vi "Text control 2 v7.0_pump-specific.vi"() -> ()   [LabVIEW 2016]
panel:
  in  "Tab Control":enum32{"Main", "Other parameters"}(tab)
  out "Line running":i32
  out "Total lines":i32
  out "Path":path=path "C:/users/rlp38/09Apr2009LTtesting/test2.txt"
  out "I vs Vg":cluster{"Y data in":dbl[], "X data in":dbl[]}[](graph)
  out "Is max":dbl format="%.2e"
  out "Id max":dbl format="%.2e"
  out "Ig max":dbl format="%.2e"
  out "Imax vs time":cluster{"Y data in":dbl[], "X data in":dbl[]}[](graph)
  out "Imin vs time":cluster{"Y data in":dbl[], "X data in":dbl[]}[](graph)
  out "I vs Vd":cluster{"Y data in":dbl[], "X data in":dbl[]}[](graph)
  in  "Script":string="#-------------------------------------------------------\n# SPM pump cleaning script\n#\n# Version: 0.5\n# Author: Dimitrios Simatos\n# Last updated: 2018-01-05\n#-------------------------------------------------------\n# Description\n#\n# This script is designed to run the cleaning sequence of the SPM OEM pump.\n# This script needs to be run 4 times!\n#-------------------------------------------------------\n# Changes\n#\n# Placed initialization and hard stop commands in the beginning.\n#-------------------------------------------------------\n# Important points\n#\n# Never leave any liquid in the pump to dry after the experiments. If they dry, the residue may block the valve.\n# Always run the cleaning cycle after the experiments.\n# Use clockwise rotation when going up in valve port numbers and vice versa.\n#-------------------------------------------------------\n# Things to do before running the script\n#\n# Set time units to minutes.\n# Set filenames.\n# Replace the tubing, if necessary.\n#-------------------------------------------------------\n# Port connections\n#\n# Port 1: Waste\n# Port 2: Waste\n# Port 3: Various cleaning liquids\n# Port 4: Waste\n# Port 5: Waste\n# Port 6: Waste\n#\n# Between each of the 4 runs, the settings of Port 3 will change, according to the cleaning protocol.\n# The settings for Port 3 are:\n# 1st run: 1% v/v solution of sodium hypochlorite in ultrapure water\n# 2nd run: 0.1% w/v solution of sodium dodecyl sulfate in ultrapure water\n# 3rd run: Ultrapure water\n# 4th run: Waste (in air, not immersed in liquid)\n#-------------------------------------------------------\n# Cleaning protocol for the SPM OEM pump (from the manual)\n#\n# A cleaning procedure should be performed at the end of each day or in between two different experiments.\n# An effective cleaning can be performed in the following manner:\n# • Bleach solution to kill microorganisms\n# 1. Prepare a solution of 1% chlorine bleach and deionized water\n#    NOTE: Prepare a 1% v/v solution of sodium hypochlorite in deionized water\n# 2. Prepare a reservoir and place 1 tubing in the bleach solution and 5 tubings in a waste recipient\n# 3. Pick up the bleach solution through 1 port to entirely fill the syringe\n# 4. Sequentially output the syringe content through the remaining ports and throw it to the waste\n# 5. Repeat operation at least 2 times\n# • Detergent solution to remove debris\n# 1. Prepare a solution of 0.1% detergent and deionized water\n#    NOTE: Prepare a 0.1% w/v solution of sodium dodecyl sulfate in deionized water\n# 2. Move the tubing from the bleach solution reservoir and place it into a reservoir of detergent solution\n# 3. Pick up the detergent solution through 1 port to entirely fill the syringe\n# 4. Sequentially output the detergent solution through the remaining ports into the waste recipient\n# 5. Repeat operation at least 2 times\n# • Rinsing water to prepare the pump for your next experiment\n# 1. Move the tubing from the detergent solution reservoir and place it into a reservoir of deionized water\n# 2. Pick up the rinsing solution through 1 port to entirely fill the syringe\n# 3. Sequentially output the rinse water through the remaining ports into the waste recipient\n# 4. Repeat operation at least 2 times\n# • Replace the tubing, if necessary\n#-------------------------------------------------------\n# Pumping cycles and execution time\n#\n# Execution time for a single cycle: 6 x (1 min + 10 sec) = 7 minutes\n# Total execution time: 4 x 7 = 28 minutes\n# Since the script has to run 4 times, the cleaning lasts for: 4 x 28 = 112 minutes\n# Air must be the last to be pumped through the valve, to remove all liquids.\n# There are 4 pumping cycles. Each one draws a different liquid through port 3 and pumps it sequentially through ports 1,2,4,5,6.\n# During the sequential pumping, each port receives 200 ml of liquid (20% of the total syringe volume = 600 \"plunger units\")\n# The device must be disconnected from the port during the cleaning procedure.\n# All cycles are similar, except cycle 1 has the initialization command uncommented and the first report valve command commented.\n#-------------------------------------------------------\n# Volume of liquid needed\n#\n# Volume of liquid needed per cycle: 1 ml\n# Total volume of liquid needed per script run: 4 x 1 = 4 ml\n# Since the script has to run 4 times, the first 3 with different liquids, I need:\n# 4 ml of 1% v/v solution of sodium hypochlorite in ultrapure water\n# 4 ml of 0.1% w/v solution of sodium dodecyl sulfate in ultrapure water\n# 4 ml of ultrapure water\n#-------------------------------------------------------\n# Parameters\n#\n# Syringe size: 1 ml\n# Step resolution N = 0.01 mm\n# Drawing flow V = 300 pulses/second (6000 ul/min)\n# Pumping flow V = 300 pulses/second (6000 ul/min)\n#-------------------------------------------------------\n# Pump initialization\npump /1T #hard stop pump\npump /1ZR #initialize pump\n#-------------------------------------------------------\n# Cycle 1\n# Fill the syringe\npump /1Q #query pump\npump /1? #report absolute plunger position\n#pump /1?6 #report valve position\nwait-min 1 #wait 1 minute\npump /1N0R #set step resolution: 0.01 mm\npump /1Q #query pump\npump /1? #report absolute plunger position (the plunger should be at 0)\npump /1?6 #report valve position\nwait 1000 #wait 1 second\npump /1V300R #choose speed: 300 steps/s (6000 ul/min)\npump /1Q #query pump\nwait 1000 #wait 1 second\npump /1I3R #go to port 3, clockwise rotation\npump /1Q #query pump\npump /1?6 #report valve position\nwait 1000 #wait 1 second\npump /1A3000R #go to absolute position 3000 (= draw 1 ml)\nwait 30000 #wait 30 seconds\npump /1Q #query pump\npump /1? #report absolute plunger position (the plunger should have finished moving)\n#pump /1?6 #report valve position\n# The sequential pumping begins\n# Port 1\npump /1O1R #switch to port 1, counterclockwise rotation\npump /1Q #query pump\npump /1?6 #report valve position\npump /1A2400R #go to absolute position 2400 (= pump 200 ul)\npump /1Q #query pump\npump /1? #report absolute plunger position (the plunger should be moving to 0)\nwait-min 1 #wait 1 minute\npump /1? #report absolute plunger position (the plunger should have finished moving)\n# Port 2\npump /1I2R #switch to port 2, clockwise rotation\npump /1Q #query pump\npump /1?6 #report valve position\npump /1A1800R #go to absolute position 1800 (= pump 200 ul)\npump /1Q #query pump\npump /1? #report absolute plunger position (the plunger should be moving to 0)\nwait-min 1 #wait 1 minute\npump /1? #report absolute plunger position (the plunger should have finished moving)\n# Port 4\npump /1I4R #switch to port 4, clockwise rotation\npump /1Q #query pump\npump /1?6 #report valve position\npump /1A1200R #go to absolute position 1200 (= pump 200 ul)\npump /1Q #query pump\npump /1? #report absolute plunger position (the plunger should be moving to 0)\nwait-min 1 #wait 1 minute\npump /1? #report absolute plunger position (the plunger should have finished moving)\n# Port 5\npump /1I5R #switch to port 5, clockwise rotation\npump /1Q #query pump\npump /1?6 #report valve position\npump /1A600R #go to absolute position 600 (= pump 200 ul)\npump /1Q #query pump\npump /1? #report absolute plunger position (the plunger should be moving to 0)\nwait-min 1 #wait 1 minute\npump /1? #report absolute plunger position (the plunger should have finished moving)\n# Port 6\npump /1I6R #switch to port 6, clockwise rotation\npump /1Q #query pump\npump /1?6 #report valve position\npump /1A0R #go to absolute position 0 (= pump 200 ul)\npump /1Q #query pump\npump /1? #report absolute plunger position (the plunger should be moving to 0)\nwait-min 1 #wait 1 minute\npump /1? #report absolute plunger position (the plunger should have finished moving)\n#-------------------------------------------------------\n# Cycle 2\n# Fill the syringe\n#pump /1ZR #initialize pump\npump /1Q #query pump\npump /1? #report absolute plunger position\npump /1?6 #report valve position\nwait-min 1 #wait 1 minute\npump /1N0R #set step resolution: 0.01 mm\npump /1Q #query pump\npump /1? #report absolute plunger position (the plunger should be at 0)\npump /1?6 #report valve position\nwait 1000 #wait 1 second\npump /1V300R #choose speed: 300 steps/s (6000 ul/min)\npump /1Q #query pump\nwait 1000 #wait 1 second\npump /1O3R #go to port 3, counterclockwise rotation\npump /1Q #query pump\npump /1?6 #report valve position\nwait 1000 #wait 1 second\npump /1A3000R #go to absolute position 3000 (= draw 1 ml)\nwait 30000 #wait 30 seconds\npump /1Q #query pump\npump /1? #report absolute plunger position (the plunger should have finished moving)\n#pump /1?6 #report valve position\n# The sequential pumping begins\n# Port 1\npump /1O1R #switch to port 1, counterclockwise rotation\npump /1Q #query pump\npump /1?6 #report valve position\npump /1A2400R #go to absolute position 2400 (= pump 200 ul)\npump /1Q #query pump\npump /1? #report absolute plunger position (the plunger should be moving to 0)\nwait-min 1 #wait 1 minute\npump /1? #report absolute plunger position (the plunger should have finished moving)\n# Port 2\npump /1I2R #switch to port 2, clockwise rotation\npump /1Q #query pump\npump /1?6 #report valve position\npump /1A1800R #go to absolute position 1800 (= pump 200 ul)\npump /1Q #query pump\npump /1? #report absolute plunger position (the plunger should be moving to 0)\nwait-min 1 #wait 1 minute\npump /1? #report absolute plunger position (the plunger should have finished moving)\n# Port 4\npump /1I4R #switch to port 4, clockwise rotation\npump /1Q #query pump\npump /1?6 #report valve position\npump /1A1200R #go to absolute position 1200 (= pump 200 ul)\npump /1Q #query pump\npump /1? #report absolute plunger position (the plunger should be moving to 0)\nwait-min 1 #wait 1 minute\npump /1? #report absolute plunger position (the plunger should have finished moving)\n# Port 5\npump /1I5R #switch to port 5, clockwise rotation\npump /1Q #query pump\npump /1?6 #report valve position\npump /1A600R #go to absolute position 600 (= pump 200 ul)\npump /1Q #query pump\npump /1? #report absolute plunger position (the plunger should be moving to 0)\nwait-min 1 #wait 1 minute\npump /1? #report absolute plunger position (the plunger should have finished moving)\n# Port 6\npump /1I6R #switch to port 6, clockwise rotation\npump /1Q #query pump\npump /1?6 #report valve position\npump /1A0R #go to absolute position 0 (= pump 200 ul)\npump /1Q #query pump\npump /1? #report absolute plunger position (the plunger should be moving to 0)\nwait-min 1 #wait 1 minute\npump /1? #report absolute plunger position (the plunger should have finished moving)\n#-------------------------------------------------------\n# Cycle 3\n# Fill the syringe\n#pump /1ZR #initialize pump\npump /1Q #query pump\npump /1? #report absolute plunger position\npump /1?6 #report valve position\nwait-min 1 #wait 1 minute\npump /1N0R #set step resolution: 0.01 mm\npump /1Q #query pump\npump /1? #report absolute plunger position (the plunger should be at 0)\npump /1?6 #report valve position\nwait 1000 #wait 1 second\npump /1V300R #choose speed: 300 steps/s (6000 ul/min)\npump /1Q #query pump\nwait 1000 #wait 1 second\npump /1O3R #go to port 3, counterclockwise rotation\npump /1Q #query pump\npump /1?6 #report valve position\nwait 1000 #wait 1 second\npump /1A3000R #go to absolute position 3000 (= draw 1 ml)\nwait 30000 #wait 30 seconds\npump /1Q #query pump\npump /1? #report absolute plunger position (the plunger should have finished moving)\n#pump /1?6 #report valve position\n# The sequential pumping begins\n# Port 1\npump /1O1R #switch to port 1, counterclockwise rotation\npump /1Q #query pump\npump /1?6 #report valve position\npump /1A2400R #go to absolute position 2400 (= pump 200 ul)\npump /1Q #query pump\npump /1? #report absolute plunger position (the plunger should be moving to 0)\nwait-min 1 #wait 1 minute\npump /1? #report absolute plunger position (the plunger should have finished moving)\n# Port 2\npump /1I2R #switch to port 2, clockwise rotation\npump /1Q #query pump\npump /1?6 #report valve position\npump /1A1800R #go to absolute position 1800 (= pump 200 ul)\npump /1Q #query pump\npump /1? #report absolute plunger position (the plunger should be moving to 0)\nwait-min 1 #wait 1 minute\npump /1? #report absolute plunger position (the plunger should have finished moving)\n# Port 4\npump /1I4R #switch to port 4, clockwise rotation\npump /1Q #query pump\npump /1?6 #report valve position\npump /1A1200R #go to absolute position 1200 (= pump 200 ul)\npump /1Q #query pump\npump /1? #report absolute plunger position (the plunger should be moving to 0)\nwait-min 1 #wait 1 minute\npump /1? #report absolute plunger position (the plunger should have finished moving)\n# Port 5\npump /1I5R #switch to port 5, clockwise rotation\npump /1Q #query pump\npump /1?6 #report valve position\npump /1A600R #go to absolute position 600 (= pump 200 ul)\npump /1Q #query pump\npump /1? #report absolute plunger position (the plunger should be moving to 0)\nwait-min 1 #wait 1 minute\npump /1? #report absolute plunger position (the plunger should have finished moving)\n# Port 6\npump /1I6R #switch to port 6, clockwise rotation\npump /1Q #query pump\npump /1?6 #report valve position\npump /1A0R #go to absolute position 0 (= pump 200 ul)\npump /1Q #query pump\npump /1? #report absolute plunger position (the plunger should be moving to 0)\nwait-min 1 #wait 1 minute\npump /1? #report absolute plunger position (the plunger should have finished moving)\n#-------------------------------------------------------\n# Cycle 4\n# Fill the syringe\n#pump /1ZR #initialize pump\npump /1Q #query pump\npump /1? #report absolute plunger position\npump /1?6 #report valve position\nwait-min 1 #wait 1 minute\npump /1N0R #set step resolution: 0.01 mm\npump /1Q #query pump\npump /1? #report absolute plunger position (the plunger should be at 0)\npump /1?6 #report valve position\nwait 1000 #wait 1 second\npump /1V300R #choose speed: 300 steps/s (6000 ul/min)\npump /1Q #query pump\nwait 1000 #wait 1 second\npump /1O3R #go to port 3, counterclockwise rotation\npump /1Q #query pump\npump /1?6 #report valve position\nwait 1000 #wait 1 second\npump /1A3000R #go to absolute position 3000 (= draw 1 ml)\nwait 30000 #wait 30 seconds\npump /1Q #query pump\npump /1? #report absolute plunger position (the plunger should have finished moving)\n#pump /1?6 #report valve position\n# The sequential pumping begins\n# Port 1\npump /1O1R #switch to port 1, counterclockwise rotation\npump /1Q #query pump\npump /1?6 #report valve position\npump /1A2400R #go to absolute position 2400 (= pump 200 ul)\npump /1Q #query pump\npump /1? #report absolute plunger position (the plunger should be moving to 0)\nwait-min 1 #wait 1 minute\npump /1? #report absolute plunger position (the plunger should have finished moving)\n# Port 2\npump /1I2R #switch to port 2, clockwise rotation\npump /1Q #query pump\npump /1?6 #report valve position\npump /1A1800R #go to absolute position 1800 (= pump 200 ul)\npump /1Q #query pump\npump /1? #report absolute plunger position (the plunger should be moving to 0)\nwait-min 1 #wait 1 minute\npump /1? #report absolute plunger position (the plunger should have finished moving)\n# Port 4\npump /1I4R #switch to port 4, clockwise rotation\npump /1Q #query pump\npump /1?6 #report valve position\npump /1A1200R #go to absolute position 1200 (= pump 200 ul)\npump /1Q #query pump\npump /1? #report absolute plunger position (the plunger should be moving to 0)\nwait-min 1 #wait 1 minute\npump /1? #report absolute plunger position (the plunger should have finished moving)\n# Port 5\npump /1I5R #switch to port 5, clockwise rotation\npump /1Q #query pump\npump /1?6 #report valve position\npump /1A600R #go to absolute position 600 (= pump 200 ul)\npump /1Q #query pump\npump /1? #report absolute plunger position (the plunger should be moving to 0)\nwait-min 1 #wait 1 minute\npump /1? #report absolute plunger position (the plunger should have finished moving)\n# Port 6\npump /1I6R #switch to port 6, clockwise rotation\npump /1Q #query pump\npump /1?6 #report valve position\npump /1A0R #go to absolute position 0 (= pump 200 ul)\npump /1Q #query pump\npump /1? #report absolute plunger position (the plunger should be moving to 0)\nwait-min 1 #wait 1 minute\npump /1? #report absolute plunger position (the plunger should have finished moving)\n#-------------------------------------------------------"
  out "Command running:":string
  out "Serial port data":string
  out "Elapsed Time":dbl caption="Elapsed Time (s)"
  in  "Time Units":u16(ring)=1 items=["Seconds", "Minutes", "Hours"]
  in  "Time Offset":dbl caption="Set Start Time (s)"
  in  "Reset":bool
  in  "Auto Reset":bool
  in  "integration time":u32(slide) max=2 step=1 scale=0.0..2.0
  in  "Interrupt scan":bool
  out "Absolute plunger position vs time":cluster{"Y data in":dbl[], "X data in":dbl[]}[](graph)
  out "Valve position vs time":cluster{"Y data in":dbl[], "X data in":dbl[]}[](graph)
  out "Is on":dbl format="%.2e"
  out "Id on":dbl format="%.2e"
  out "Ig on":dbl format="%.2e"
  out "Ion vs time":cluster{"Y data in":dbl[], "X data in":dbl[]}[](graph)
  out "Ioff vs time":cluster{"Y data in":dbl[], "X data in":dbl[]}[](graph)
  out "Ig min":dbl format="%.2e"
  out "Id min":dbl format="%.2e"
  out "Is min":dbl format="%.2e"
  out "Is off":dbl format="%.2e"
  out "Id off":dbl format="%.2e"
  out "Ig off":dbl format="%.2e"
  in  "Integration time (long)":dbl=0.32 min=0.04 max=2.0 step=0.02 format="%.2f"
  in  "Integration time (short)":dbl=0.0019 min=8e-05 max=0.0019 step=8e-05 format="%^.0e"
  in  "Gate: Compliance":dbl=0.001 format="%.8f"
  in  "Drain: Compliance":dbl=0.001 format="%.8f"
  in  "Hard stop pump":bool
  in  "Halt pump":bool
  in  "Interrupt program":bool
  in  "Suffix (script)":string="step_1_up-H2O_initial_script.txt"
  in  "Filename (variable part)":string="step_1_up-H2O_initial_"
  in  "Plot output curve extrema vs time":bool
  in  "Plot transfer curve extrema vs time":bool=TRUE
  in  "Plot sample extrema vs time":bool
  out "I vs time (Bias Stress)":cluster{"Y data in":dbl[], "X data in":dbl[]}[](graph)
  in  "Sample I - Probe 4 (Disabled)":u32(ring)=3 items=["SMU1  ", "SMU2  ", "SMU3  ", "SMU4  ", "SMU5  ", "SMU6  "]
  in  "Sample I - Source/Common":u32(ring) items=["SMU1  ", "SMU2  ", "SMU3  ", "SMU4  ", "SMU5  ", "SMU6  "]
  in  "Sample I - Probe 3 (Disabled)":u32(ring)=2 items=["SMU1  ", "SMU2  ", "SMU3  ", "SMU4  ", "SMU5  ", "SMU6  "]
  in  "Sample I - Drain/Gate":u32(ring)=1 items=["SMU1  ", "SMU2  ", "SMU3  ", "SMU4  ", "SMU5  ", "SMU6  "]
  in  "Sample - Probe 4":u32(ring)=3 items=["SMU1  ", "SMU2  ", "SMU3  ", "SMU4  ", "SMU5  ", "SMU6  "]
  in  "Sample - Source/Common":u32(ring) items=["SMU1  ", "SMU2  ", "SMU3  ", "SMU4  ", "SMU5  ", "SMU6  "]
  in  "Sample - Gate":u32(ring)=2 items=["SMU1  ", "SMU2  ", "SMU3  ", "SMU4  ", "SMU5  ", "SMU6  "]
  in  "Sample - Drain":u32(ring)=1 items=["SMU1  ", "SMU2  ", "SMU3  ", "SMU4  ", "SMU5  ", "SMU6  "]
  in  "VSU2 Stress - Source/Common":u32(ring) items=["SMU1  ", "SMU2  ", "SMU3  ", "SMU4  ", "SMU5  ", "SMU6  "]
  in  "Stress I - Source/Common":u32(ring) items=["SMU1  ", "SMU2  ", "SMU3  ", "SMU4  ", "SMU5  ", "SMU6  "]
  in  "Stress I - Drain/Gate":u32(ring)=1 items=["SMU1  ", "SMU2  ", "SMU3  ", "SMU4  ", "SMU5  ", "SMU6  "]
  in  "Stress V - Source/Common":u32(ring) items=["SMU1  ", "SMU2  ", "SMU3  ", "SMU4  ", "SMU5  ", "SMU6  "]
  in  "Stress V - Gate":u32(ring)=2 items=["SMU1  ", "SMU2  ", "SMU3  ", "SMU4  ", "SMU5  ", "SMU6  "]
  in  "Stress V - Drain":u32(ring)=1 items=["SMU1  ", "SMU2  ", "SMU3  ", "SMU4  ", "SMU5  ", "SMU6  "]
  in  "FPP - Source":u32(ring) items=["VSU1  ", "VSU2  "]
  in  "FPP - Probe 2":u32(ring)=3 items=["SMU1  ", "SMU2  ", "SMU3  ", "SMU4  ", "SMU5  ", "SMU6  "]
  in  "FPP - Probe 1":u32(ring) items=["SMU1  ", "SMU2  ", "SMU3  ", "SMU4  ", "SMU5  ", "SMU6  "]
  in  "FPP - Gate":u32(ring)=2 items=["SMU1  ", "SMU2  ", "SMU3  ", "SMU4  ", "SMU5  ", "SMU6  "]
  in  "FPP - Drain":u32(ring)=1 items=["SMU1  ", "SMU2  ", "SMU3  ", "SMU4  ", "SMU5  ", "SMU6  "]
  in  "Pulsed Stress V - Vextra":u32(ring)=1 items=["VSU1  ", "VSU2  "]
  in  "Pulsed Stress V - Probe 4":u32(ring)=3 items=["SMU1  ", "SMU2  ", "SMU3  ", "SMU4  ", "SMU5  ", "SMU6  "]
  in  "Pulsed Stress V - Source/Common":u32(ring) items=["SMU1  ", "SMU2  ", "SMU3  ", "SMU4  ", "SMU5  ", "SMU6  "]
  in  "Pulsed Stress V - Gate":u32(ring)=2 items=["SMU1  ", "SMU2  ", "SMU3  ", "SMU4  ", "SMU5  ", "SMU6  "]
  in  "Pulsed Stress V - Drain":u32(ring)=1 items=["SMU1  ", "SMU2  ", "SMU3  ", "SMU4  ", "SMU5  ", "SMU6  "]
  in  "Transfer/Output - Probe 4":u32(ring)=3 items=["SMU1  ", "SMU2  ", "SMU3  ", "SMU4  ", "SMU5  ", "SMU6  "]
  in  "Transfer/Output - Source/Common":u32(ring) items=["SMU1  ", "SMU2  ", "SMU3  ", "SMU4  ", "SMU5  ", "SMU6  "]
  in  "Transfer/Output - Gate":u32(ring)=2 items=["SMU1  ", "SMU2  ", "SMU3  ", "SMU4  ", "SMU5  ", "SMU6  "]
  in  "Transfer/Output - Drain":u32(ring)=1 items=["SMU1  ", "SMU2  ", "SMU3  ", "SMU4  ", "SMU5  ", "SMU6  "]
  in  "Gate Range\nmode":u16(ring) items=["Auto", "Limited", "Fixed"]
  in  "Gate Range":u8(slide)=3 max=11 scale=0.0..11.0
  in  "Source/Drain\nRange mode":u16(ring) items=["Auto", "Limited", "Fixed"]
  in  "Source/Drain Range":u8(slide)=3 max=11 scale=0.0..11.0
  in  "Panel Controls":T1={"Emergency Stop"=refnum, "TransGraph Max"=1e-05, "Text/Graph (text=false)"=TRUE} {"TransGraph Max" format="%.2e"}
  in  "Panel Controls 2":T2={"Emergency Stop"=refnum, "TransGraph Max"=1e-05, "Text/Graph (text=false)"=TRUE, "TransGraph Min"=1e-11} {"TransGraph Min" format="%.2e"; "TransGraph Max" format="%.2e"}
  in  "Probe 4":cluster{"on/off":bool, "Voltage":dbl} {"Voltage" min=-100.0 max=100.0 format="%.2f"}
  in  "Full Reset":bool
  in  "Standby":T3
  out "error out":errorcluster
  in  "Delay before read (ms)":u32=1000
  in  "byte count":u32=64
  in  "Serial End Mode for Reads":u16(ring)=2 items=["None", "LastBit", "TermChar"]
  in  "Timeout (ms)":u32=10000
  in  "Enable Termination\nChar (T)":bool=TRUE
  in  "Termination char\n(0xA = '\\n' = LF)\n(0xD = '\\r' = CR)":u8=13 format="%.0x"
  in  "flow control":u16(ring) items=["None"=0, "XON/XOFF"=1, "RTS/CTS"=2, "DTR/DSR"=4]
  in  "stop bits":u16(ring)=10 items=["1.0"=10, "1.5"=15, "2.0"=20]
  in  "parity":u16(ring) items=["None", "Odd", "Even", "Mark", "Space"]
  in  "data bits":u16=8 min=5 max=8 step=1
  in  "VISA resource name":refnum<visa-resource-name>="COM6"
  in  "baud rate":u32=9600
  out "Timings Indicator":T4 {"integration time" scale=0.0..2.0}
  in  "Timings (overwritten by the Front Panel)":T5={"integration time"=0, "Short/Long integration time"=0.00064, "hold time (sec)"=0.0, "delay time (sec)"=0.0, "Step Time (0 disables)"=0.0, "sweep method"=0, "Pulse period"=0.005, "Base voltage"=0.0, "Pulse width"=0.0005} {"Pulse width" min=0.0005 max=0.1 step=0.0001 format="%.4f"; "Base voltage" format="%^.4e"; "Pulse period" min=0.005 max=1.0 step=0.0001 format="%.4f"; "sweep method" items=["Continuous", "Pulsed"]; "Step Time (0 disables)" format="%.2f"; "delay time (sec)" format="%.4f"; "hold time (sec)" format="%.4f"; "Short/Long integration time" format="%^.0e"; "integration time" scale=0.0..2.0}
  out "Probe 4 Indicator":cluster{"on/off":bool, "Voltage":dbl} {"Voltage" min=-100.0 max=100.0 format="%.2f"}
  in  "VISA resource name in":refnum<visa-resource-name>="GPIB0::14::INSTR"
  in  "Gate":T6={"Gate Start"=0.0, "Gate Stop"=2.0, "Gate Step (linear only)"=1.0, "Gate Compliance"=0.0001, "Gate PComp"=0.0, "Range mode"=0, "Range"=6} {"Range" max=11 scale=0.0..11.0; "Range mode" items=["Auto", "Limited", "Fixed"]; "Gate PComp" format="%^.2e"; "Gate Compliance" format="%^.2e"; "Gate Step (linear only)" format="%^.4e"; "Gate Stop" format="%^.4e"; "Gate Start" format="%^.4e"}
  in  "Drain 2":T7={"Drain Start"=0.0, "Drain Stop"=2.0, "Drain Compliance"=0.0001, "Drain Step"=1.0, "Drain PComp"=0.0, "Range mode"=0, "Range"=6} {"Range" max=11 scale=0.0..11.0; "Range mode" items=["Auto", "Limited", "Fixed"]; "Drain PComp" format="%^.2e"; "Drain Step" format="%^.4e"; "Drain Compliance" format="%^.2e"; "Drain Stop" format="%^.4e"; "Drain Start" format="%^.4e"}
  # "Syntax:\nitime [s|m|l] time(sec): [s|m|l] determines the integration time setting (small|medium|long) and time sets the value.\nNOTE: The value of the integration time has to be within the range allowed by its category (s|m|l), otherwise, the closest value will be used. (e.g. if the category is set to short but the time value is very long, the actual value used will be the maximum short integration time.\nIntegration times:\n    Short: Default: 640 us. Range: 8E-5 - 1.92E-3 seconds.\n    Medium: Fixed at 1 NPL cycle (0.02 seconds).\n    Long: Default: 16 NPL cycles (0.32 seconds). Range: 2-100 NPL cycles (0.04 seconds - 2 seconds).\ngaterangemode [a|l|f]\ndrainrangemode [a|l|f]\npulsed [on|off] PulsePeriod(sec) PulseBaseVoltage PulseONWidth(sec)\nstandby [on l off]\nwait NumMilliseconds\nwait-min NumMinutes\n# texthere = comment\nProbe4 [ON|OFF] Voltage\ntransfer [s|d] VgStart VgStop VgStep VdStart VdStop VdStep\noutput [s|d] VgStart VgStop VgStep VdStart VdStop VdStep\nsample Vg Vd NumSamples Time(s) SampleInterval(s)\nsamplei Idg NumSamples Time(s) SampleInterval(s) VDGcompliance\n100 samples is approximately 13 seconds with medium integration\n# If in doubt use SampleInterval(s) = 0.004\n    NOTE: When doing bias stress measurements, it is best to set the Time Units to \"Seconds\", as the \"sample\" command has been configured to give the output to seconds.\nstressV VG VD IGcompliance IDcompliance Duration(sec)\nstressI IDG VDGcompliance Duration(sec)\nvsu2pulse Bias Duration(s)\npulsedstressV [s|d] VEstop VgON VgOFF Period(s) PulseONwidth(s) Vd\nsample-fpp Vg Vd NumSamples Time\nresample-fpp Vg Vd\ntransfer-fpp [s|d] VgStart VgStop VgStep VdStart VdStop VdStep\noutput-fpp [s|d] VgStart VgStop VgStep VdStart VdStop VdStep\nserial SerialPortCommand\npump SerialPortCommand for the SPM pump\n\nSPM Pump Syntax (<x>: pump number, use 1 if only one pump):\nif the command syntax contains [R], then append the letter R to the command\n/<x>Q: query (a query command should follow each command)\n/<x>Z[R] or /<x>Y[R]: initialize pump\n/<x>N<n>[R] (<n>=0,1): <0> (<1>) microstep 0.01 mm (0.00125 mm) resolution\n/<x>I<n> (<n>=0-6): turn to port number n (clockwise)\n/<x>O<n> (<n>=0-6): turn to port number n (counterclockwise)\n/<x>X: Re-execute last command string\n/<x>G<n>[R] (<n>=0-60000): repeat command sequence (default: 0, 0=loop forever)\n/<x>g: Mark the start of a repeat sequence (max = 10)\n/<x>M<n>[R] (<n>=0-86400000): delay command execution by n milliseconds\n/<x>H: Halt; Pause the sequence after finishing the current move\n/<x>T: Hardstop; Interrupt the current move and suppress it from the sequence\n/<x>A<n>[R] (<n>=0-3000 with N=0, 0-24000 with N=1): absolute position\n/<x>P<n>[R] (<n>=0-3000 with N=0, 0-24000 with N=1): relative pickup\n/<x>D<n>[R] (<n>=0-3000 with N=0, 0-24000 with N=1): relative dispense\n/<x>V<n>[R] (<n>=1-1600 default: 150): set peak speed (pulses/sec)\nNOTE: The lowest speed limit is 1 pulse/sec, not 5, as the manual states.\n/<x>S<n>[R] (<n>=10-40 default: 22): set speed (NOT in pulses/sec, look in manual)\nNOTE: When controlled with absolute position, one does not need to pay special attention to the syringe that is mounted on the pump.\nWithdraw from lower stage (ports 3, 5), dispense from higher stage (ports 2, 4, 6).\nConnect Port 1 to waste."
  # "Time"
  # "1\n2\n3\n4\n5\n6\n7\n8\n9\n10\n11\n12\n13\n14\n15\n16\n17\n18\n19\n20"
  # "Serial port settings"
  # "SMUs"
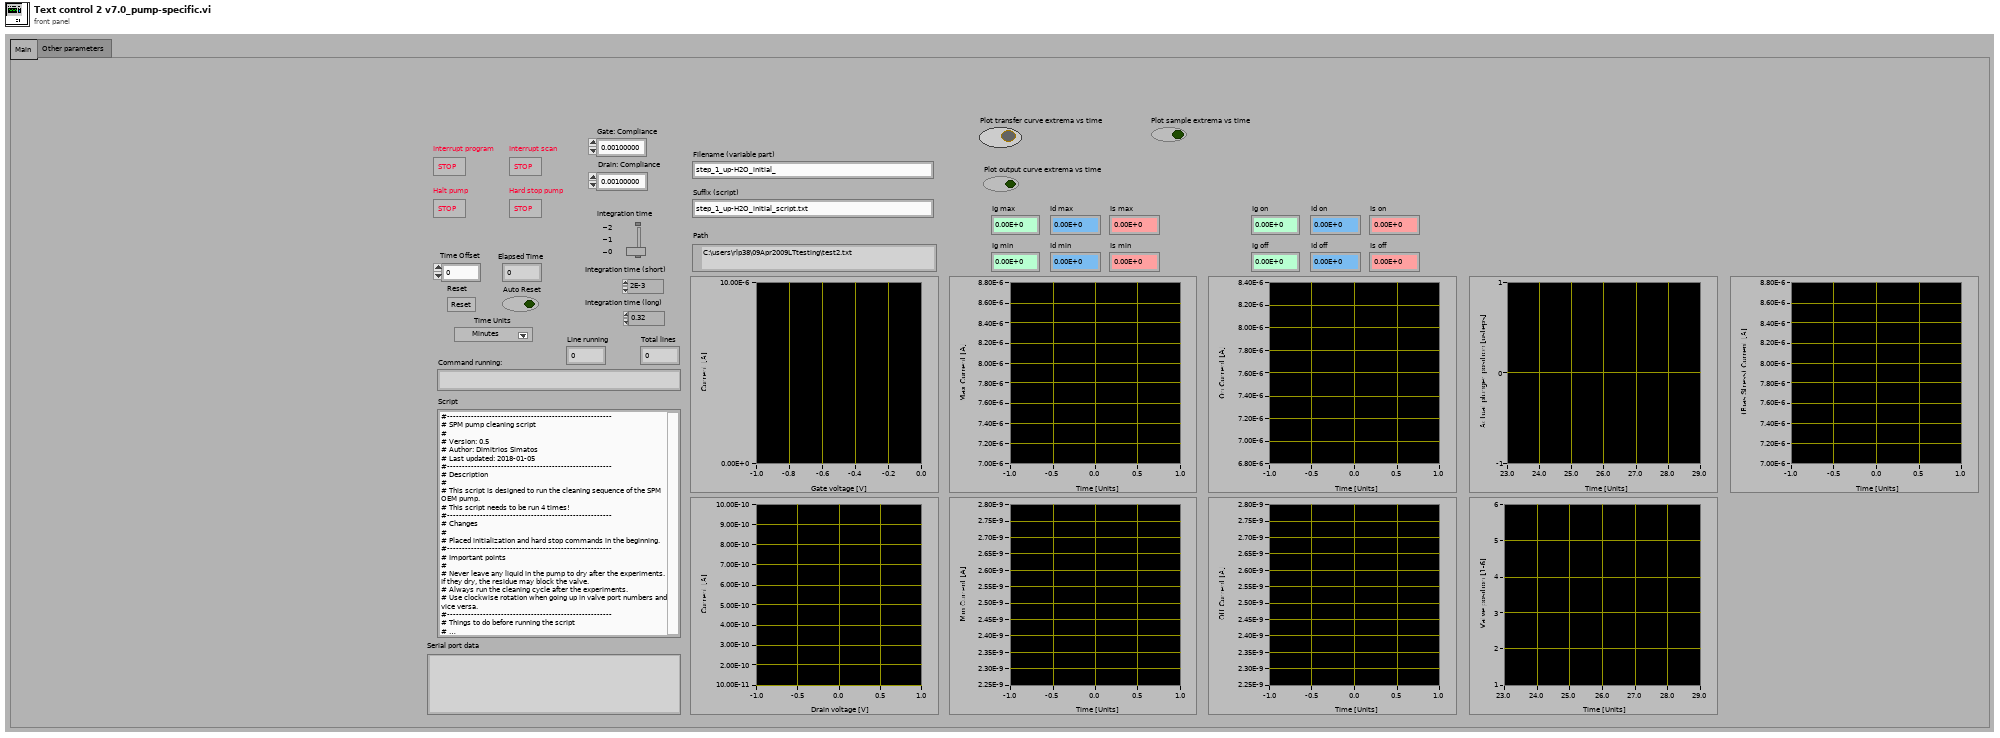
[diagram p1: front panel]
types:
  T1 = cluster{"Emergency Stop":refnum<vi>, "TransGraph Max":dbl, "Text/Graph (text=false)":bool}
  T2 = cluster{"Emergency Stop":refnum<vi>, "TransGraph Max":dbl, "Text/Graph (text=false)":bool, "TransGraph Min":dbl}
  T3 = cluster{"Gate Standby":bool, "Drain Standby":bool}
  T4 = cluster{"Short/Long integration time":dbl, "hold time (sec)":dbl, "delay time (sec)":dbl, "Step Time (0 disables)":dbl, "sweep method":u16, "Pulse period":dbl, "Base voltage":dbl, "Pulse width":dbl, "integration time":u32}
  T5 = cluster{"integration time":u32, "Short/Long integration time":dbl, "hold time (sec)":dbl, "delay time (sec)":dbl, "Step Time (0 disables)":dbl, "sweep method":u16, "Pulse period":dbl, "Base voltage":dbl, "Pulse width":dbl}
  T6 = cluster{"Gate Start":dbl, "Gate Stop":dbl, "Gate Step (linear only)":dbl, "Gate Compliance":dbl, "Gate PComp":dbl, "Range mode":u16, "Range":u8}
  T7 = cluster{"Drain Start":dbl, "Drain Stop":dbl, "Drain Compliance":dbl, "Drain Step":dbl, "Drain PComp":dbl, "Range mode":u16, "Range":u8}
  T8 = enum16{"open", "replace", "create", "open or create", "replace or create", "replace or create with confirmation"}
  T9 = cluster{"V2 Start":dbl, "V2 Step":dbl, "Number of points":i32}
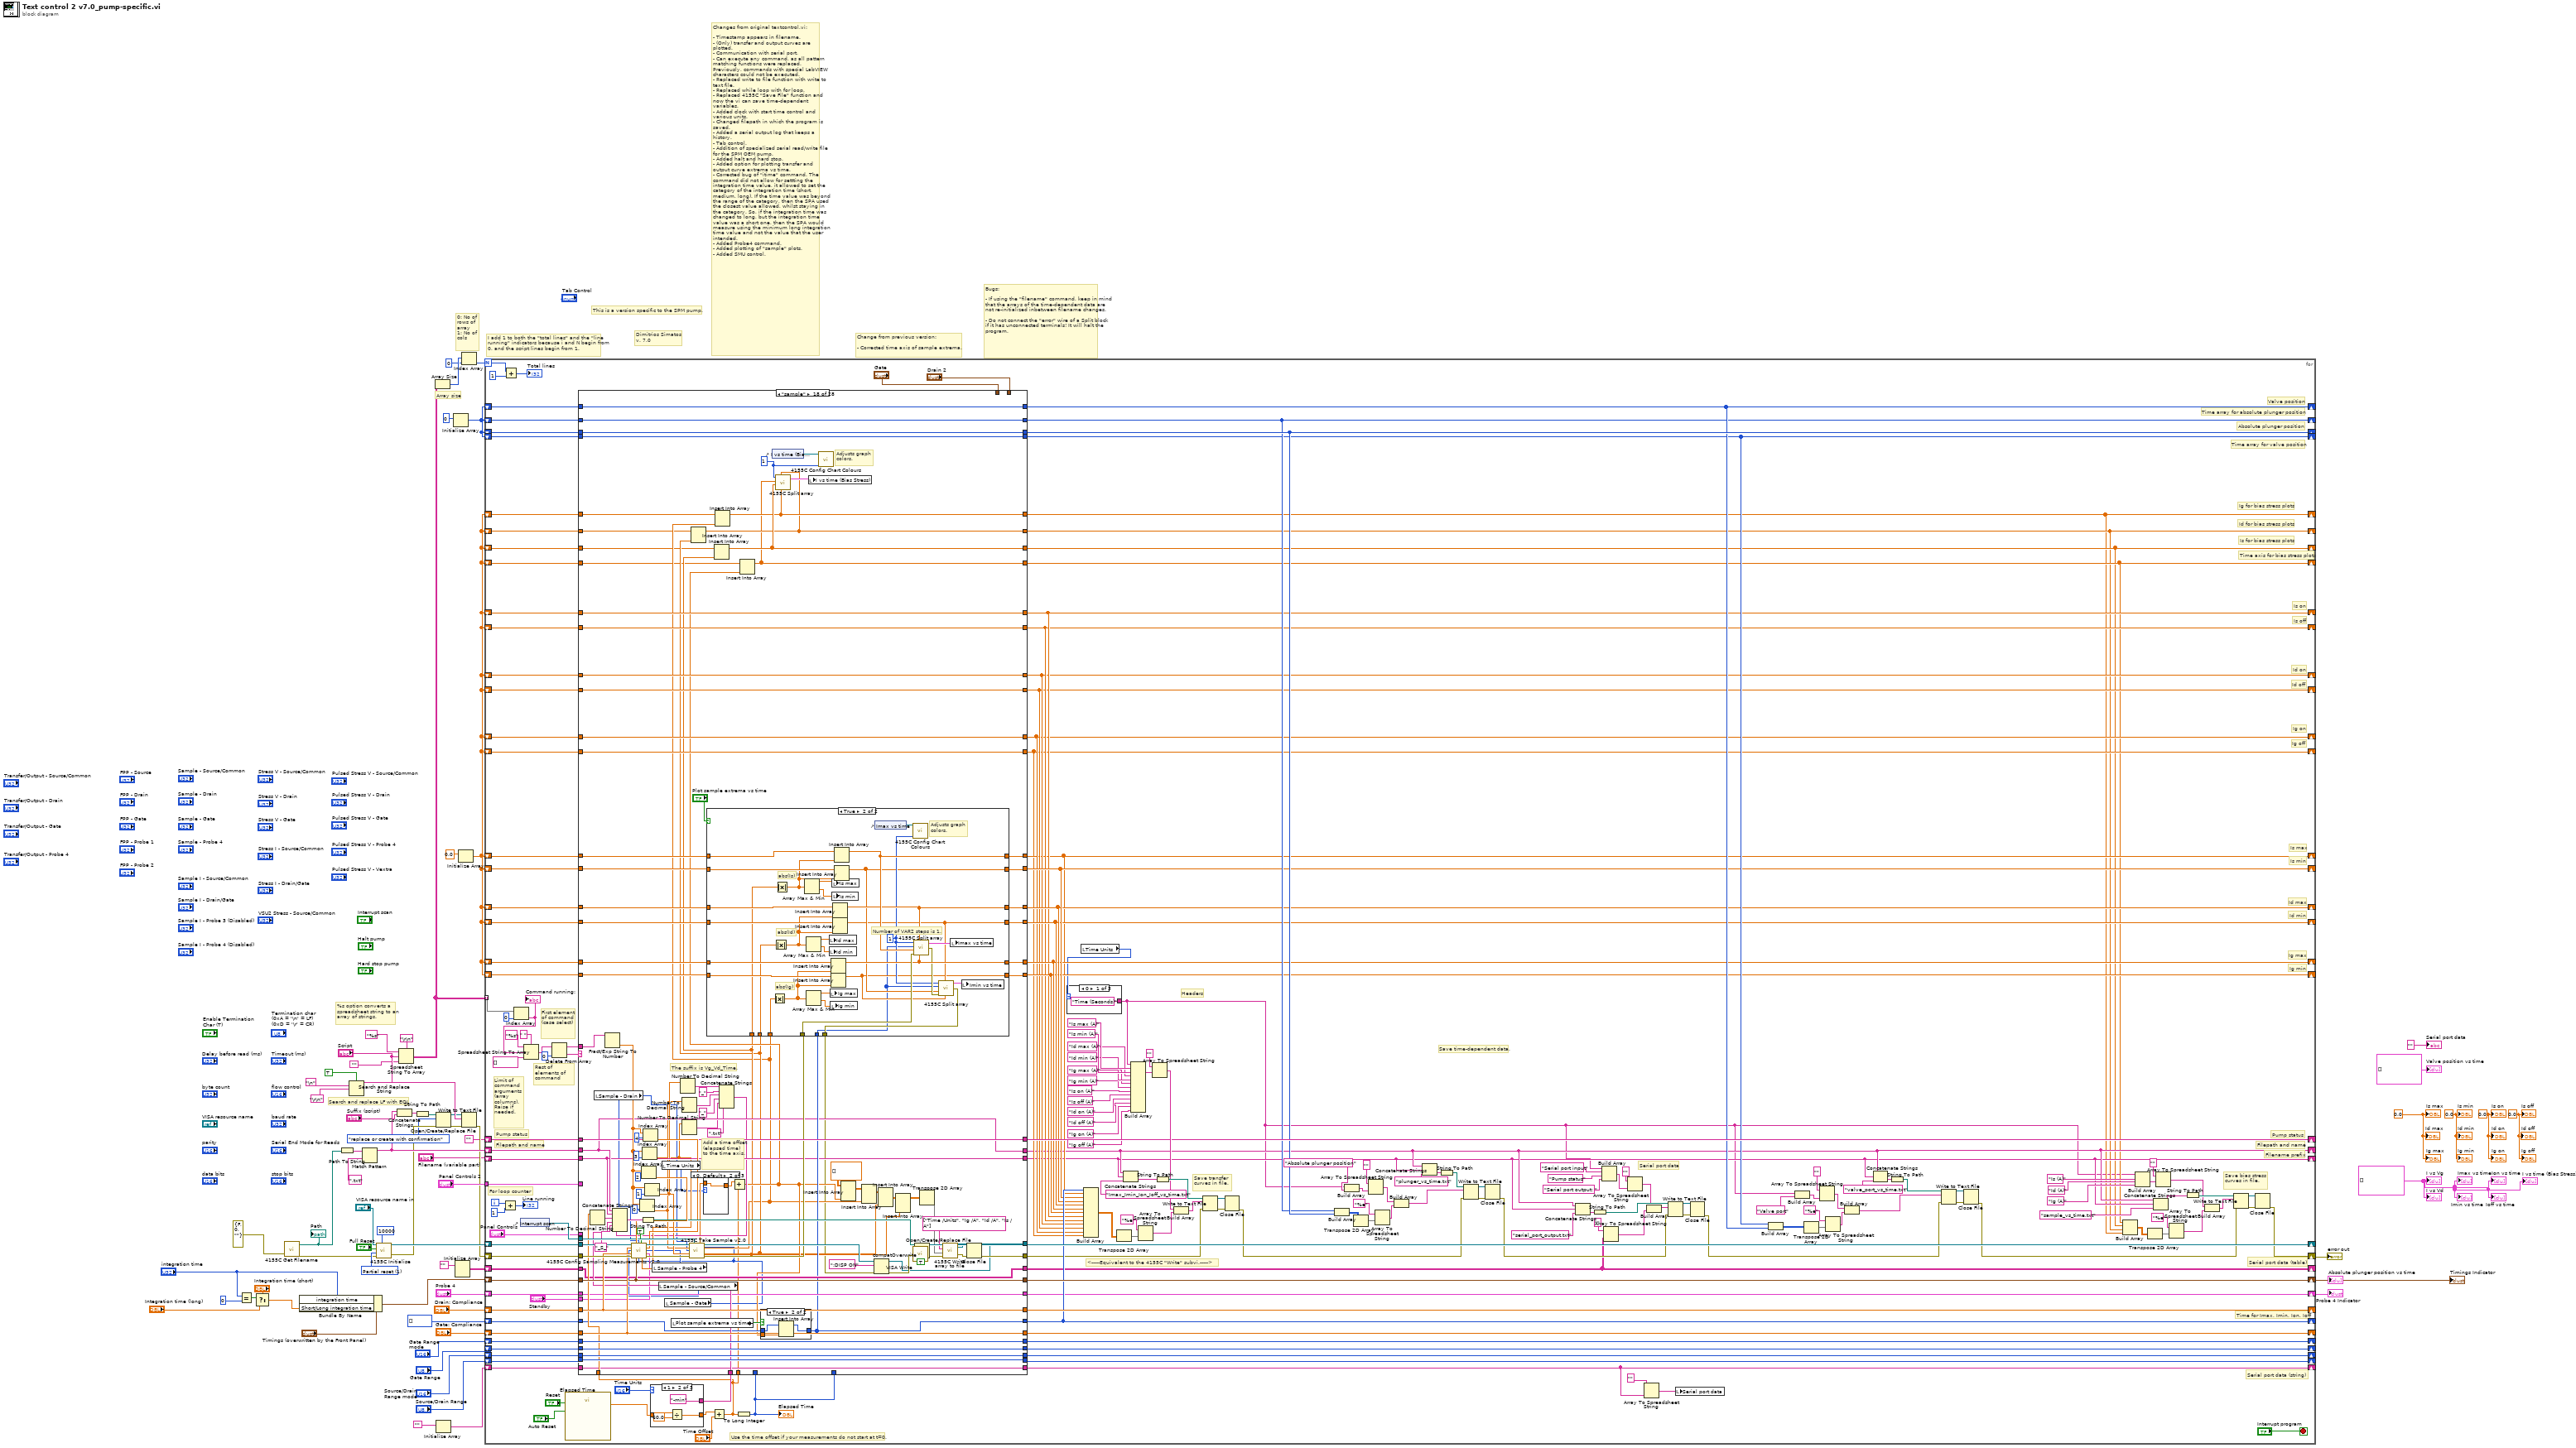
[diagram p0: block diagram]
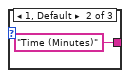
[diagram p2: hidden frame]
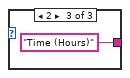
[diagram p3: hidden frame]
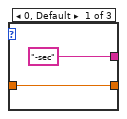
[diagram p4: hidden frame]
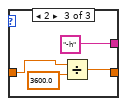
[diagram p5: hidden frame]
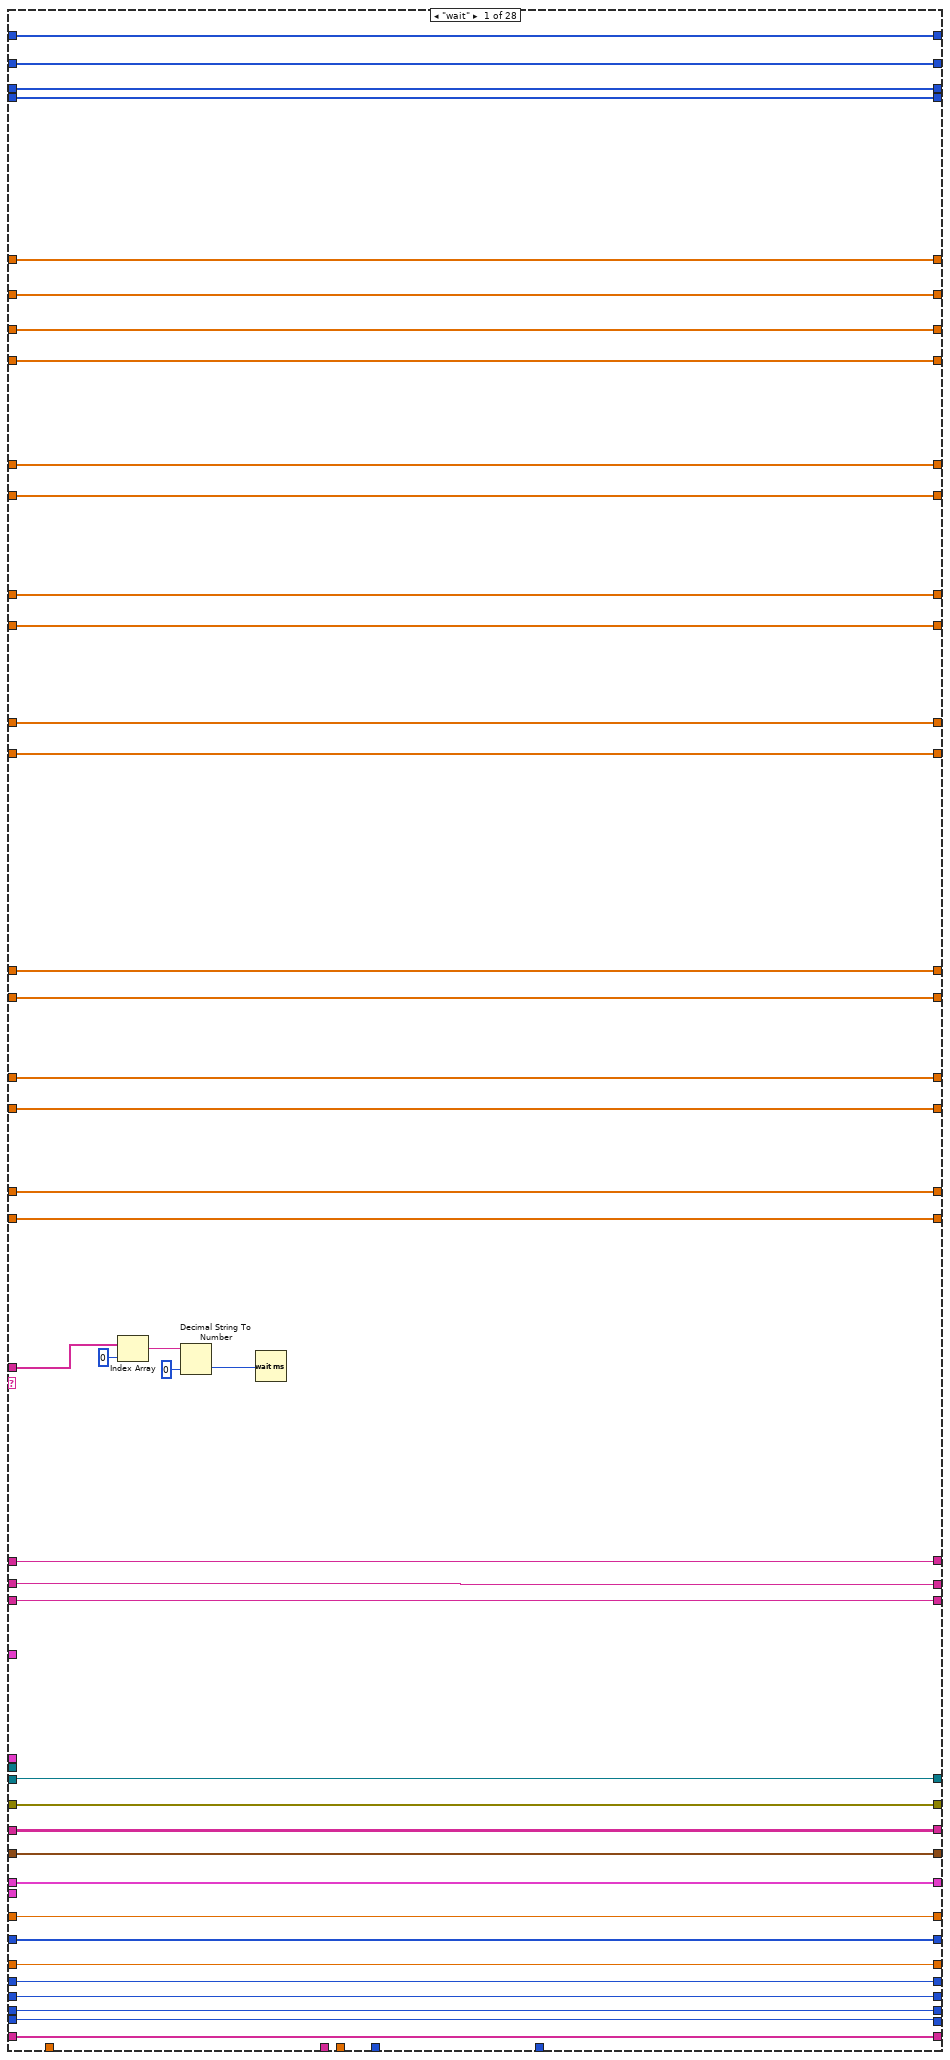
[diagram p6: hidden frame]
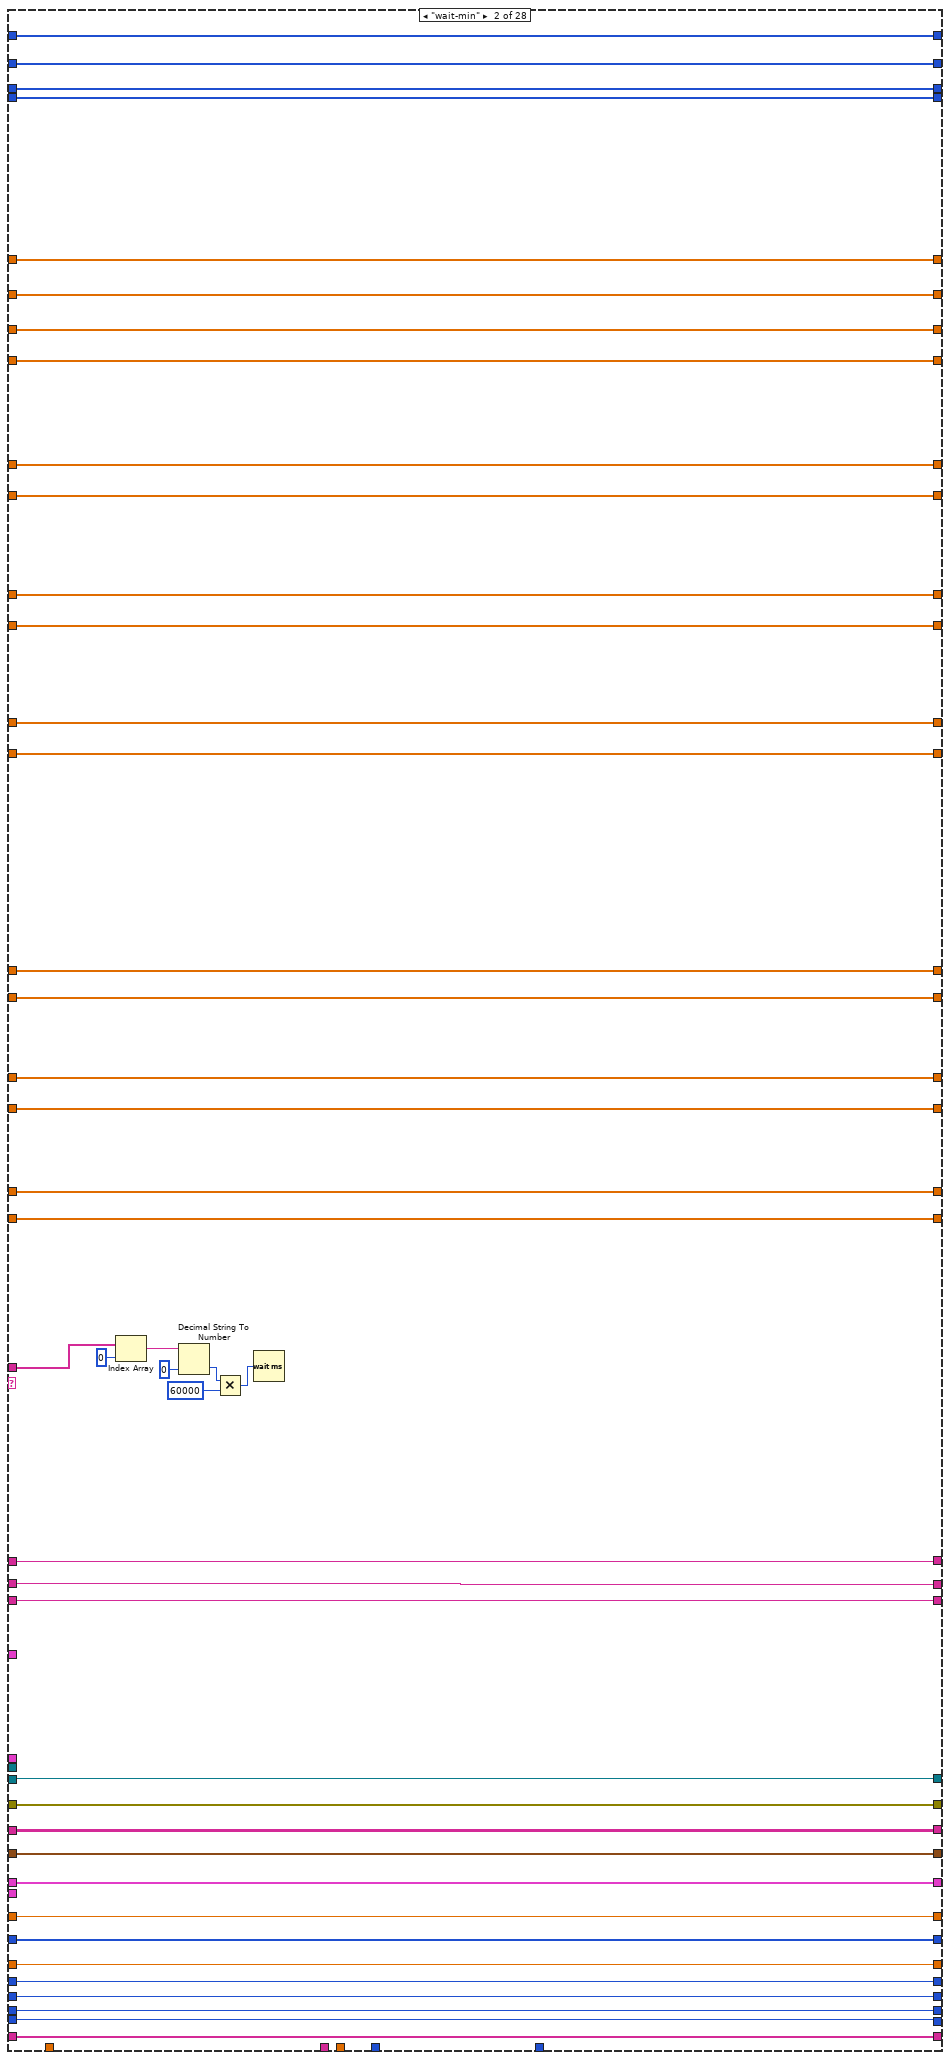
[diagram p7: hidden frame]
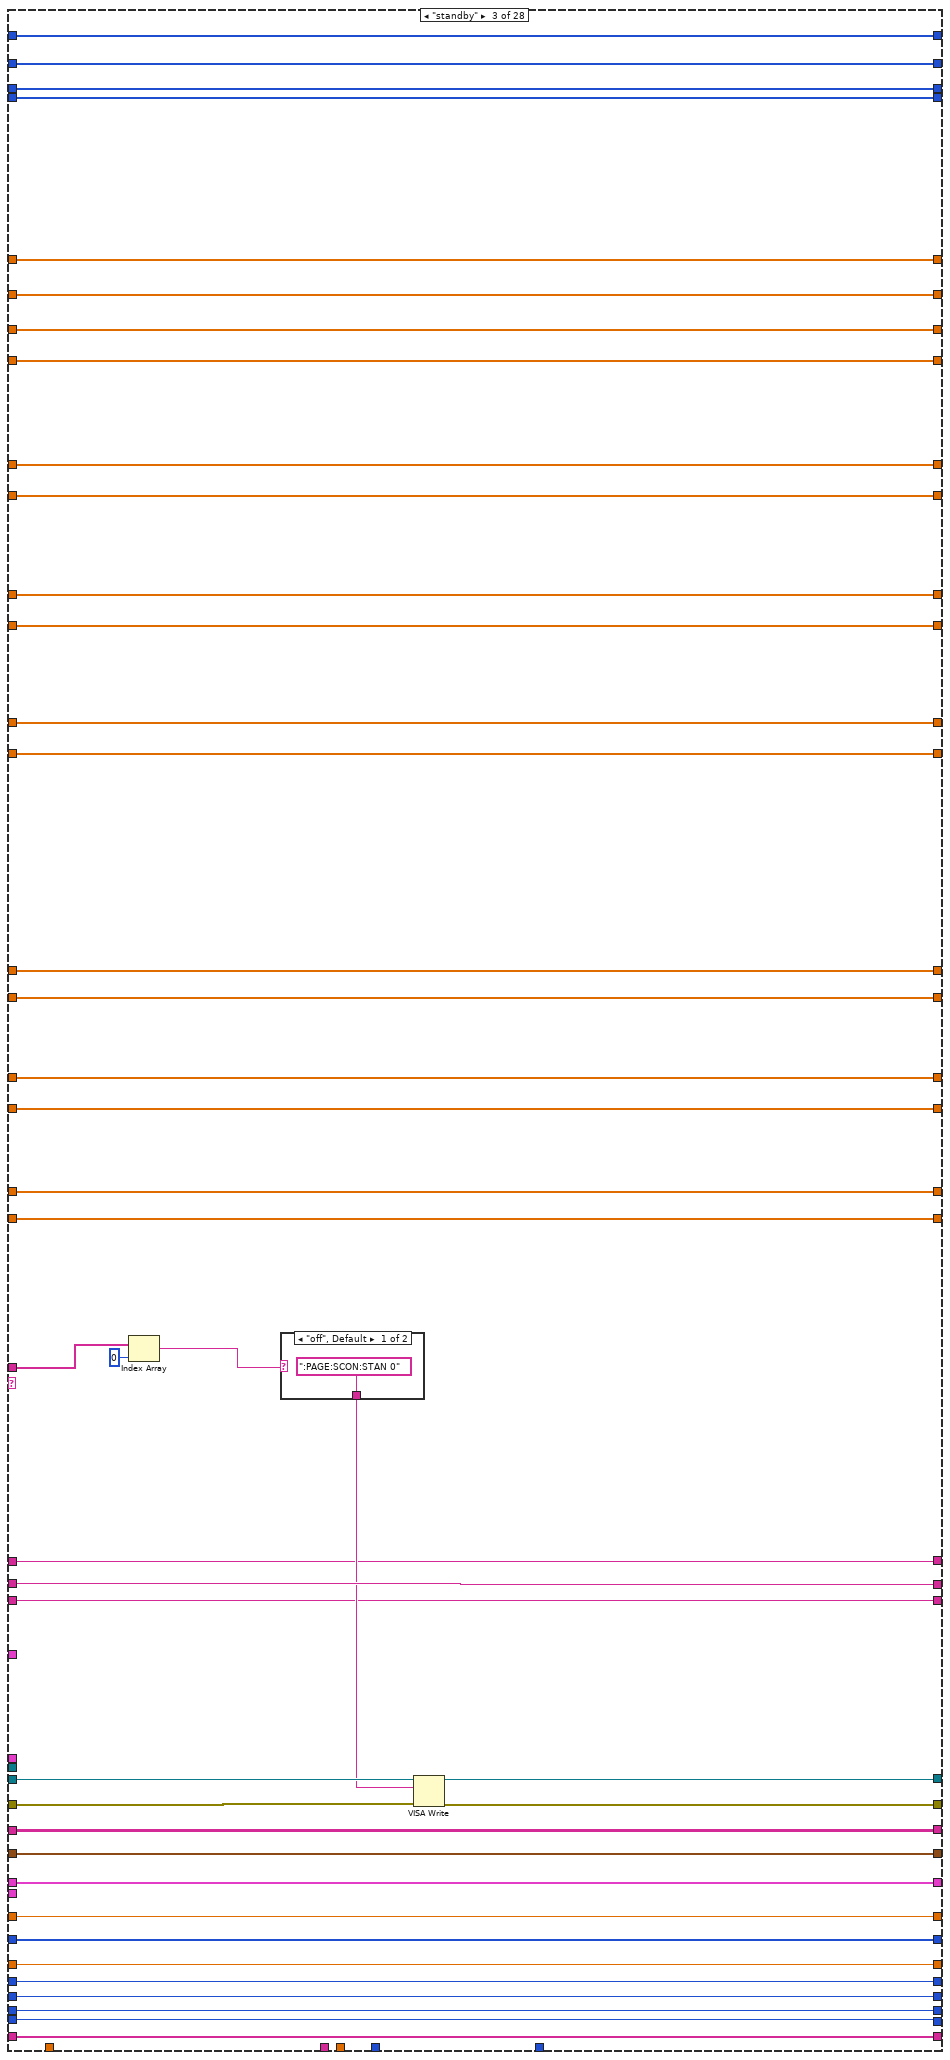
[diagram p8: hidden frame]
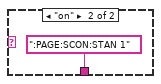
[diagram p9: hidden frame]
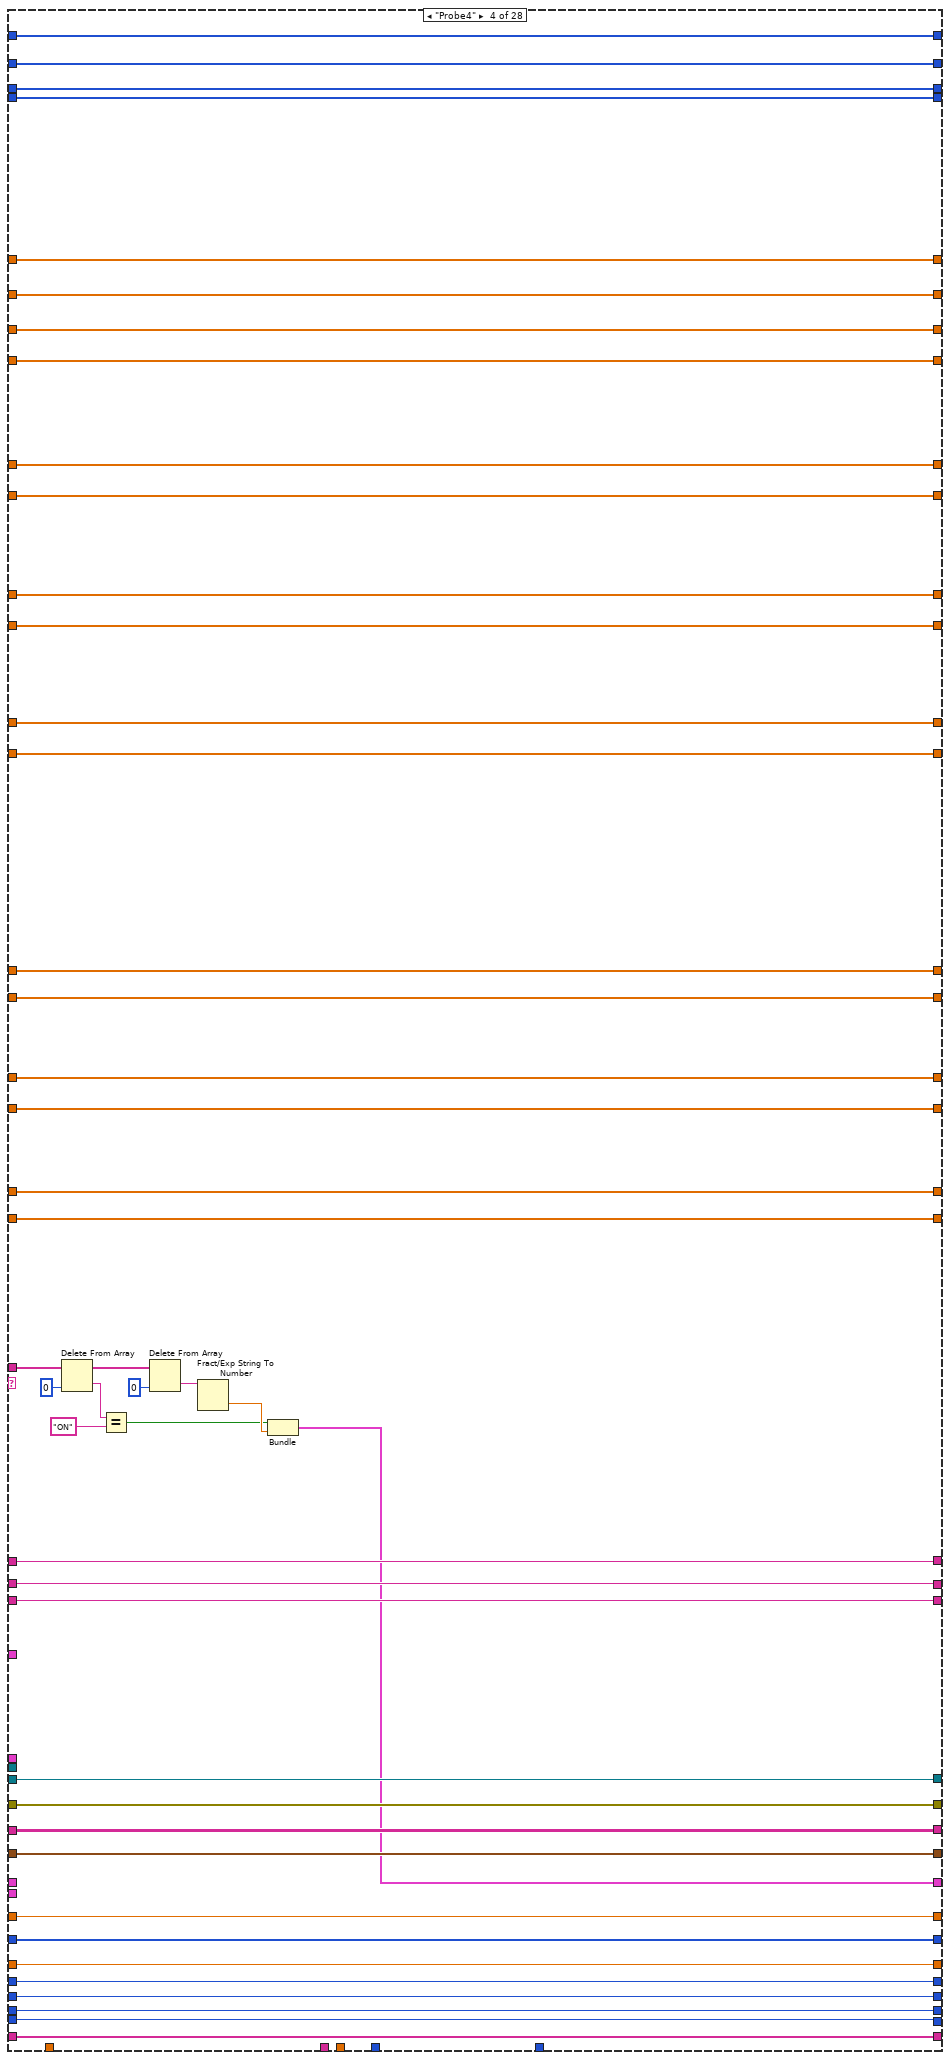
[diagram p10: hidden frame]
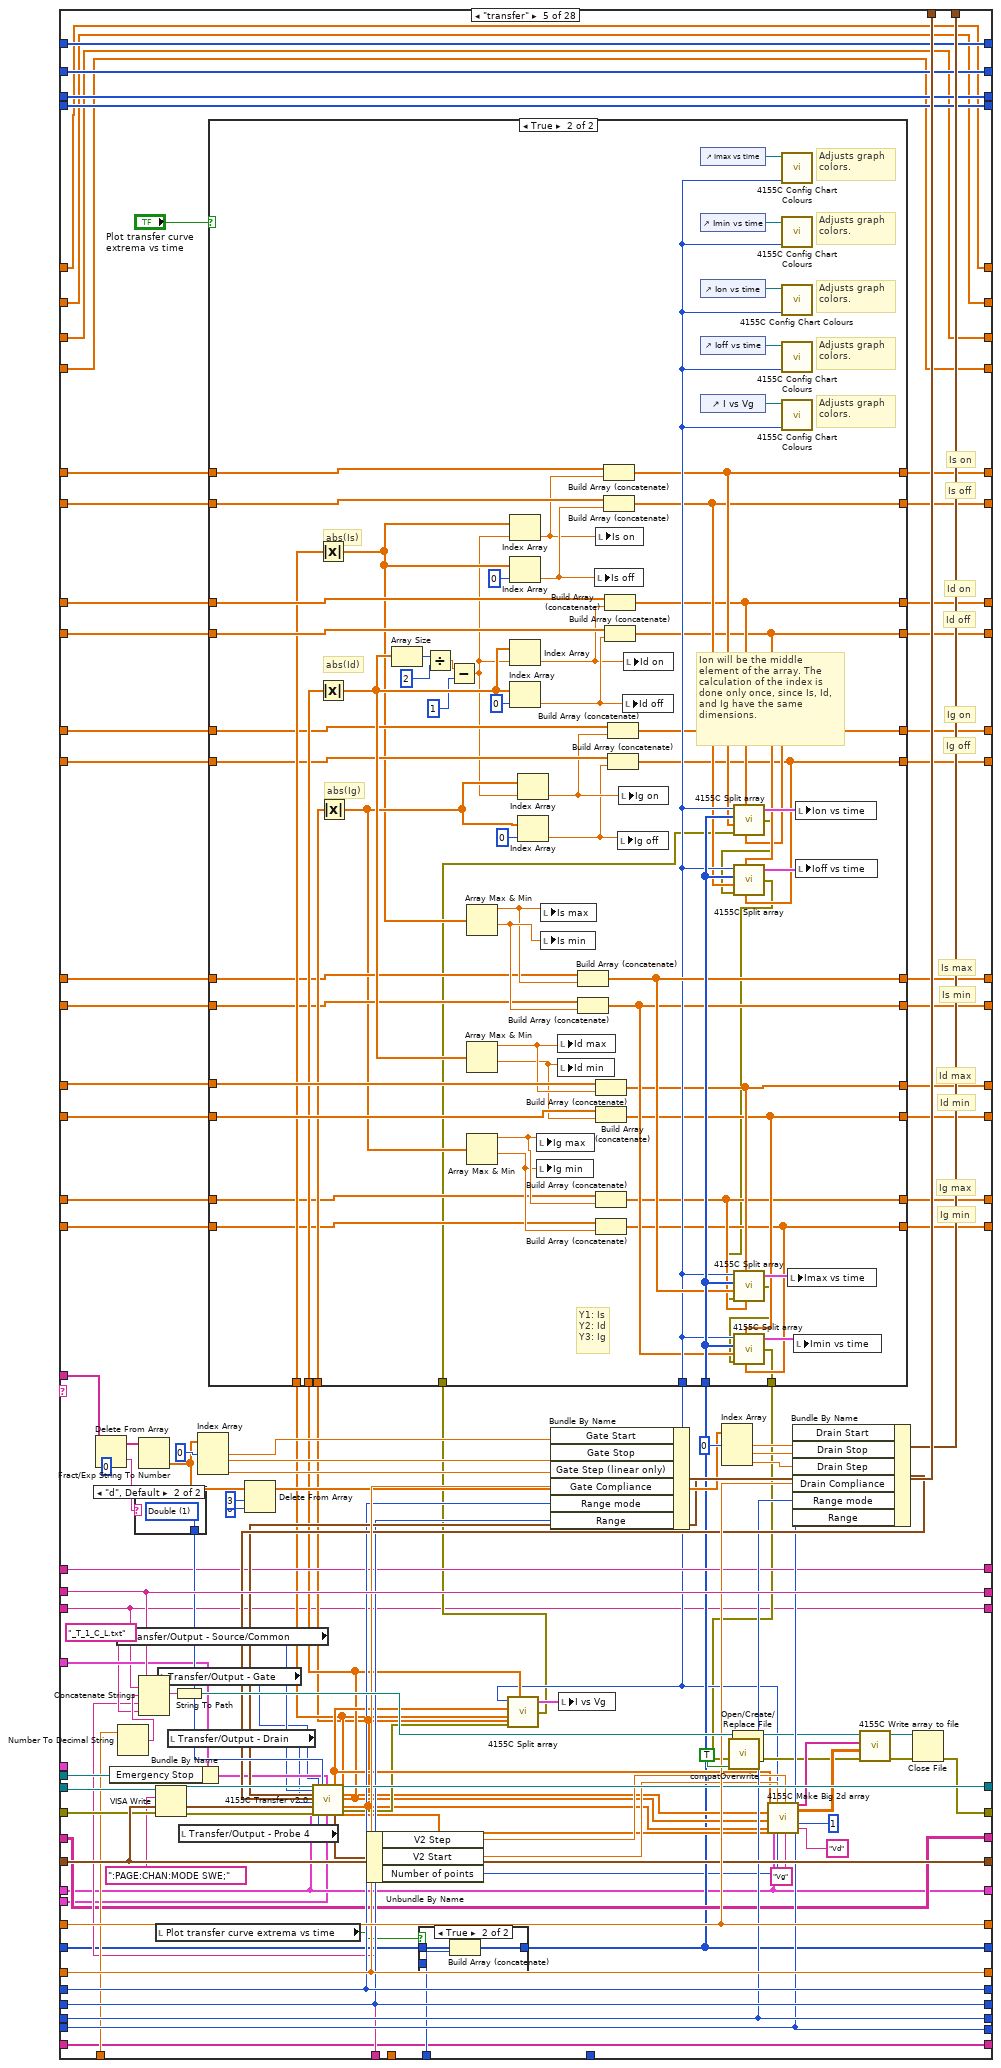
[diagram p11: hidden frame]
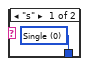
[diagram p14: hidden frame]
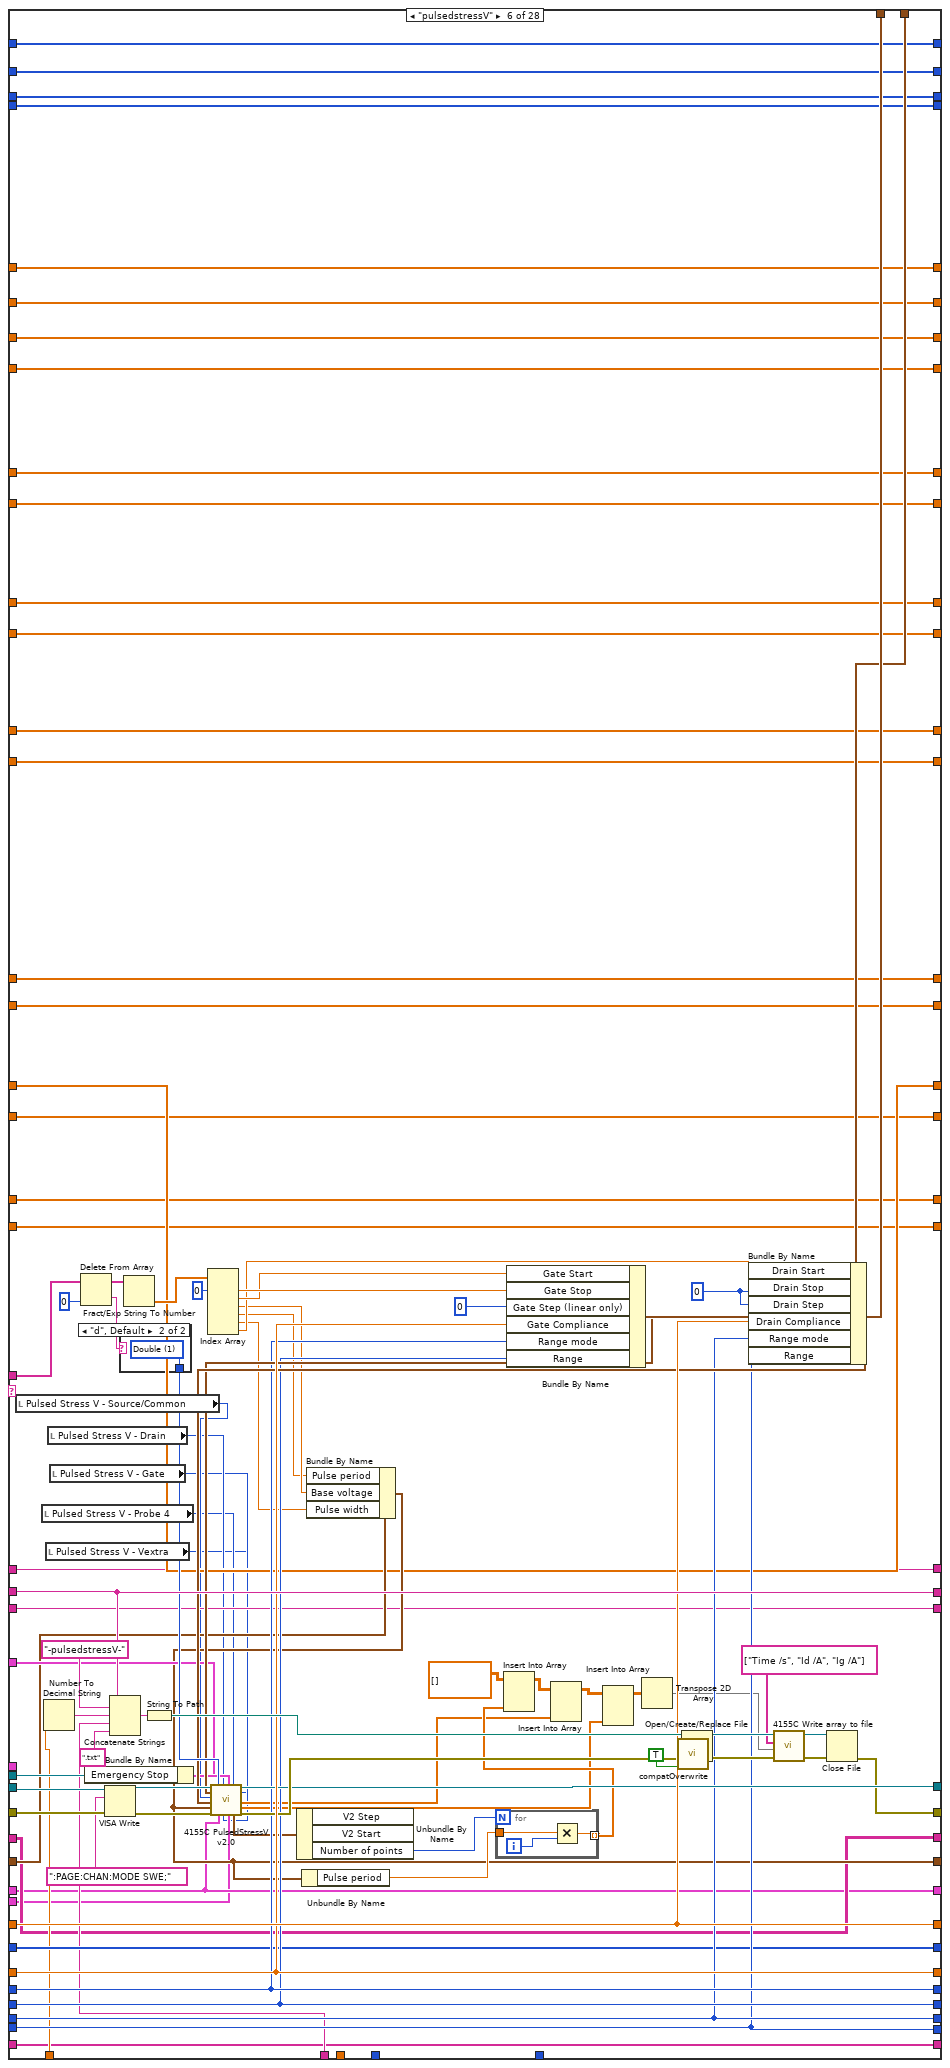
[diagram p15: hidden frame]
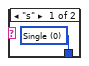
[diagram p16: hidden frame]
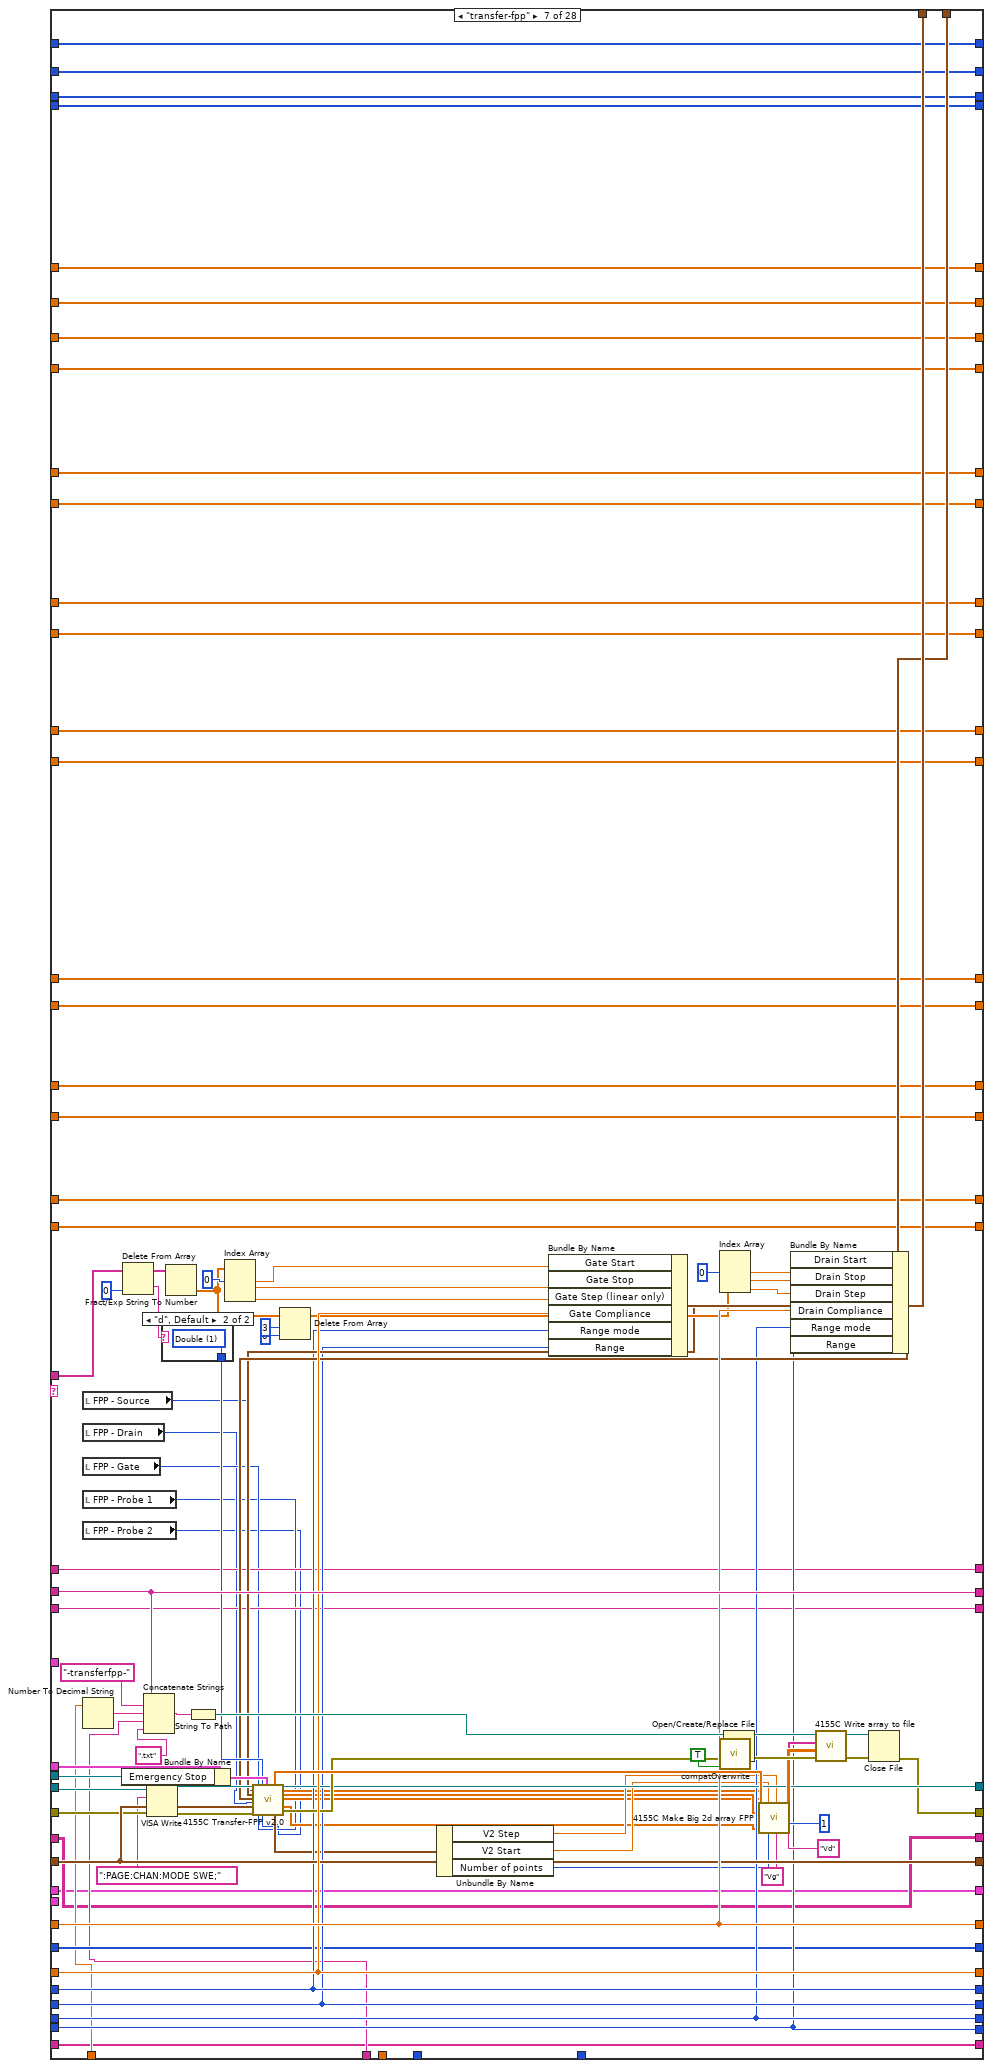
[diagram p17: hidden frame]
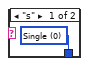
[diagram p18: hidden frame]
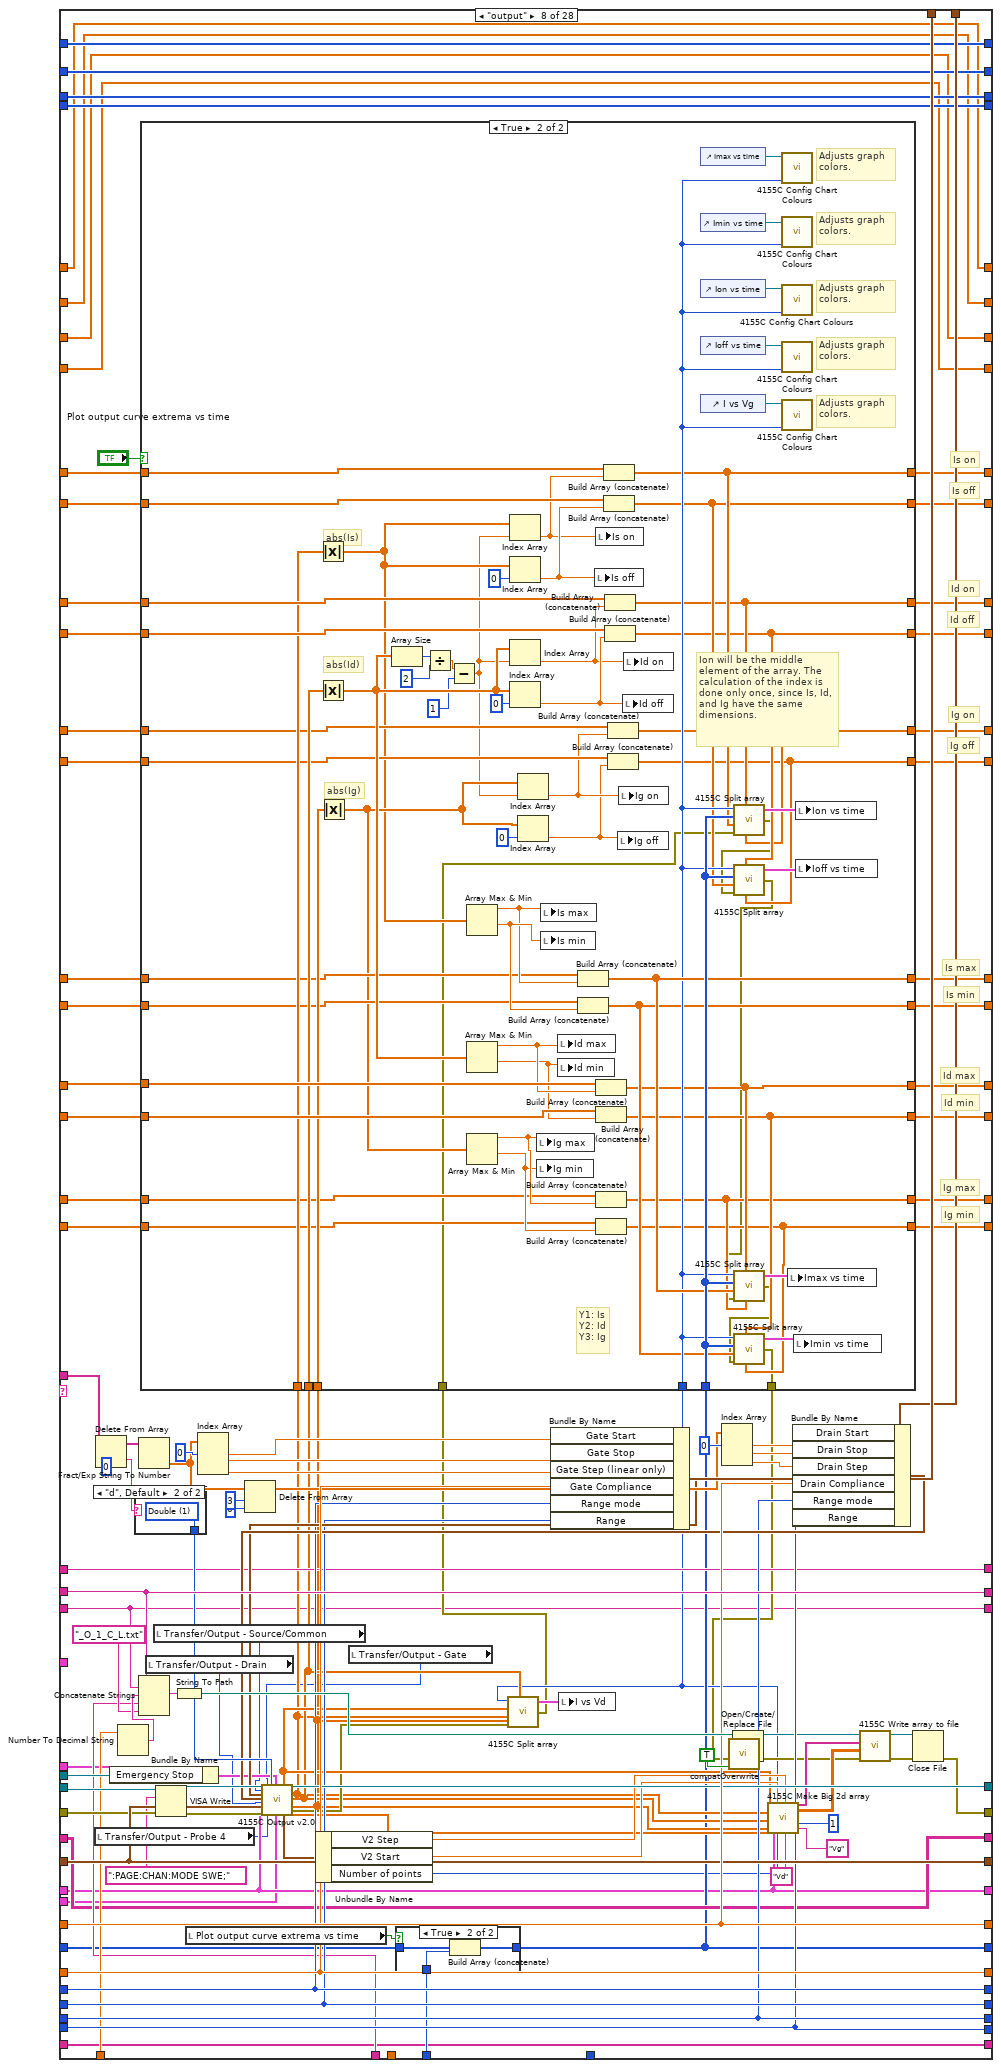
[diagram p19: hidden frame]
diagram:
  w1 = cluster{"Y data in":dbl[], "X data in":dbl[]}[] [] ("I vs Vg")
  w12 = 0.0 ("Is off")
  w13 = 0.0 ("Is on")
  w14 = 0.0 ("Is min")
  w15 = 0.0 ("Is max")
  w63 = u16 1 items=["Reset All", "Partial reset"] ("Type of reset")
  # "Change from previous version:\n\n- Corrected time axis of sample extrema."
  # "This is a version specific to the SPM pump."
  # "I add 1 to both the \"total lines\" and the \"line running\" indicators because i and N begin from 0, and the script lines begin from 1."
  # "Bugs:\n\n- If using the \"filename\" command, keep in mind that the arrays of the time-dependent data are not re-initialized inbetween filename changes. \n\n- Do not connect the \"error\" wire of a Split block if it has unconnected terminals! It will halt the program."
  # "Array size"
  # "%s option converts a spreadsheet string to an array of strings."
  # "0: No of rows of array\n1: No of cols"
  # "Dimitrios Simatos\nv. 7.0"
  # "Changes from original textcontrol.vi:\n\n- Timestamp appears in filename.\n- (Only) transfer and output curves are plotted.\n- Communication with serial port.\n- Can execute any command, as all pattern matching functions were replaced. Previously, commands with special LabVIEW characters could not be executed.\n- Replaced write to file function with write to text file.\n- Replaced while loop with for loop.\n- Replaced 4155C \"Save File\" function and now the vi can save time-dependent variables.\n- Added clock with start time control and various units.\n- Changed filepath in which the program is saved.\n- Added a serial output log that keeps a history.\n- Tab control.\n- Addition of specialized serial read/write file for the SPM OEM pump.\n- Added halt and hard stop.\n- Added option for plotting transfer and output curve extrema vs time.\n- Corrected bug of \"itime\" command. The command did not allow for settting the integration time value, it allowed to set the category of the integration time (short, medium, long). If the time value was beyond the range of the category, then the SPA used the closest value allowed, whilst staying in the category. So, if the integration time was changed to long, but the integration time value was a short one, then the SPA would measure using the minimum long integration time value and not the value that the user intended.\n- Added Probe4 command.\n- Added plotting of \"sample\" plots.\n- Added SMU control."
  # "Search and replace LF with EOL"
  n1 = Equal?(x="integration time", y=u32 0) -> (x = y?=w64:bool)
  n2 = Select(t="Integration time (short)", s=w64, f="Integration time (long)") -> (s? t:f=w16:dbl)
  n3 = call "4155C Get Filename.vi"("error in (no error)"=errorcluster {"status"=FALSE, "code"=0, "source"=""}) -> ("error out"=w58:errorcluster, "path"=w33:path)  [unwired: 2 in, 1 out]
  "Path" <- w33
  n4 = Bundle By Name(cluster="Timings (overwritten by the Front Panel)", "integration time"="integration time", "Short/Long integration time"=w16) -> (w56:T5)
  n5 = Path To String(path=w33) -> (string=w34:string)
  n6 = Search and Replace String(replace all?=TRUE ("replace all? (F)"), input string="Script", search string="\n", replace string="\r\n") -> (result string=w46:string)  [unwired: 4 in, 3 out]
  n7 = Match Pattern(string=w34, regular expression=".txt") -> (before substring=w29:string)  [unwired: 1 in, 3 out]
  n8 = call "4155C Initialise.vi"("VISA resource name in"="VISA resource name in", "Reset"="Full Reset", "Type of reset"=w63, "error in (no error)"=w58, "VISA Timeout Value"=u32 10000) -> ("VISA Resource Name out"=w57:refnum<visa-resource-name>, "error out"=w5:errorcluster)
  n9 = Concatenate Strings(w29, "Suffix (script)") -> (w28:string)
  n10 = Spreadsheet String To Array(delimiter (Tab)="\r\n", format string="%s", spreadsheet string="Script", array type (2D Dbl)="") -> (array=w37:string[][])
  n11 = String To Path(string=w28) -> (path=w8:path)
  n12 = Array Size(array=w37) -> (size(s)=w41:i32[])
  n13 = Initialize Array("") -> (w21:string[])  [unwired: 1 in]
  n14 = Open/Create/Replace File(file path (use dialog)=w8, error in=w5, operation (0:open)=T8."replace or create with confirmation") -> (refnum out=w7:refnum<file>, error out=w6:errorcluster)  [unwired: 3 in, 1 out]
  n15 = Initialize Array(0 ("element")) -> (w23:i32[])  [unwired: 1 in]
  n16 = Initialize Array("") -> (w19:string[][])  [unwired: 2 in]
  n17 = Initialize Array(0.0 ("element")) -> (w2:dbl[])  [unwired: 1 in]
  n18 = Index Array(array=w41, index=0) -> (element=w39:i32)
  n19 = Write to Text File(file (use dialog)=w7, text=w46, error in=w6) -> (error out=w27:errorcluster)  [unwired: 1 in, 2 out]
  n20 = for {
    N: w39 -> [w207]
    shift-left: "Source/Drain Range" -> [w247]
    shift-right: [w243] -> _
    shift-left: "Source/Drain\nRange mode" -> [w248]
    shift-right: [w244] -> _
    shift-left: "Gate Range" -> [w249]
    shift-right: [w245] -> _
    shift-left: "Gate Range\nmode" -> [w250]
    shift-right: [w246] -> _
    shift-left: "Gate: Compliance" -> [w259]
    shift-right: [w255] -> _
    shift-left: "Drain: Compliance" -> [w260]
    shift-right: [w256] -> _
    shift-left: w56 -> [w261]
    shift-right: [w257] -> w17
    shift-left: w27 -> [w262]
    shift-right: [w77] -> w32
    shift-left: w57 -> [w263]
    shift-right: [w258] -> _
    shift-left: w29 -> [w264]
    shift-right: [w76] -> _
    tunnel: "Panel Controls 2" -> [w241]
    shift-right: [w119] -> _
    shift-left: w2 -> [w240]
    shift-right: [w177] -> _
    shift-left: i32[] [] -> [w236]
    tunnel: w37 -> [w235] mode=indexing
    shift-right: [w118] -> _
    shift-left: w2 -> [w212]
    shift-right: [w150] -> _
    shift-left: w21 -> [w199]
    shift-right: [w178] -> _
    shift-left: w23 -> [w194]
    shift-right: [w160] -> _
    shift-left: w23 -> [w193]
    shift-right: [w192] -> _
    shift-left: "" -> [w191]
    shift-right: [w155] -> _
    shift-left: w23 -> [w175]
    shift-right: [w154] -> _
    shift-left: w23 -> [w159]
    shift-right: [w151] -> _
    shift-left: w19 -> [w153]
    shift-right: [w112] -> _
    shift-left: w2 -> [w140]
    shift-right: [w113] -> _
    shift-left: w2 -> [w139]
    shift-right: [w117] -> _
    shift-left: w2 -> [w128]
    shift-right: [w116] -> _
    shift-left: w2 -> [w127]
    shift-right: [w110] -> _
    shift-left: w2 -> [w126]
    shift-right: [w120] -> _
    shift-left: w2 -> [w125]
    shift-right: [w111] -> _
    shift-left: w2 -> [w124]
    shift-right: [w109] -> _
    shift-left: w2 -> [w123]
    shift-right: [w115] -> _
    shift-left: w2 -> [w122]
    shift-right: [w114] -> _
    shift-left: w2 -> [w121]
    shift-right: [w75] -> _
    shift-left: "Filename (variable part)" -> [w104]
    shift-right: [w101] -> w3
    shift-left: "Probe 4" -> [w242]
    shift-right: [w71] -> _
    shift-left: w2 -> [w98]
    shift-right: [w72] -> _
    shift-left: w2 -> [w97]
    shift-right: [w73] -> _
    shift-left: w2 -> [w96]
    shift-right: [w74] -> _
    shift-left: w2 -> [w95]
    i -> [w202]
    stop <- "Interrupt program" stop-if-true
    # "Ig for bias stress plots"
    # "Id for bias stress plots"
    # "Is for bias stress plots"
    # "Time axis for bias stress plots"
    # "Save bias stress curves in file."
    # "Filename prefix"
    # "Is off"
    # "Is on"
    # "Ig off"
    # "Ig on"
    # "Is min"
    # "Is max"
    # "Ig min"
    # "Ig max"
    # "Id min"
    # "Id max"
    # "Id off"
    # "Id on"
    # "Pump status"
    # "Filepath and name"
    # "Pump status"
    # "Limit of command arguments (array columns). Raise if needed."
    # "Serial port data (string)"
    # "Serial port data (table)"
    # "Time array for valve position"
    # "Time array for absolute plunger position"
    # "Valve position"
    # "Absolute plunger position"
    # "Serial port data"
    # "For loop counter"
    # "<-----Equivalent to the 4155C \"Write\" subvi.----->"
    # "Headers"
    # "Save transfer curves in file."
    # "Filepath and name"
    # "Save time-dependent data."
    # "Use the time offset if your measurements do not start at t=0."
    # "Time for Imax, Imin, Ion, Ioff"
    # "Rest of elements of command"
    # "First element of command\n(case select)"
    n21 = Add(x=w202, y=1) -> (x+y=→"Line running":i32)
    n22 = Add(x=w207, y=1) -> (x+y=→"Total lines":i32)
    n23 = Index Array(array=w235, index=0 ("line index")) -> (element=w230:string)
    "Command running:" <- w230
    n24 = control-ref of="Interrupt scan"() -> (w254:refnum<vi>)
    n25 = Spreadsheet String To Array(delimiter (Tab)=" ", format string="%s", spreadsheet string=w230, array type (2D Dbl)=string[] []) -> (array=w228:string[])
    n26 = Delete From Array(array=w228, index=0) -> (deleted portion=w141:string, array with subset deleted=w227:string[])  [unwired: 1 in]
    n27 = call "Elapsed Time"("Reset"="Reset", "Auto Reset"="Auto Reset") -> ("Elapsed Time (s)"=w237:dbl)  [unwired: 10 in, 7 out]
    n28 = case shown="1" "Time Units" {
      tunnel: ["-sec" "-min" "-h"] -> w238
      tunnel: [w268 w272 w275] -> w208
      tunnel: w237 -> [w268 w271 w276]
      frame 0, Default {
      }
      frame 1 {
        n29 = Divide(x=w271, y=60.0) -> (x/y=w272:dbl)
      }
      frame 2 {
        n30 = Divide(x=w276, y=3600.0) -> (x/y=w275:dbl)
      }
    }
    n31 = Add(x=w208, y="Time Offset") -> (x+y=w99:dbl)
    n32 = To Long Integer(number=w99) -> (32bit integer=w100:i32)
    "Elapsed Time" <- w100
    n33 = case shown="\"sample\"" w141 {
      tunnel: w227 -> [w318 w361 w403 w411 w556 w674 w829 w958 w1129 w1161 w1246 w1297 w1346 w1391 w1429 _ _ w1640 w1777 _ w1893 w1963 w2030 w2129 w2215 w2259 w2334 w2393]
      tunnel: w264 -> [w313 w357 w401 w433 w563 w738 w837 w965 w1137 w1184 w1235 w1289 w1339 w1385 w1422 w1465 w1531 w1567 w1759 w1814 w1880 w1950 w2018 w2123 w2211 w2261 w2336 w2395]
      tunnel: w263 -> [w312 w356 w392 w431 w534 w723 w806 w936 w1105 w1185 w1236 w1290 w1340 w1386 w1423 w1470 w1533 w1645 w1783 w1818 w1899 w1969 w2036 w2135 w2169 w2265 w2340 w2397]
      tunnel: w262 -> [w311 w355 w391 w430 w533 w722 w805 w935 w1102 w1186 w1237 w1291 w1341 w1387 w1424 w1469 w1504 w1644 w1782 w1817 w1898 w1968 w2035 w2134 w2168 w2264 w2339 w2398]
      tunnel: w261 -> [w310 w354 w400 w428 w559 w699 w833 w961 w1133 w1194 w1245 w1288 w1338 w1384 w1421 w1468 w1528 w1615 w1751 w1823 w1873 w1943 w2011 w2122 w2210 w2266 w2341 w2400]
      tunnel: w260 -> [w309 w353 w399 w427 w561 w736 w835 w963 w1135 w1193 w1244 w1296 w1345 w1390 w1428 w1467 w1513 w1643 w1781 w1826 w1897 w1967 w2034 w2133 w2219 w2267 w2342 w2401]
      tunnel: w259 -> [w308 w352 w398 w425 w560 w735 w834 w962 w1134 w1192 w1243 w1295 w1344 w1389 w1427 w1466 w1514 w1623 w1760 w1825 w1881 w1951 w2019 w2124 w2212 w2269 w2343 w2403]
      tunnel: [w312 w356 w390 w431 w558 w733 w831 w960 w1131 w1185 w1236 w1290 w1340 w1386 w1423 w1470 w1533 w1616 w1733 w1816 w1874 w1944 w2012 w2076 w2171 w2265 w2340 w2397] -> w258
      tunnel: [w311 w355 w389 w430 w557 w732 w830 w959 w1130 w1186 w1237 w1291 w1341 w1387 w1424 w1469 w1503 w1624 w1734 w1815 w1882 w1952 w2020 w2075 w2170 w2263 w2338 w2398] -> w174
      tunnel: [w310 w354 w400 w428 w559 w695 w833 w961 w1133 w1187 w1238 w1288 w1338 w1384 w1421 w1468 w1528 w1615 w1751 w1823 w1873 w1943 w2011 w2122 w2210 w2266 w2341 w2400] -> w257
      tunnel: [w309 w353 w399 w427 w561 w736 w835 w963 w1135 w1193 w1244 w1296 w1345 w1390 w1428 w1467 w1513 w1643 w1781 w1826 w1897 w1967 w2034 w2133 w2219 w2267 w2342 w2401] -> w256
      tunnel: [w308 w352 w398 w425 w560 w735 w834 w962 w1134 w1192 w1243 w1295 w1344 w1389 w1427 w1466 w1514 w1623 w1760 w1825 w1881 w1951 w2019 w2124 w2212 w2269 w2343 w2403] -> w255
      tunnel: [w313 w357 w401 w433 w563 w738 w837 w965 w1137 w1184 w1235 w1289 w1339 w1385 w1422 w1465 w1531 w1567 w1759 w1814 w1880 w1950 w2018 w2123 w2211 w2261 w2336 w2395] -> w76
      tunnel: w254 -> [_ _ _ _ w565 w742 w842 w967 w1141 _ _ _ _ _ _ _ _ w1620 w1756 _ w1879 w1949 w2017 w2095 w2187 _ _ _]
      tunnel: "Gate" -> [_ _ _ _ w543 w726 w816 w945 w1116 _ _ _ _ _ _ _ _ _ _ _ _ _ _ _ _ _ _ _]
      tunnel: "Drain 2" -> [_ _ _ _ w542 w725 w815 w944 w1115 _ _ _ _ _ _ _ _ _ _ _ _ _ _ _ _ _ _ _]
      tunnel: "Panel Controls" -> [_ _ _ _ _ _ w814 w865 w1114 _ _ _ _ _ _ _ _ _ _ _ _ _ _ _ _ _ _ _]
      tunnel: w250 -> [w307 w351 w397 w424 w527 w716 w799 w929 w1100 w1191 w1242 _ w1337 w1383 w1420 w1464 w1515 w1611 w1747 w1819 w1869 w1939 w2007 w2118 w2206 w2270 w2344 w2404]
      tunnel: w249 -> [w306 w350 w396 w423 w526 w715 w798 w928 w1099 w1190 w1241 w1294 _ w1374 w1426 w1463 w1516 w1612 w1748 w1820 w1870 w1940 w2008 w2119 w2207 w2271 w2345 w2405]
      tunnel: w248 -> [w305 w349 w395 w422 w525 w714 w797 w927 w1098 w1189 w1240 w1293 w1343 w1388 _ w1462 w1517 w1613 w1749 w1821 w1871 w1941 w2009 w2120 w2208 w2272 w2346 w2406]
      tunnel: w247 -> [w304 w348 w394 w421 w524 w713 w796 w926 w1101 w1188 w1239 w1292 w1342 _ w1425 w1461 w1518 w1614 w1750 w1822 w1872 w1942 w2010 w2121 w2209 w2273 w2347 w2407]
      tunnel: [w307 w351 w397 w424 w527 w716 w799 w929 w1100 w1191 w1242 w1287 w1337 w1383 w1420 w1464 w1515 w1611 w1747 w1819 w1869 w1939 w2007 w2118 w2206 w2270 w2344 w2404] -> w246
      tunnel: [w306 w350 w396 w423 w526 w715 w798 w928 w1099 w1190 w1241 w1294 w1329 w1374 w1426 w1463 w1516 w1612 w1748 w1820 w1870 w1940 w2008 w2119 w2207 w2271 w2345 w2405] -> w245
      tunnel: [w305 w349 w395 w422 w525 w714 w797 w927 w1098 w1189 w1240 w1293 w1343 w1388 w1419 w1462 w1517 w1613 w1749 w1821 w1871 w1941 w2009 w2120 w2208 w2272 w2346 w2406] -> w244
      tunnel: [w304 w348 w394 w421 w524 w713 w796 w926 w1101 w1188 w1239 w1292 w1342 w1375 w1425 w1461 w1518 w1614 w1750 w1822 w1872 w1942 w2010 w2121 w2209 w2273 w2347 w2407] -> w243
      tunnel: w242 -> [w282 w323 w366 _ w460 w662 w762 w862 w1063 w1158 w1212 w1265 w1307 w1352 w1397 w1439 w1475 w1588 w1707 w1792 w1834 w1908 w1977 w2049 w2140 w2224 w2278 w2391]
      tunnel: w241 -> [_ _ _ _ w518 w710 _ _ _ _ _ _ _ _ _ _ _ _ _ _ _ _ _ _ _ _ _ _]
      tunnel: [w303 w344 w387 w438 w475 w687 w786 w878 w1087 w1183 w1233 w1286 w1328 w1373 w1418 w1460 w1499 w1577 w1712 w1813 w1858 w1932 w2001 w2073 w2164 w2262 w2337 w2412] -> w119
      tunnel: w240 -> [w303 w344 w387 w438 w515 w687 w786 w918 w1087 w1183 w1233 w1286 w1328 w1373 w1418 w1460 w1499 w1584 w1712 w1813 w1858 w1932 w2001 w2073 w2164 w2262 w2337 w2412]
      tunnel: w99 -> [_ _ _ _ w514 w684 w784 w917 w1084 _ _ _ _ _ _ _ w1497 w1604 w1729 _ w1855 w1929 w1998 w2070 w2160 _ _ _]
      tunnel: w238 -> [_ _ _ _ w511 w683 w782 w914 w1083 _ _ _ _ _ _ _ w1495 w1602 w1728 _ w1854 w1928 w1997 w2069 w2161 _ w2305 _]
      tunnel: w100 -> [_ _ _ _ w507 _ _ w910 _ _ _ _ _ _ _ _ _ _ _ _ _ _ _ _ _ _ w2308 _]
      tunnel: [w302 w343 w386 w426 w479 w686 w785 w882 w1086 w1182 w1232 w1285 w1327 w1372 w1417 w1459 w1498 w1569 w1731 w1812 w1857 w1931 w2000 w2072 w2163 w2268 w2317 w2402] -> w177
      tunnel: w236 -> [w302 w343 w386 w426 w510 w686 w785 w913 w1086 w1182 w1232 w1285 w1327 w1372 w1417 w1459 w1498 w1573 w1731 w1812 w1857 w1931 w2000 w2072 w2163 w2268 w2317 w2402]
      tunnel: [w301 w342 w385 w437 w474 w682 w781 w877 w1082 w1181 w1231 w1284 w1326 w1371 w1416 w1458 w1494 w1576 w1711 w1811 w1853 w1927 w1996 w2068 w2159 w2257 w2333 w2411] -> w118
      tunnel: w212 -> [w301 w342 w385 w437 w506 w682 w781 w909 w1082 w1181 w1231 w1284 w1326 w1371 w1416 w1458 w1494 w1583 w1711 w1811 w1853 w1927 w1996 w2068 w2159 w2257 w2333 w2411]
      tunnel: [w300 w341 w384 w420 w499 w681 w780 w902 w1081 w1180 w1230 w1283 w1325 w1370 w1415 w1457 w1493 w1601 w1727 w1810 w1852 w1926 w1995 w2067 w2158 w2256 w2332 w2408] -> w150
      tunnel: w199 -> [w300 w341 w384 w420 w499 w681 w780 w902 w1081 w1180 w1230 w1283 w1325 w1370 w1415 w1457 w1493 w1601 w1727 w1810 w1852 w1926 w1995 w2067 w2158 w2255 w2306 w2408]
      tunnel: [w299 w340 w383 w448 w498 w680 w779 w901 w1080 w1179 w1229 w1282 w1324 w1369 w1414 w1456 w1492 w1600 w1726 w1809 w1851 w1925 w1994 w2066 w2157 w2241 w2319 w2422] -> w178
      tunnel: w194 -> [w299 w340 w383 w448 w498 w680 w779 w901 w1080 w1179 w1229 w1282 w1324 w1369 w1414 w1456 w1492 w1600 w1726 w1809 w1851 w1925 w1994 w2066 w2157 w2241 w2318 w2422]
      tunnel: [w298 w339 w382 w450 w497 w679 w778 w900 w1079 w1178 w1228 w1281 w1323 w1368 w1413 w1455 w1491 w1599 w1725 w1808 w1850 w1924 w1993 w2065 w2156 w2240 w2301 w2424] -> w160
      tunnel: w193 -> [w298 w339 w382 w450 w497 w679 w778 w900 w1079 w1178 w1228 w1281 w1323 w1368 w1413 w1455 w1491 w1599 w1725 w1808 w1850 w1924 w1993 w2065 w2156 w2240 w2299 w2424]
      tunnel: [w297 w338 w381 w434 w496 w678 w777 w899 w1078 w1177 w1227 w1280 w1322 w1367 w1412 w1454 w1490 w1598 w1724 w1807 w1849 w1923 w1992 w2064 w2155 w2239 w2298 w2396] -> w192
      tunnel: w191 -> [w297 w338 w381 w434 w496 w678 w777 w899 w1078 w1177 w1227 w1280 w1322 w1367 w1412 w1454 w1490 w1598 w1724 w1807 w1849 w1923 w1992 w2064 w2155 w2239 w2309 w2396]
      tunnel: w100 -> [_ _ _ _ _ _ _ _ _ _ _ _ _ _ _ _ _ _ _ _ _ _ _ _ _ _ w2297 _]
      tunnel: w175 -> [w296 w337 w380 w449 w495 w677 w776 w898 w1077 w1176 w1226 w1279 w1321 w1366 w1411 w1453 w1489 w1597 w1723 w1806 w1848 w1922 w1991 w2063 w2154 w2238 w2296 w2423]
      tunnel: [w296 w337 w380 w449 w495 w677 w776 w898 w1077 w1176 w1226 w1279 w1321 w1366 w1411 w1453 w1489 w1597 w1723 w1806 w1848 w1922 w1991 w2063 w2154 w2238 w2295 w2423] -> w155
      tunnel: [w295 w336 w379 w447 w494 w676 w775 w897 w1076 w1175 w1225 w1278 w1320 w1365 w1410 w1452 w1488 w1596 w1722 w1805 w1847 w1921 w1990 w2062 w2153 w2237 w2294 w2421] -> w154
      tunnel: w159 -> [w295 w336 w379 w447 w494 w676 w775 w897 w1076 w1175 w1225 w1278 w1320 w1365 w1410 w1452 w1488 w1596 w1722 w1805 w1847 w1921 w1990 w2062 w2153 w2237 w2293 w2421]
      tunnel: [w294 w335 w378 w429 w493 w675 w774 w896 w1075 w1174 w1224 w1277 w1319 w1364 w1409 w1451 w1487 w1595 w1721 w1804 w1846 w1920 w1989 w2061 w2152 w2236 w2291 w2399] -> w151
      tunnel: w153 -> [w294 w335 w378 w429 w493 w675 w774 w896 w1075 w1174 w1224 w1277 w1319 w1364 w1409 w1451 w1487 w1595 w1721 w1804 w1846 w1920 w1989 w2061 w2152 w2236 w2290 w2399]
      tunnel: [w292 w333 w376 w443 w468 w672 w772 w871 w1073 w1172 w1223 w1276 w1317 w1362 w1407 w1449 w1485 w1594 w1720 w1803 w1845 w1919 w1987 w2060 w2151 w2235 w2289 w2417] -> w112
      tunnel: w140 -> [w292 w333 w376 w443 w492 w672 w772 w895 w1073 w1172 w1223 w1276 w1317 w1362 w1407 w1449 w1485 w1594 w1720 w1803 w1845 w1919 w1987 w2060 w2151 w2235 w2289 w2417]
      tunnel: [w293 w334 w377 w444 w469 w673 w773 w872 w1074 w1173 w1222 w1275 w1318 w1363 w1408 w1450 w1486 w1593 w1719 w1802 w1844 w1918 w1988 w2059 w2150 w2234 w2288 w2418] -> w113
      tunnel: w139 -> [w293 w334 w377 w444 w491 w673 w773 w894 w1074 w1173 w1222 w1275 w1318 w1363 w1408 w1450 w1486 w1593 w1719 w1802 w1844 w1918 w1988 w2059 w2150 w2234 w2288 w2418]
      tunnel: [w285 w326 w369 w436 w473 w669 w770 w876 w1071 w1165 w1220 w1273 w1315 w1360 w1405 w1447 w1478 w1575 w1710 w1801 w1837 w1911 w1980 w2052 w2145 w2227 w2287 w2410] -> w117
      tunnel: w128 -> [w285 w326 w369 w436 w487 w669 w770 w890 w1071 w1165 w1220 w1273 w1315 w1360 w1405 w1447 w1478 w1582 w1710 w1801 w1837 w1911 w1980 w2052 w2145 w2227 w2287 w2410]
      tunnel: [w284 w325 w368 w435 w472 w670 w771 w875 w1072 w1164 w1221 w1274 w1316 w1361 w1406 w1448 w1477 w1574 w1709 w1800 w1836 w1910 w1979 w2051 w2144 w2226 w2286 w2409] -> w116
      tunnel: w127 -> [w284 w325 w368 w435 w486 w670 w771 w889 w1072 w1164 w1221 w1274 w1316 w1361 w1406 w1448 w1477 w1581 w1709 w1800 w1836 w1910 w1979 w2051 w2144 w2226 w2286 w2409]
      tunnel: [w287 w328 w371 w440 w478 w668 w768 w881 w1069 w1170 w1218 w1271 w1313 w1358 w1403 w1445 w1480 w1579 w1714 w1795 w1839 w1913 w1982 w2054 w2143 w2231 w2284 w2414] -> w110
      tunnel: w126 -> [w287 w328 w371 w440 w485 w668 w768 w888 w1069 w1170 w1218 w1271 w1313 w1358 w1403 w1445 w1480 w1586 w1714 w1795 w1839 w1913 w1982 w2054 w2143 w2231 w2284 w2414]
      tunnel: [w286 w327 w370 w439 w476 w671 w769 w879 w1070 w1171 w1219 w1272 w1314 w1359 w1404 w1446 w1479 w1578 w1713 w1794 w1838 w1912 w1981 w2053 w2142 w2230 w2285 w2413] -> w120
      tunnel: w125 -> [w286 w327 w370 w439 w484 w671 w769 w887 w1070 w1171 w1219 w1272 w1314 w1359 w1404 w1446 w1479 w1585 w1713 w1794 w1838 w1912 w1981 w2053 w2142 w2230 w2285 w2413]
      tunnel: [w289 w330 w373 w442 w467 w667 w766 w870 w1067 w1168 w1216 w1269 w1311 w1356 w1401 w1443 w1482 w1590 w1716 w1797 w1841 w1915 w1984 w2056 w2147 w2233 w2282 w2416] -> w111
      tunnel: w124 -> [w289 w330 w373 w442 w483 w667 w766 w886 w1067 w1168 w1216 w1269 w1311 w1356 w1401 w1443 w1482 w1590 w1716 w1797 w1841 w1915 w1984 w2056 w2147 w2233 w2282 w2416]
      tunnel: [w288 w329 w372 w441 w466 w666 w767 w869 w1068 w1169 w1217 w1270 w1312 w1357 w1402 w1444 w1481 w1589 w1715 w1796 w1840 w1914 w1983 w2055 w2146 w2232 w2283 w2415] -> w109
      tunnel: w123 -> [w288 w329 w372 w441 w482 w666 w767 w885 w1068 w1169 w1217 w1270 w1312 w1357 w1402 w1444 w1481 w1589 w1715 w1796 w1840 w1914 w1983 w2055 w2146 w2232 w2283 w2415]
      tunnel: [w291 w332 w375 w446 w471 w665 w764 w874 w1065 w1166 w1214 w1267 w1309 w1354 w1399 w1441 w1484 w1592 w1718 w1799 w1843 w1917 w1986 w2058 w2149 w2229 w2280 w2420] -> w115
      tunnel: w122 -> [w291 w332 w375 w446 w481 w665 w764 w884 w1065 w1166 w1214 w1267 w1309 w1354 w1399 w1441 w1484 w1592 w1718 w1799 w1843 w1917 w1986 w2058 w2149 w2229 w2280 w2420]
      tunnel: [w290 w331 w374 w445 w470 w664 w765 w873 w1066 w1167 w1215 w1268 w1310 w1355 w1400 w1442 w1483 w1591 w1717 w1798 w1842 w1916 w1985 w2057 w2148 w2228 w2281 w2419] -> w114
      tunnel: w121 -> [w290 w331 w374 w445 w480 w664 w765 w883 w1066 w1167 w1215 w1268 w1310 w1355 w1400 w1442 w1483 w1591 w1717 w1798 w1842 w1916 w1985 w2057 w2148 w2228 w2281 w2419]
      tunnel: w104 -> [w283 w324 w367 w432 w463 w663 w763 w866 w1064 w1163 w1213 w1266 w1308 w1353 w1398 w1440 w1476 w1566 w1708 w1793 w1835 w1909 w1978 w2050 w2141 w2225 w2279 _]
      tunnel: [w283 w324 w367 w432 w463 w663 w763 w866 w1064 w1163 w1213 w1266 w1308 w1353 w1398 w1440 w1476 w1566 w1708 w1793 w1835 w1909 w1978 w2050 w2141 w2225 w2279 w2392] -> w75
      tunnel: [w282 w323 w366 w410 w460 w662 w762 w862 w1063 w1158 w1212 w1265 w1307 w1352 w1397 w1439 w1475 w1588 w1707 w1792 w1834 w1908 w1977 w2049 w2140 w2224 w2278 w2391] -> w101
      tunnel: w99 -> [_ _ _ _ _ _ _ _ _ _ _ _ _ _ _ _ _ w1536 _ _ _ _ _ _ _ _ _ _]
      tunnel: [w281 w322 w365 w409 w459 w661 w761 w861 w1062 w1157 w1211 w1264 w1306 w1351 w1396 w1438 w1474 w1550 w1706 w1791 w1833 w1907 w1976 w2048 w2139 w2223 w2277 w2390] -> w71
      tunnel: [w280 w321 w364 w408 w458 w660 w760 w860 w1061 w1156 w1210 w1263 w1305 w1350 w1395 w1437 w1473 w1549 w1705 w1790 w1832 w1906 w1975 w2047 w2138 w2222 w2276 w2389] -> w72
      tunnel: [w279 w320 w363 w407 w457 w659 w759 w859 w1060 w1155 w1209 w1262 w1304 w1349 w1394 w1436 w1472 w1551 w1704 w1789 w1831 w1905 w1974 w2046 w2137 w2221 w2275 w2388] -> w73
      tunnel: [w278 w319 w362 w406 w456 w658 w758 w858 w1059 w1154 w1208 w1261 w1303 w1348 w1393 w1435 w1471 w1548 w1703 w1788 w1830 w1904 w1973 w2045 w2136 w2220 w2274 w2387] -> w74
      tunnel: w98 -> [w281 w322 w365 w409 w459 w661 w761 w861 w1062 w1157 w1211 w1264 w1306 w1351 w1396 w1438 w1474 w1547 w1706 w1791 w1833 w1907 w1976 w2048 w2139 w2223 w2277 w2390]
      tunnel: w97 -> [w280 w321 w364 w408 w458 w660 w760 w860 w1061 w1156 w1210 w1263 w1305 w1350 w1395 w1437 w1473 w1546 w1705 w1790 w1832 w1906 w1975 w2047 w2138 w2222 w2276 w2389]
      tunnel: w96 -> [w279 w320 w363 w407 w457 w659 w759 w859 w1060 w1155 w1209 w1262 w1304 w1349 w1394 w1436 w1472 w1545 w1704 w1789 w1831 w1905 w1974 w2046 w2137 w2221 w2275 w2388]
      tunnel: w95 -> [w278 w319 w362 w406 w456 w658 w758 w858 w1059 w1154 w1208 w1261 w1303 w1348 w1393 w1435 w1471 w1544 w1703 w1788 w1830 w1904 w1973 w2045 w2136 w2220 w2274 w2387]
      tunnel: "Standby" -> [_ _ _ _ w455 w657 _ w857 _ _ _ _ _ _ _ _ _ w1542 w1702 _ _ _ _ w2044 _ _ _ _]
      frame "wait" {
        n34 = Index Array(array=w318, index=0 ("Index")) -> (element=w316:string)
        n35 = Decimal String To Number(string=w316, default (0L)=u32 0) -> (number=w315:u32)  [unwired: 1 in, 1 out]
        n36 = Wait (ms)(milliseconds to wait=w315) -> ()  [unwired: 1 out]
      }
      frame "wait-min" {
        n37 = Index Array(array=w361, index=0 ("Index")) -> (element=w359:string)
        n38 = Decimal String To Number(string=w359, default (0L)=u32 0) -> (number=w347:u32)  [unwired: 1 in, 1 out]
        n39 = Multiply(x=w347, y=u32 60000) -> (x*y=w346:u32)
        n40 = Wait (ms)(milliseconds to wait=w346) -> ()  [unwired: 1 out]
      }
      frame "standby" {
        n41 = Index Array(array=w403, index=0 ("Index")) -> (element=w393:string)
        n42 = case shown="\"off\", Default" w393 {
          tunnel: [":PAGE:SCON:STAN 0" ":PAGE:SCON:STAN 1"] -> w388
          frame "off", Default {
          }
          frame "on" {
          }
        }
        n43 = VISA Write(VISA resource name=w392, write buffer=w388, error in (no error)=w391) -> (VISA resource name out=w390:refnum<visa-resource-name>, error out=w389:errorcluster)  [unwired: 1 out]
      }
      frame "Probe4" {
        n44 = Delete From Array(array=w411, index=0) -> (deleted portion=w414:string, array with subset deleted=w417:string[])  [unwired: 1 in]
        n45 = Equal?(x=w414, y="ON") -> (x = y?=w412:bool)
        n46 = Delete From Array(array=w417, index=0) -> (deleted portion=w416:string)  [unwired: 1 in, 1 out]
        n47 = Fract/Exp String To Number(string=w416) -> (number=w413:dbl)  [unwired: 3 in, 1 out]
        n48 = Bundle(w412, w413) -> (w410:cluster{bool, dbl})  [unwired: 1 in]
      }
      frame "transfer" {
        # "Is off"
        # "Is on"
        # "Ig off"
        # "Ig on"
        # "Is min"
        # "Is max"
        # "Ig min"
        # "Ig max"
        # "Id min"
        # "Id max"
        # "Id off"
        # "Id on"
        n49 = Delete From Array(array=w556, index=0 ("Index")) -> (deleted portion=w554:string, array with subset deleted=w553:string[])  [unwired: 1 in]
        n50 = Bundle By Name(cluster=w518, "Emergency Stop"=w565) -> (w519:T2)
        n51 = local read "Transfer/Output - Source/Common"() -> (w454:u32)
        n52 = Number To Decimal String(number=w514) -> (decimal integer string=w513:string)  [unwired: 1 in]
        n53 = case shown="\"d\", Default" w554 {
          tunnel: [w650 w651] -> w552
          frame "s" {
            w650 = u16 0 items=["Single", "Double"] ("sweep mode")
          }
          frame "d", Default {
            w651 = u16 1 items=["Single", "Double"] ("sweep mode")
          }
        }
        n54 = Fract/Exp String To Number(string=w553) -> (number=w538:dbl[])  [unwired: 3 in, 1 out]
        n55 = Concatenate Strings(w563, w463, w513, w511, "_T_1_C_L.txt" ("Suffix (transfer)")) -> (w564:string)
        n56 = VISA Write(VISA resource name=w534, write buffer=":PAGE:CHAN:MODE SWE;" ("write buffer (\"\")"), error in (no error)=w533) -> (VISA resource name out=w531:refnum<visa-resource-name>, error out=w532:errorcluster)  [unwired: 1 out]
        n57 = local read "Plot transfer curve extrema vs time"() -> (w461:bool)
        n58 = local read "Transfer/Output - Gate"() -> (w452:u32)
        n59 = local read "Transfer/Output - Drain"() -> (w453:u32)
        n60 = String To Path(string=w564) -> (path=w562:path)
        n61 = local read "Transfer/Output - Probe 4"() -> (w451:u32)
        n62 = Index Array(array=w538, index #1=0 ("Index")) -> (element #1=w551:dbl, element #2=w550:dbl, element #3=w549:dbl)  [unwired: 2 in]
        n63 = Delete From Array(array=w538, length=3 ("Length"), index=0 ("Index")) -> (array with subset deleted=w536:dbl[])  [unwired: 1 out]
        n64 = case shown="True" w461 {
          tunnel: w510 -> [w567 w570]
          tunnel: w507 -> [_ w569]
          tunnel: [w567 w568] -> w479
          frame False {
          }
          frame True {
            n65 = Build Array (concatenate)(w570, w569) -> (w568:i32[])
          }
        }
        n66 = Bundle By Name(cluster=w543, "Gate Start"=w551, "Gate Stop"=w550, "Gate Step (linear only)"=w549, "Gate Compliance"=w560, "Range mode"=w527, "Range"=w526) -> (w528:T6)
        n67 = Index Array(array=w536, index #1=0 ("Index")) -> (element #1=w546:dbl, element #2=w545:dbl, element #3=w544:dbl)  [unwired: 2 in]
        n68 = call <vilib>:"compatOverwrite.vi"("overwrite (F)"=TRUE) -> ("overwrite?"=w517:T8)
        n69 = Bundle By Name(cluster=w542, "Drain Start"=w546, "Drain Stop"=w545, "Drain Step"=w544, "Drain Compliance"=w561, "Range mode"=w525, "Range"=w524) -> (w529:T7)
        n70 = call "4155C Transfer v2.0.vi"("VISA resource name in"=w531, "Source/Common"=w454, 2:"Gate"=w528, 3:"Drain"=w529, 4:"Drain"=w453, "Timings"=w559, "error in (no error)"=w532, 7:"Probe 4"=w460, 8:"Gate"=w452, 9:"Probe 4"=w451, "sweep mode"=w552, "Panel Controls"=w519, "Standby"=w455) -> ("VG"=w516:dbl[], "Outparams"=w523:T9, "VISA Resource Name out"=w558:refnum<visa-resource-name>, "IS"=w489:dbl[], "ID"=w490:dbl[], "IG"=w488:dbl[], "error out"=w508:errorcluster, "Probe 4"=w520:dbl[])  [unwired: 7 in]
        n71 = Unbundle By Name(w523) -> ("V2 Step"=w522:dbl, "V2 Start"=w521:dbl, "Number of points"=w477:i32)
        n72 = call "4155C Split array.vi"("Number of VAR2 steps"=w477, "Y2 data in"=w490, "X data in"=w516, "Y1 data in"=w489, "Y3 data in"=w488, "error in (no error)"=w508) -> ("Array of clusters"=w509:cluster{"Y data in":dbl[], "X data in":dbl[]}[], "error out"=w465:errorcluster)  [unwired: 1 in]
        n73 = case shown="True" "Plot transfer curve extrema vs time" {
          tunnel: w515 -> [w579 w649]
          tunnel: w506 -> [w580 w644]
          tunnel: w492 -> [w573 w640]
          tunnel: w491 -> [w574 w639]
          tunnel: w490 -> [_ w636]
          tunnel: w489 -> [_ w634]
          tunnel: w488 -> [_ w633]
          tunnel: w487 -> [w581 w629]
          tunnel: w486 -> [w582 w628]
          tunnel: w485 -> [w577 w625]
          tunnel: w484 -> [w578 w624]
          tunnel: w483 -> [w572 w621]
          tunnel: w482 -> [w571 w620]
          tunnel: w481 -> [w576 w617]
          tunnel: w480 -> [w575 w616]
          tunnel: w479 -> [_ w609]
          tunnel: [w577 w604] -> w478
          tunnel: w477 -> [_ w603]
          tunnel: [w578 w602] -> w476
          tunnel: [w579 w601] -> w475
          tunnel: [w580 w600] -> w474
          tunnel: [w581 w599] -> w473
          tunnel: [w582 w598] -> w472
          tunnel: [w576 w597] -> w471
          tunnel: [w575 w596] -> w470
          tunnel: [w574 w595] -> w469
          tunnel: [w573 w594] -> w468
          tunnel: [w572 w593] -> w467
          tunnel: [w571 w592] -> w466
          tunnel: w465 -> [w583 w591]
          tunnel: [w583 w587] -> w464
          frame False {
          }
          frame True {
            # "Adjusts graph colors."
            # "Adjusts graph colors."
            # "Ion will be the middle element of the array. The calculation of the index is done only once, since Is, Id, and Ig have the same dimensions."
            # "abs(Ig)"
            # "abs(Is)"
            # "Y1: Is\nY2: Id\nY3: Ig"
            # "abs(Id)"
            # "Adjusts graph colors."
            # "Adjusts graph colors."
            # "Adjusts graph colors."
            n74 = Absolute Value(x=w634) -> (abs(x)=w619:dbl[])
            n75 = Absolute Value(x=w636) -> (abs(x)=w635:dbl[])
            n76 = Absolute Value(x=w633) -> (abs(x)=w622:dbl[])
            n77 = Array Size(array=w635) -> (size(s)=w643:i32)
            n78 = Divide(x=w643, y=2) -> (x/y=w586:dbl)
            n79 = Subtract(x=w586, y=1) -> (x-y=w585:dbl)
            n80 = Array Max & Min(array=w619) -> (max value=w626:dbl, min value=w627:dbl)  [unwired: 2 out]
            n81 = Array Max & Min(array=w635) -> (max value=w648:dbl, min value=w632:dbl)  [unwired: 2 out]
            n82 = Array Max & Min(array=w622) -> (max value=w631:dbl, min value=w630:dbl)  [unwired: 2 out]
            n83 = Index Array(array=w619, index=w585) -> (element=w610:dbl)
            n84 = Index Array(array=w619, index=0) -> (element=w611:dbl)
            n85 = Index Array(array=w635, index=w585) -> (element=w612:dbl)
            n86 = Index Array(array=w635, index=0) -> (element=w613:dbl)
            n87 = Index Array(array=w622, index=w585) -> (element=w615:dbl)
            n88 = Index Array(array=w622, index=0) -> (element=w614:dbl)
            n89 = local write "Ig max"(w631) -> ()
            n90 = local write "Ig min"(w630) -> ()
            n91 = local write "Is max"(w626) -> ()
            n92 = local write "Is min"(w627) -> ()
            n93 = local write "Id max"(w648) -> ()
            n94 = local write "Id min"(w632) -> ()
            n95 = Build Array (concatenate)(w625, w626) -> (w604:dbl[])
            n96 = Build Array (concatenate)(w624, w627) -> (w602:dbl[])
            n97 = local write "Is off"(w611) -> ()
            n98 = local write "Is on"(w610) -> ()
            n99 = Build Array (concatenate)(w649, w648) -> (w601:dbl[])
            n100 = Build Array (concatenate)(w644, w632) -> (w600:dbl[])
            n101 = Build Array (concatenate)(w629, w631) -> (w599:dbl[])
            n102 = Build Array (concatenate)(w628, w630) -> (w598:dbl[])
            n103 = Build Array (concatenate)(w617, w610) -> (w597:dbl[])
            n104 = Build Array (concatenate)(w616, w611) -> (w596:dbl[])
            n105 = Build Array (concatenate)(w639, w612) -> (w595:dbl[])
            n106 = Build Array (concatenate)(w640, w613) -> (w594:dbl[])
            n107 = Build Array (concatenate)(w621, w615) -> (w593:dbl[])
            n108 = Build Array (concatenate)(w620, w614) -> (w592:dbl[])
            n109 = local write "Ig off"(w614) -> ()
            n110 = local write "Ig on"(w615) -> ()
            n111 = local write "Id off"(w613) -> ()
            n112 = local write "Id on"(w612) -> ()
            n113 = control-ref of="Imax vs time"() -> (w638:refnum<vi>)
            n114 = control-ref of="Imin vs time"() -> (w637:refnum<vi>)
            n115 = control-ref of="Ion vs time"() -> (w606:refnum<vi>)
            n116 = control-ref of="Ioff vs time"() -> (w605:refnum<vi>)
            n117 = control-ref of="I vs Vg"() -> (w647:refnum<vi>)
            n118 = call "4155C Split array.vi"("Number of VAR2 steps"=w603, "Y2 data in"=w595, "X data in"=w609, "Y1 data in"=w597, "Y3 data in"=w593, "error in (no error)"=w591) -> ("Array of clusters"=w607:cluster{"Y data in":dbl[], "X data in":dbl[]}[], "error out"=w590:errorcluster)  [unwired: 1 in]
            n119 = call "4155C Split array.vi"("Number of VAR2 steps"=w603, "Y2 data in"=w594, "X data in"=w609, "Y1 data in"=w596, "Y3 data in"=w592, "error in (no error)"=w590) -> ("Array of clusters"=w608:cluster{"Y data in":dbl[], "X data in":dbl[]}[], "error out"=w589:errorcluster)  [unwired: 1 in]
            n120 = call "4155C Split array.vi"("Number of VAR2 steps"=w603, "Y2 data in"=w601, "X data in"=w609, "Y1 data in"=w604, "Y3 data in"=w599, "error in (no error)"=w589) -> ("Array of clusters"=w646:cluster{"Y data in":dbl[], "X data in":dbl[]}[], "error out"=w588:errorcluster)  [unwired: 1 in]
            n121 = call "4155C Split array.vi"("Number of VAR2 steps"=w603, "Y2 data in"=w600, "X data in"=w609, "Y1 data in"=w602, "Y3 data in"=w598, "error in (no error)"=w588) -> ("Array of clusters"=w645:cluster{"Y data in":dbl[], "X data in":dbl[]}[], "error out"=w587:errorcluster)  [unwired: 1 in]
            n122 = call "4155C Config Chart Colours.vi"("Numeric"=w603, "XY Graph 2"=w638) -> ()  [unwired: 6 in]
            n123 = call "4155C Config Chart Colours.vi"("Numeric"=w603, "XY Graph 2"=w637) -> ()  [unwired: 6 in]
            n124 = call "4155C Config Chart Colours.vi"("Numeric"=w603, "XY Graph 2"=w606) -> ()  [unwired: 6 in]
            n125 = call "4155C Config Chart Colours.vi"("Numeric"=w603, "XY Graph 2"=w605) -> ()  [unwired: 6 in]
            n126 = call "4155C Config Chart Colours.vi"("Numeric"=w603, "XY Graph 2"=w647) -> ()  [unwired: 6 in]
            n127 = local write "Imax vs time"(w646) -> ()
            n128 = local write "Imin vs time"(w645) -> ()
            n129 = local write "Ion vs time"(w607) -> ()
            n130 = local write "Ioff vs time"(w608) -> ()
          }
        }
        n131 = local write "I vs Vg"(w509) -> ()
        n132 = Open/Create/Replace File(file path (use dialog)=w562, error in=w464, operation (0:open)=w517) -> (refnum out=w504:refnum<file>, error out=w502:errorcluster)  [unwired: 3 in, 1 out]
        n133 = call "4155C Make Big 2d array.vi"("1D Var1"=w516, "1d IS"=w489, "1d ID"=w490, "1d IG"=w488, "1d SMU4"=w520, "SMU4"=w460, "VAR2 START"=w521, "Number of VAR2 steps"=w477, "VAR2 STEP"=w522, "VAR1 Name"="Vg", "Decimal places in header"=i8 1, "VAR2 Name"="Vd") -> ("Header array"=w505:string[], "Data array"=w503:dbl[][])  [unwired: 14 in]
        n134 = call "4155C Write array to file.vi"("Byte Stream File Refnum"=w504, "Header"=w505, "Data Array"=w503, "error in (no error)"=w502) -> ("dup refnum"=w501:refnum<file>, "error out"=w500:errorcluster)  [unwired: 1 in]
        n135 = Close File(refnum=w501, error in=w500) -> (error out=w557:errorcluster)  [unwired: 1 out]
      }
      frame "pulsedstressV" {
        w693 = 0
        n136 = local read "Pulsed Stress V - Source/Common"() -> (w656:u32)
        n137 = local read "Pulsed Stress V - Probe 4"() -> (w653:u32)
        n138 = Number To Decimal String(number=w684) -> (decimal integer string=w739:string)  [unwired: 1 in]
        n139 = local read "Pulsed Stress V - Vextra"() -> (w652:u32)
        n140 = local read "Pulsed Stress V - Drain"() -> (w655:u32)
        n141 = local read "Pulsed Stress V - Gate"() -> (w654:u32)
        n142 = Delete From Array(array=w674, index=0 ("Index")) -> (deleted portion=w730:string, array with subset deleted=w729:string[])  [unwired: 1 in]
        n143 = Bundle By Name(cluster=w710, "Emergency Stop"=w742) -> (w711:T2)
        n144 = VISA Write(VISA resource name=w723, write buffer=":PAGE:CHAN:MODE SWE;" ("write buffer (\"\")"), error in (no error)=w722) -> (VISA resource name out=w720:refnum<visa-resource-name>, error out=w721:errorcluster)  [unwired: 1 out]
        n145 = Concatenate Strings(w738, "-pulsedstressV-" ("Substring"), w739, w683, ".txt" ("Substring")) -> (w741:string)
        n146 = case shown="\"d\", Default" w730 {
          tunnel: [w751 w752] -> w728
          frame "s" {
            w751 = u16 0 items=["Single", "Double"] ("sweep mode")
          }
          frame "d", Default {
            w752 = u16 1 items=["Single", "Double"] ("sweep mode")
          }
        }
        n147 = Fract/Exp String To Number(string=w729) -> (number=w724:dbl[])  [unwired: 3 in, 1 out]
        n148 = String To Path(string=w741) -> (path=w737:path)
        n149 = Index Array(array=w724, index #1=0 ("Index")) -> (element #1=w702:dbl, element #2=w701:dbl, element #3=w698:dbl, element #4=w697:dbl, element #5=w696:dbl, element #6=w700:dbl)  [unwired: 5 in]
        n150 = Bundle By Name(cluster=w699, "Pulse period"=w697, "Base voltage"=w698, "Pulse width"=w696) -> (w695:T5)
        n151 = Unbundle By Name(w695) -> ("Pulse period"=w703:dbl)
        n152 = Bundle By Name(cluster=w726, "Gate Start"=w701, "Gate Stop"=w702, "Gate Step (linear only)"=0, "Gate Compliance"=w735, "Range mode"=w716, "Range"=w715) -> (w717:T6)
        n153 = call <vilib>:"compatOverwrite.vi"("overwrite (F)"=TRUE) -> ("overwrite?"=w688:T8)
        n154 = Bundle By Name(cluster=w725, "Drain Start"=w700, "Drain Stop"=w693, "Drain Step"=w693, "Drain Compliance"=w736, "Range mode"=w714, "Range"=w713) -> (w718:T7)
        n155 = call "4155C PulsedStressV v2.0.vi"("VISA resource name in"=w720, "Gate"=w717, "Pulsed Stress V - Source/Common"=w656, "Drain"=w718, "Timings"=w695, "error in (no error)"=w721, "sweep mode"=w728, "Probe 4"=w662, "Pulsed Stress V - Drain"=w655, "Pulsed Stress V - Gate"=w654, "Panel Controls"=w711, "Standby"=w657, "Pulsed Stress V - Probe 4"=w653, "Pulsed Stress V - Vextra"=w652) -> ("Outparams"=w712:T9, "VISA Resource Name out"=w733:refnum<visa-resource-name>, "ID"=w691:dbl[], "IG"=w689:dbl[], "error out"=w734:errorcluster)  [unwired: 1 in]
        n156 = Unbundle By Name(w712) -> ("Number of points"=w690:i32)  [unwired: 2 out]
        n157 = for {
          N: w690 -> [_]
          tunnel: [w748] -> w692 mode=indexing
          tunnel: w703 -> [w750]
          i -> [w749]
          n158 = Multiply(x=w750, y=w749) -> (x*y=w748:dbl)
        }
        n159 = Insert Into Array(array=dbl[][] [] ("Input Array"), new element=w692) -> (w704:dbl[][])  [unwired: 2 in]
        n160 = Insert Into Array(array=w704, new element=w691) -> (w709:dbl[][])  [unwired: 2 in]
        n161 = Insert Into Array(array=w709, new element=w689) -> (w708:dbl[][])  [unwired: 2 in]
        n162 = Transpose 2D Array(2D array=w708) -> (transposed array=w707:dbl[][])
        n163 = Open/Create/Replace File(file path (use dialog)=w737, error in=w734, operation (0:open)=w688) -> (refnum out=w745:refnum<file>, error out=w746:errorcluster)  [unwired: 3 in, 1 out]
        n164 = call "4155C Write array to file.vi"("Byte Stream File Refnum"=w745, "Header"=string[] ["Time /s", "Id /A", "Ig /A"], "Data Array"=w707, "error in (no error)"=w746) -> ("dup refnum"=w743:refnum<file>, "error out"=w744:errorcluster)  [unwired: 1 in]
        n165 = Close File(refnum=w743, error in=w744) -> (error out=w732:errorcluster)  [unwired: 1 out]
      }
      frame "transfer-fpp" {
        n166 = local read "FPP - Source"() -> (w757:u32)
        n167 = local read "FPP - Drain"() -> (w755:u32)
        n168 = local read "FPP - Gate"() -> (w756:u32)
        n169 = local read "FPP - Probe 1"() -> (w754:u32)
        n170 = local read "FPP - Probe 2"() -> (w753:u32)
        n171 = Number To Decimal String(number=w784) -> (decimal integer string=w838:string)  [unwired: 1 in]
        n172 = Bundle By Name(cluster=w814, "Emergency Stop"=w842) -> (w850:T1)
        n173 = Delete From Array(array=w829, index=0 ("Index")) -> (deleted portion=w827:string, array with subset deleted=w826:string[])  [unwired: 1 in]
        n174 = Concatenate Strings(w837, "-transferfpp-" ("Substring"), w838, w782, ".txt" ("Substring")) -> (w840:string)
        n175 = VISA Write(VISA resource name=w806, write buffer=":PAGE:CHAN:MODE SWE;" ("write buffer (\"\")"), error in (no error)=w805) -> (VISA resource name out=w803:refnum<visa-resource-name>, error out=w804:errorcluster)  [unwired: 1 out]
        n176 = case shown="\"d\", Default" w827 {
          tunnel: [w851 w852] -> w825
          frame "s" {
            w851 = u16 0 items=["Single", "Double"] ("sweep mode")
          }
          frame "d", Default {
            w852 = u16 1 items=["Single", "Double"] ("sweep mode")
          }
        }
        n177 = Fract/Exp String To Number(string=w826) -> (number=w810:dbl[])  [unwired: 3 in, 1 out]
        n178 = String To Path(string=w840) -> (path=w836:path)
        n179 = Index Array(array=w810, index #1=0 ("Index")) -> (element #1=w824:dbl, element #2=w823:dbl, element #3=w822:dbl)  [unwired: 2 in]
        n180 = Delete From Array(array=w810, length=3 ("Length"), index=0 ("Index")) -> (array with subset deleted=w808:dbl[])  [unwired: 1 out]
        n181 = Bundle By Name(cluster=w816, "Gate Start"=w824, "Gate Stop"=w823, "Gate Step (linear only)"=w822, "Gate Compliance"=w834, "Range mode"=w799, "Range"=w798) -> (w800:T6)
        n182 = Index Array(array=w808, index #1=0 ("Index")) -> (element #1=w819:dbl, element #2=w818:dbl, element #3=w817:dbl)  [unwired: 2 in]
        n183 = call <vilib>:"compatOverwrite.vi"("overwrite (F)"=TRUE) -> ("overwrite?"=w787:T8)
        n184 = Bundle By Name(cluster=w815, "Drain Start"=w819, "Drain Stop"=w818, "Drain Step"=w817, "Drain Compliance"=w835, "Range mode"=w797, "Range"=w796) -> (w801:T7)
        n185 = call "4155C Transfer-FPP v2.0.vi"("VISA resource name in"=w803, "FPP - Source"=w757, "Gate"=w800, "Drain"=w801, "FPP - Drain"=w755, "Timings"=w833, "error in (no error)"=w804, "FPP - Gate"=w756, "FPP - Probe 1"=w754, "sweep mode"=w825, "FPP - Probe 2"=w753, "Panel Controls"=w850) -> ("VG"=w841:dbl[], "Outparams"=w795:T9, "VISA Resource Name out"=w831:refnum<visa-resource-name>, "Vprobe2"=w791:dbl[], "ID"=w790:dbl[], "IG"=w789:dbl[], "Vprobe1"=w788:dbl[], "error out"=w832:errorcluster)  [unwired: 8 in]
        n186 = Unbundle By Name(w795) -> ("V2 Step"=w794:dbl, "V2 Start"=w793:dbl, "Number of points"=w792:i32)
        n187 = Open/Create/Replace File(file path (use dialog)=w836, error in=w832, operation (0:open)=w787) -> (refnum out=w847:refnum<file>, error out=w848:errorcluster)  [unwired: 3 in, 1 out]
        n188 = call "4155C Make Big 2d array FPP.vi"("1D Var1"=w841, "1d ID"=w790, "1d Vp2"=w791, "1d IG"=w789, "1d Vp1"=w788, "VAR2 START"=w793, "Number of VAR2 steps"=w792, "VAR2 STEP"=w794, "VAR1 Name"="Vg", "Decimal places in header"=i8 1, "VAR2 Name"="Vd") -> ("Header array"=w843:string[], "Data array"=w844:dbl[][])  [unwired: 15 in]
        n189 = call "4155C Write array to file.vi"("Byte Stream File Refnum"=w847, "Header"=w843, "Data Array"=w844, "error in (no error)"=w848) -> ("dup refnum"=w845:refnum<file>, "error out"=w846:errorcluster)  [unwired: 1 in]
        n190 = Close File(refnum=w845, error in=w846) -> (error out=w830:errorcluster)  [unwired: 1 out]
      }
      frame "output" {
        # "Is off"
        # "Is on"
        # "Ig off"
        # "Ig on"
        # "Is min"
        # "Is max"
        # "Ig min"
        # "Ig max"
        # "Id min"
        # "Id max"
        # "Id off"
        # "Id on"
        n191 = local read "Transfer/Output - Probe 4"() -> (w853:u32)
        n192 = Delete From Array(array=w958, index=0 ("Index")) -> (deleted portion=w956:string, array with subset deleted=w955:string[])  [unwired: 1 in]
        n193 = Bundle By Name(cluster=w865, "Emergency Stop"=w967) -> (w921:T1)
        n194 = Number To Decimal String(number=w917) -> (decimal integer string=w916:string)  [unwired: 1 in]
        n195 = case shown="\"d\", Default" w956 {
          tunnel: [w1052 w1053] -> w954
          frame "s" {
            w1052 = u16 0 items=["Single", "Double"] ("sweep mode")
          }
          frame "d", Default {
            w1053 = u16 1 items=["Single", "Double"] ("sweep mode")
          }
        }
        n196 = Fract/Exp String To Number(string=w955) -> (number=w940:dbl[])  [unwired: 3 in, 1 out]
        n197 = Concatenate Strings(w965, w866, w916, w914, "_O_1_C_L.txt" ("Suffix (transfer)")) -> (w966:string)
        n198 = local read "Transfer/Output - Drain"() -> (w855:u32)
        n199 = local read "Transfer/Output - Source/Common"() -> (w856:u32)
        n200 = VISA Write(VISA resource name=w936, write buffer=":PAGE:CHAN:MODE SWE;" ("write buffer (\"\")"), error in (no error)=w935) -> (VISA resource name out=w933:refnum<visa-resource-name>, error out=w934:errorcluster)  [unwired: 1 out]
        n201 = String To Path(string=w966) -> (path=w964:path)
        n202 = local read "Plot output curve extrema vs time"() -> (w863:bool)
        n203 = Index Array(array=w940, index #1=0 ("Index")) -> (element #1=w953:dbl, element #2=w952:dbl, element #3=w951:dbl)  [unwired: 2 in]
        n204 = Delete From Array(array=w940, length=3 ("Length"), index=0 ("Index")) -> (array with subset deleted=w938:dbl[])  [unwired: 1 out]
        n205 = local read "Transfer/Output - Gate"() -> (w854:u32)
        n206 = case shown="True" w863 {
          tunnel: w913 -> [w969 w972]
          tunnel: w910 -> [_ w971]
          tunnel: [w969 w970] -> w882
          frame False {
          }
          frame True {
            n207 = Build Array (concatenate)(w972, w971) -> (w970:i32[])
          }
        }
        n208 = Bundle By Name(cluster=w945, "Gate Start"=w953, "Gate Stop"=w952, "Gate Step (linear only)"=w951, "Gate Compliance"=w962, "Range mode"=w929, "Range"=w928) -> (w930:T6)
        n209 = Index Array(array=w938, index #1=0 ("Index")) -> (element #1=w948:dbl, element #2=w947:dbl, element #3=w946:dbl)  [unwired: 2 in]
        n210 = call <vilib>:"compatOverwrite.vi"("overwrite (F)"=TRUE) -> ("overwrite?"=w920:T8)
        n211 = Bundle By Name(cluster=w944, "Drain Start"=w948, "Drain Stop"=w947, "Drain Step"=w946, "Drain Compliance"=w963, "Range mode"=w927, "Range"=w926) -> (w931:T7)
        n212 = call "4155C Output v2.0.vi"("VISA resource name in"=w933, "Source/Common"=w856, 2:"Gate"=w930, 3:"Drain"=w931, 4:"Drain"=w855, "Timings"=w961, "error in (no error)"=w934, 7:"Probe 4"=w862, 8:"Gate"=w854, 9:"Probe 4"=w853, "sweep mode"=w954, "Panel controls"=w921, "Standby"=w857) -> ("VD"=w919:dbl[], "Outparams"=w925:T9, "VISA Resource Name out"=w960:refnum<visa-resource-name>, "IS"=w892:dbl[], "ID"=w893:dbl[], "IG"=w891:dbl[], "error out"=w911:errorcluster, "Probe 4"=w922:dbl[])  [unwired: 7 in]
        n213 = Unbundle By Name(w925) -> ("V2 Step"=w924:dbl, "V2 Start"=w923:dbl, "Number of points"=w880:i32)
        n214 = call "4155C Split array.vi"("Number of VAR2 steps"=w880, "Y2 data in"=w893, "X data in"=w919, "Y1 data in"=w892, "Y3 data in"=w891, "error in (no error)"=w911) -> ("Array of clusters"=w912:cluster{"Y data in":dbl[], "X data in":dbl[]}[], "error out"=w868:errorcluster)  [unwired: 1 in]
        n215 = case shown="True" "Plot output curve extrema vs time" {
          tunnel: w918 -> [w976 w1051]
          tunnel: w909 -> [w975 w1046]
          tunnel: w895 -> [w981 w1042]
          tunnel: w894 -> [w982 w1041]
          tunnel: w893 -> [_ w1038]
          tunnel: w892 -> [_ w1036]
          tunnel: w891 -> [_ w1035]
          tunnel: w890 -> [w974 w1031]
          tunnel: w889 -> [w973 w1030]
          tunnel: w888 -> [w978 w1027]
          tunnel: w887 -> [w977 w1026]
          tunnel: w886 -> [w980 w1023]
          tunnel: w885 -> [w979 w1022]
          tunnel: w884 -> [w984 w1019]
          tunnel: w883 -> [w983 w1018]
          tunnel: w882 -> [_ w1011]
          tunnel: [w978 w1006] -> w881
          tunnel: w880 -> [_ w1005]
          tunnel: [w977 w1004] -> w879
          tunnel: [w976 w1003] -> w878
          tunnel: [w975 w1002] -> w877
          tunnel: [w974 w1001] -> w876
          tunnel: [w973 w1000] -> w875
          tunnel: [w984 w999] -> w874
          tunnel: [w983 w998] -> w873
          tunnel: [w982 w997] -> w872
          tunnel: [w981 w996] -> w871
          tunnel: [w980 w995] -> w870
          tunnel: [w979 w994] -> w869
          tunnel: w868 -> [w985 w993]
          tunnel: [w985 w989] -> w867
          frame False {
          }
          frame True {
            # "Adjusts graph colors."
            # "Adjusts graph colors."
            # "Ion will be the middle element of the array. The calculation of the index is done only once, since Is, Id, and Ig have the same dimensions."
            # "abs(Ig)"
            # "abs(Is)"
            # "Y1: Is\nY2: Id\nY3: Ig"
            # "abs(Id)"
            # "Adjusts graph colors."
            # "Adjusts graph colors."
            # "Adjusts graph colors."
            n216 = Absolute Value(x=w1036) -> (abs(x)=w1021:dbl[])
            n217 = Absolute Value(x=w1038) -> (abs(x)=w1037:dbl[])
            n218 = Absolute Value(x=w1035) -> (abs(x)=w1024:dbl[])
            n219 = Array Size(array=w1037) -> (size(s)=w1045:i32)
            n220 = Divide(x=w1045, y=2) -> (x/y=w988:dbl)
            n221 = Subtract(x=w988, y=1) -> (x-y=w987:dbl)
            n222 = Array Max & Min(array=w1021) -> (max value=w1028:dbl, min value=w1029:dbl)  [unwired: 2 out]
            n223 = Array Max & Min(array=w1037) -> (max value=w1050:dbl, min value=w1034:dbl)  [unwired: 2 out]
            n224 = Array Max & Min(array=w1024) -> (max value=w1033:dbl, min value=w1032:dbl)  [unwired: 2 out]
            n225 = Index Array(array=w1021, index=w987) -> (element=w1012:dbl)
            n226 = Index Array(array=w1021, index=0) -> (element=w1013:dbl)
            n227 = Index Array(array=w1037, index=w987) -> (element=w1014:dbl)
            n228 = Index Array(array=w1037, index=0) -> (element=w1015:dbl)
            n229 = Index Array(array=w1024, index=w987) -> (element=w1017:dbl)
            n230 = Index Array(array=w1024, index=0) -> (element=w1016:dbl)
            n231 = local write "Ig max"(w1033) -> ()
            n232 = local write "Ig min"(w1032) -> ()
            n233 = local write "Is max"(w1028) -> ()
            n234 = local write "Is min"(w1029) -> ()
            n235 = local write "Id max"(w1050) -> ()
            n236 = local write "Id min"(w1034) -> ()
            n237 = Build Array (concatenate)(w1027, w1028) -> (w1006:dbl[])
            n238 = Build Array (concatenate)(w1026, w1029) -> (w1004:dbl[])
            n239 = local write "Is off"(w1013) -> ()
            n240 = local write "Is on"(w1012) -> ()
            n241 = Build Array (concatenate)(w1051, w1050) -> (w1003:dbl[])
            n242 = Build Array (concatenate)(w1046, w1034) -> (w1002:dbl[])
            n243 = Build Array (concatenate)(w1031, w1033) -> (w1001:dbl[])
            n244 = Build Array (concatenate)(w1030, w1032) -> (w1000:dbl[])
            n245 = Build Array (concatenate)(w1019, w1012) -> (w999:dbl[])
            n246 = Build Array (concatenate)(w1018, w1013) -> (w998:dbl[])
            n247 = Build Array (concatenate)(w1041, w1014) -> (w997:dbl[])
            n248 = Build Array (concatenate)(w1042, w1015) -> (w996:dbl[])
            n249 = Build Array (concatenate)(w1023, w1017) -> (w995:dbl[])
            n250 = Build Array (concatenate)(w1022, w1016) -> (w994:dbl[])
            n251 = local write "Ig off"(w1016) -> ()
            n252 = local write "Ig on"(w1017) -> ()
            n253 = local write "Id off"(w1015) -> ()
            n254 = local write "Id on"(w1014) -> ()
            n255 = control-ref of="Imax vs time"() -> (w1040:refnum<vi>)
            n256 = control-ref of="Imin vs time"() -> (w1039:refnum<vi>)
            n257 = control-ref of="Ion vs time"() -> (w1008:refnum<vi>)
            n258 = control-ref of="Ioff vs time"() -> (w1007:refnum<vi>)
            n259 = control-ref of="I vs Vg"() -> (w1049:refnum<vi>)
            n260 = call "4155C Split array.vi"("Number of VAR2 steps"=w1005, "Y2 data in"=w997, "X data in"=w1011, "Y1 data in"=w999, "Y3 data in"=w995, "error in (no error)"=w993) -> ("Array of clusters"=w1009:cluster{"Y data in":dbl[], "X data in":dbl[]}[], "error out"=w992:errorcluster)  [unwired: 1 in]
            n261 = call "4155C Split array.vi"("Number of VAR2 steps"=w1005, "Y2 data in"=w996, "X data in"=w1011, "Y1 data in"=w998, "Y3 data in"=w994, "error in (no error)"=w992) -> ("Array of clusters"=w1010:cluster{"Y data in":dbl[], "X data in":dbl[]}[], "error out"=w991:errorcluster)  [unwired: 1 in]
            n262 = call "4155C Split array.vi"("Number of VAR2 steps"=w1005, "Y2 data in"=w1003, "X data in"=w1011, "Y1 data in"=w1006, "Y3 data in"=w1001, "error in (no error)"=w991) -> ("Array of clusters"=w1048:cluster{"Y data in":dbl[], "X data in":dbl[]}[], "error out"=w990:errorcluster)  [unwired: 1 in]
            n263 = call "4155C Split array.vi"("Number of VAR2 steps"=w1005, "Y2 data in"=w1002, "X data in"=w1011, "Y1 data in"=w1004, "Y3 data in"=w1000, "error in (no error)"=w990) -> ("Array of clusters"=w1047:cluster{"Y data in":dbl[], "X data in":dbl[]}[], "error out"=w989:errorcluster)  [unwired: 1 in]
            n264 = call "4155C Config Chart Colours.vi"("Numeric"=w1005, "XY Graph 2"=w1040) -> ()  [unwired: 6 in]
            n265 = call "4155C Config Chart Colours.vi"("Numeric"=w1005, "XY Graph 2"=w1039) -> ()  [unwired: 6 in]
            n266 = call "4155C Config Chart Colours.vi"("Numeric"=w1005, "XY Graph 2"=w1008) -> ()  [unwired: 6 in]
            n267 = call "4155C Config Chart Colours.vi"("Numeric"=w1005, "XY Graph 2"=w1007) -> ()  [unwired: 6 in]
            n268 = call "4155C Config Chart Colours.vi"("Numeric"=w1005, "XY Graph 2"=w1049) -> ()  [unwired: 6 in]
            n269 = local write "Imax vs time"(w1048) -> ()
            n270 = local write "Imin vs time"(w1047) -> ()
            n271 = local write "Ion vs time"(w1009) -> ()
            n272 = local write "Ioff vs time"(w1010) -> ()
          }
        }
        n273 = local write "I vs Vd"(w912) -> ()
        n274 = Open/Create/Replace File(file path (use dialog)=w964, error in=w867, operation (0:open)=w920) -> (refnum out=w907:refnum<file>, error out=w905:errorcluster)  [unwired: 3 in, 1 out]
        n275 = call "4155C Make Big 2d array.vi"("1D Var1"=w919, "1d IS"=w892, "1d ID"=w893, "1d IG"=w891, "1d SMU4"=w922, "SMU4"=w862, "VAR2 START"=w923, "Number of VAR2 steps"=w880, "VAR2 STEP"=w924, "VAR1 Name"="Vd", "Decimal places in header"=i8 1, "VAR2 Name"="Vg") -> ("Header array"=w908:string[], "Data array"=w906:dbl[][])  [unwired: 14 in]
        n276 = call "4155C Write array to file.vi"("Byte Stream File Refnum"=w907, "Header"=w908, "Data Array"=w906, "error in (no error)"=w905) -> ("dup refnum"=w904:refnum<file>, "error out"=w903:errorcluster)  [unwired: 1 in]
        n277 = Close File(refnum=w904, error in=w903) -> (error out=w959:errorcluster)  [unwired: 1 out]
      }
      frame "output-fpp" {
        n278 = local read "FPP - Source"() -> (w1058:u32)
        n279 = local read "FPP - Drain"() -> (w1057:u32)
        n280 = local read "FPP - Gate"() -> (w1056:u32)
        n281 = local read "FPP - Probe 1"() -> (w1055:u32)
        n282 = local read "FPP - Probe 2"() -> (w1054:u32)
        n283 = Number To Decimal String(number=w1084) -> (decimal integer string=w1138:string)  [unwired: 1 in]
        n284 = Bundle By Name(cluster=w1114, "Emergency Stop"=w1141) -> (w1151:T1)
        n285 = Delete From Array(array=w1129, index=0 ("Index")) -> (deleted portion=w1127:string, array with subset deleted=w1126:string[])  [unwired: 1 in]
        n286 = VISA Write(VISA resource name=w1105, write buffer=":PAGE:CHAN:MODE SWE;" ("write buffer (\"\")"), error in (no error)=w1102) -> (VISA resource name out=w1104:refnum<visa-resource-name>, error out=w1103:errorcluster)  [unwired: 1 out]
        n287 = Concatenate Strings(w1137, "-outputfpp-" ("Substring"), w1138, w1083, ".txt" ("Substring")) -> (w1140:string)
        n288 = case shown="\"d\", Default" w1127 {
          tunnel: [w1152 w1153] -> w1125
          frame "s" {
            w1152 = u16 0 items=["Single", "Double"] ("sweep mode")
          }
          frame "d", Default {
            w1153 = u16 1 items=["Single", "Double"] ("sweep mode")
          }
        }
        n289 = Fract/Exp String To Number(string=w1126) -> (number=w1108:dbl[])  [unwired: 3 in, 1 out]
        n290 = String To Path(string=w1140) -> (path=w1136:path)
        n291 = Index Array(array=w1108, index #1=0 ("Index")) -> (element #1=w1124:dbl, element #2=w1123:dbl, element #3=w1122:dbl)  [unwired: 2 in]
        n292 = Delete From Array(array=w1108, length=3 ("Length"), index=0 ("Index")) -> (array with subset deleted=w1107:dbl[])  [unwired: 1 out]
        n293 = Bundle By Name(cluster=w1116, "Gate Start"=w1124, "Gate Stop"=w1123, "Gate Step (linear only)"=w1122, "Gate Compliance"=w1134, "Range mode"=w1100, "Range"=w1099) -> (w1150:T6)
        n294 = Index Array(array=w1107, index #1=0 ("Index")) -> (element #1=w1119:dbl, element #2=w1118:dbl, element #3=w1117:dbl)  [unwired: 2 in]
        n295 = call <vilib>:"compatOverwrite.vi"("overwrite (F)"=TRUE) -> ("overwrite?"=w1088:T8)
        n296 = Bundle By Name(cluster=w1115, "Drain Start"=w1119, "Drain Stop"=w1118, "Drain Step"=w1117, "Drain Compliance"=w1135, "Range mode"=w1098, "Range"=w1101) -> (w1149:T7)
        n297 = call "4155C Output-FPP v2.0.vi"("VISA resource name in"=w1104, "FPP - Source"=w1058, "Gate"=w1150, "Drain"=w1149, "FPP - Drain"=w1057, "Timings"=w1133, "error in (no error)"=w1103, "FPP - Gate"=w1056, "FPP - Probe 1"=w1055, "sweep mode"=w1125, "FPP - Probe 2"=w1054, "Panel controls"=w1151) -> ("VD"=w1093:dbl[], "Outparams"=w1096:T9, "VISA Resource Name out"=w1131:refnum<visa-resource-name>, "Vprobe2"=w1092:dbl[], "ID"=w1091:dbl[], "IG"=w1090:dbl[], "Vprobe1"=w1089:dbl[], "error out"=w1132:errorcluster)  [unwired: 8 in]
        n298 = Unbundle By Name(w1096) -> ("V2 Step"=w1097:dbl, "V2 Start"=w1095:dbl, "Number of points"=w1094:i32)
        n299 = Open/Create/Replace File(file path (use dialog)=w1136, error in=w1132, operation (0:open)=w1088) -> (refnum out=w1146:refnum<file>, error out=w1147:errorcluster)  [unwired: 3 in, 1 out]
        n300 = call "4155C Make Big 2d array FPP.vi"("1D Var1"=w1093, "1d ID"=w1091, "1d Vp2"=w1092, "1d IG"=w1090, "1d Vp1"=w1089, "VAR2 START"=w1095, "Number of VAR2 steps"=w1094, "VAR2 STEP"=w1097, "VAR1 Name"="Vd", "Decimal places in header"=i8 1, "VAR2 Name"="Vg") -> ("Header array"=w1142:string[], "Data array"=w1143:dbl[][])  [unwired: 15 in]
        n301 = call "4155C Write array to file.vi"("Byte Stream File Refnum"=w1146, "Header"=w1142, "Data Array"=w1143, "error in (no error)"=w1147) -> ("dup refnum"=w1144:refnum<file>, "error out"=w1145:errorcluster)  [unwired: 1 in]
        n302 = Close File(refnum=w1144, error in=w1145) -> (error out=w1130:errorcluster)  [unwired: 1 out]
      }
      frame "itime" {
        n303 = Delete From Array(array=w1161, index=1) -> (deleted portion=w1160:string)  [unwired: 1 in, 1 out]
        n304 = Delete From Array(array=w1161, index=0 ("Index")) -> (deleted portion=w1195:string)  [unwired: 1 in, 1 out]
        n305 = Fract/Exp String To Number(string=w1160) -> (number=w1159:dbl)  [unwired: 3 in, 1 out]
        n306 = case shown="\"l\"" w1195 {
          tunnel: w1194 -> [w1200 w1202 w1206]
          tunnel: [w1199 w1201 w1205] -> w1187
          tunnel: w1159 -> [w1197 _ w1204]
          frame "s" {
            w1198 = u32 0 items=["short  ", "medium  ", "long  "] ("integration time 2")
            n307 = Bundle By Name(cluster=w1200, "integration time"=w1198, "Short/Long integration time"=w1197) -> (w1199:T5)
          }
          frame "m", Default {
            w1203 = u32 1 items=["short  ", "medium  ", "long  "] ("integration time 2")
            n308 = Bundle By Name(cluster=w1202, "integration time"=w1203) -> (w1201:T5)
          }
          frame "l" {
            w1207 = u32 2 items=["short  ", "medium  ", "long  "] ("integration time 2")
            n309 = Bundle By Name(cluster=w1206, "integration time"=w1207, "Short/Long integration time"=w1204) -> (w1205:T5)
          }
        }
      }
      frame "pulsed" {
        n310 = Delete From Array(array=w1246, index=0 ("Index")) -> (deleted portion=w1247:string, array with subset deleted=w1234:string[])  [unwired: 1 in]
        n311 = case shown="\"on\", Default" w1247 {
          tunnel: w1245 -> [w1257 w1260]
          tunnel: [w1256 w1259] -> w1238
          tunnel: w1234 -> [w1254 _]
          frame "on", Default {
            w1255 = u16 1 items=["Continuous", "Pulsed"] ("sweep method")
            n312 = Fract/Exp String To Number(string=w1254) -> (number=w1252:dbl[])  [unwired: 3 in, 1 out]
            n313 = Index Array(array=w1252, index #1=0 ("Index")) -> (element #1=w1251:dbl, element #2=w1250:dbl, element #3=w1249:dbl)  [unwired: 2 in]
            n314 = Bundle By Name(cluster=w1257, "sweep method"=w1255, "Pulse period"=w1251, "Base voltage"=w1250, "Pulse width"=w1249) -> (w1256:T5)
          }
          frame "off" {
            w1258 = u16 0 items=["Continuous", "Pulsed"] ("sweep method")
            n315 = Bundle By Name(cluster=w1260, "sweep method"=w1258) -> (w1259:T5)
          }
        }
      }
      frame "gaterangemode" {
        n316 = Delete From Array(array=w1297, index=0 ("Index")) -> (deleted portion=w1298:string)  [unwired: 1 in, 1 out]
        n317 = case shown="\"f\"" w1298 {
          tunnel: [w1300 w1301 w1302] -> w1287
          frame "a", Default {
            w1300 = u16 0 items=["Auto", "Limited", "Fixed"] ("Gate Range\nmode 2")
          }
          frame "f" {
            w1301 = u16 2 items=["Auto", "Limited", "Fixed"] ("Gate Range\nmode 2")
          }
          frame "l" {
            w1302 = u16 1 items=["Auto", "Limited", "Fixed"] ("Gate Range\nmode 2")
          }
        }
      }
      frame "gaterange" {
        (unwired) u8 11 items=["10fA  ", "100fA  ", "1nA  ", "10nA", "100nA", "1uA", "10uA", "100uA", "1mA", "10mA", "100mA", "1A"] ("Gate Range 2")
        n318 = Delete From Array(array=w1346, index=0 ("Index")) -> (deleted portion=w1336:string)  [unwired: 1 in, 1 out]
        n319 = Scan Value(string=w1336, format string="") -> (value=w1334:dbl)  [unwired: 1 in, 1 out]
        n320 = Logarithm Base 10(1:w1334) -> (0:w1333:dbl)
        n321 = Round To Nearest(number=w1333) -> (nearest integer value=w1332:dbl)
        n322 = Add(x=w1332, y=11.0) -> (x+y=w1330:dbl)
        n323 = To Unsigned Byte Integer(number=w1330) -> (unsigned 8bit integer=w1329:u8)
      }
      frame "drainrange" {
        (unwired) u8 11 items=["10fA  ", "100fA  ", "1nA  ", "10nA", "100nA", "1uA", "10uA", "100uA", "1mA", "10mA", "100mA", "1A"] ("Gate Range 2")
        n324 = Delete From Array(array=w1391, index=0 ("Index")) -> (deleted portion=w1382:string)  [unwired: 1 in, 1 out]
        n325 = Scan Value(string=w1382, format string="") -> (value=w1380:dbl)  [unwired: 1 in, 1 out]
        n326 = Logarithm Base 10(1:w1380) -> (0:w1379:dbl)
        n327 = Round To Nearest(number=w1379) -> (nearest integer value=w1378:dbl)
        n328 = Add(x=w1378, y=11.0) -> (x+y=w1376:dbl)
        n329 = To Unsigned Byte Integer(number=w1376) -> (unsigned 8bit integer=w1375:u8)
      }
      frame "drainrangemode" {
        n330 = Delete From Array(array=w1429, index=0 ("Index")) -> (deleted portion=w1430:string)  [unwired: 1 in, 1 out]
        n331 = case shown="\"f\"" w1430 {
          tunnel: [w1432 w1433 w1434] -> w1419
          frame "a", Default {
            w1432 = u16 0 items=["Auto", "Limited", "Fixed"] ("Gate Range\nmode 2")
          }
          frame "f" {
            w1433 = u16 2 items=["Auto", "Limited", "Fixed"] ("Gate Range\nmode 2")
          }
          frame "l" {
            w1434 = u16 1 items=["Auto", "Limited", "Fixed"] ("Gate Range\nmode 2")
          }
        }
      }
      frame "Error", Default {
      }
      frame "logfile" {
        n332 = Number To Decimal String(number=w1497) -> (decimal integer string=w1532:string)  [unwired: 1 in]
        n333 = Concatenate Strings(w1531, "logfile" ("Substring"), w1532, w1495, ".txt" ("Substring")) -> (w1529:string)
        n334 = String To Path(string=w1529) -> (path=w1502:path)
        n335 = Unbundle(w1528) -> ("integration time"=w1527:u32, "Short/Long integration time"=w1526:dbl, "hold time (sec)"=w1525:dbl, "delay time (sec)"=w1524:dbl, "Step Time (0 disables)"=w1523:dbl, "sweep method"=w1522:u16, "Pulse period"=w1521:dbl, "Base voltage"=w1520:dbl, "Pulse width"=w1519:dbl)
        n336 = Build Array(w1527, w1526, w1525, w1524, w1523, w1522, w1521, w1520, w1519, w1513, w1514, w1515, w1516, w1517, w1518) -> (w1506:dbl[])
        n337 = Insert Into Array(array=dbl[][] [] ("Input Array"), new element=w1506) -> (w1505:dbl[][])  [unwired: 2 in]
        n338 = call <vilib>:"compatOverwrite.vi"("overwrite (F)"=TRUE) -> ("overwrite?"=w1500:T8)
        n339 = Open/Create/Replace File(file path (use dialog)=w1502, error in=w1504, operation (0:open)=w1500) -> (refnum out=w1510:refnum<file>, error out=w1509:errorcluster)  [unwired: 3 in, 1 out]
        n340 = call "4155C Write array to file.vi"("Byte Stream File Refnum"=w1510, "Header"=string[] ["Int Time", "Short/Long Itime", "Hold time", "Delay time", "Step time", "Sweep method", "Pulse period", "Base Voltage", "Pulse width", "Drain compliance", "Gate compliance", "Gate range mode", "Gate range", "S/D range mode", "S/D range"], "Data Array"=w1505, "error in (no error)"=w1509) -> ("dup refnum"=w1512:refnum<file>, "error out"=w1511:errorcluster)  [unwired: 1 in]
        n341 = Close File(refnum=w1512, error in=w1511) -> (error out=w1503:errorcluster)  [unwired: 1 out]
      }
      frame "sample" {
        w1570 = 1
        # "The suffix is Vg_Vd_Time."
        # "Add a time offset (elapsed time) to the time axis."
        # "Adjusts graph colors."
        n342 = Number To Decimal String(number=w1604) -> (decimal integer string=w1642:string)  [unwired: 1 in]
        n343 = local read "Sample - Drain"() -> (w1538:u32)
        n344 = Fract/Exp String To Number(string=w1640) -> (number=w1608:dbl[])  [unwired: 3 in, 1 out]
        n345 = Index Array(array=w1608, index=0 ("Index")) -> (element=w1562:dbl)
        n346 = Index Array(array=w1608, index=2 ("Index")) -> (element=w1636:dbl)
        n347 = Index Array(array=w1608, index=3 ("Index")) -> (element=w1559:dbl)
        n348 = Index Array(array=w1608, index=4 ("Index")) -> (element=w1607:dbl)
        n349 = Index Array(array=w1608, index=1 ("Index")) -> (element=w1564:dbl)
        n350 = local read "Sample - Probe 4"() -> (w1541:u32)
        n351 = local read "Sample - Source/Common"() -> (w1539:u32)
        n352 = local read "Time Units"() -> (w1534:u16)
        n353 = local read "Sample - Gate"() -> (w1540:u32)
        n354 = call "4155C Config Sampling Measurements v2.0.vi"("VISA session"=w1645, "Num Points"=w1636, "Sample - Drain"=w1538, "Display on/off"=TRUE, "Gate Compliance"=w1623, "Sampling interval"=w1607, "Sample - Source/Common"=w1539, "Sample - Probe 4"=w1541, "Drain Compliance"=w1643, "Standby"=w1542, "error in (no error)"=w1644, "Timings"=w1615, "Sample - Gate"=w1540, "Sample time"=w1559) -> ("dup VISA resource name"=w1647:refnum<visa-resource-name>, "error out"=w1646:errorcluster)
        n355 = local read "Plot sample extrema vs time"() -> (w1572:bool)
        n356 = Number To Decimal String(number=w1564) -> (decimal integer string=w1565:string)  [unwired: 1 in]
        n357 = Number To Decimal String(number=w1562) -> (decimal integer string=w1561:string)  [unwired: 1 in]
        n358 = Number To Decimal String(number=w1559) -> (decimal integer string=w1558:string)  [unwired: 1 in]
        n359 = call "4155C Take Sample v2.0.vi"("VISA resource name in"=w1647, "Emergency Stop"=w1620, "Sample - Gate"=w1540, "Vg"=w1562, "Sample - Drain"=w1538, "Vd"=w1564, "error in (no error)"=w1646) -> ("Time"=w1535:dbl[], "VISA Resource Name out"=w1617:refnum<visa-resource-name>, "Ig"=w1552:dbl[], "Id"=w1553:dbl[], "Is"=w1554:dbl[], "error out"=w1580:errorcluster)  [unwired: 3 in]
        n360 = Insert Into Array(array=w1546, new element=w1553) -> (w1549:dbl[])  [unwired: 1 in]
        n361 = case shown="0, Default" w1534 {
          tunnel: [w1650 w1651 w1654] -> w1537
          tunnel: w1535 -> [w1649 w1651 w1653]
          frame 2 {
            n362 = Divide(x=w1649, y=3600.0) -> (x/y=w1650:dbl[])
          }
          frame 0, Default {
          }
          frame 1 {
            n363 = Divide(x=w1653, y=60.0) -> (x/y=w1654:dbl[])
          }
        }
        n364 = Insert Into Array(array=w1545, new element=w1554) -> (w1551:dbl[])  [unwired: 1 in]
        n365 = Insert Into Array(array=w1547, new element=w1552) -> (w1550:dbl[])  [unwired: 1 in]
        n366 = Concatenate Strings(w1565, "_" ("Substring"), w1561, "_" ("Substring"), w1558, ".txt" ("Substring")) -> (w1556:string)
        n367 = Concatenate Strings(w1567, w1566, w1642, w1602, "_S_" ("Substring"), w1556) -> (w1641:string)
        n368 = String To Path(string=w1641) -> (path=w1626:path)
        n369 = Add(x=w1537, y=w1536) -> (x+y=w1555:dbl[])
        n370 = Insert Into Array(array=w1544, new element=w1555) -> (w1548:dbl[])  [unwired: 1 in]
        n371 = case shown="True" w1572 {
          tunnel: w1555 -> [_ w1657]
          tunnel: [w1655 w1658] -> w1569
          tunnel: w1573 -> [w1655 w1656]
          frame False {
          }
          frame True {
            n372 = Insert Into Array(array=w1656, new element=w1657) -> (w1658:i32[])  [unwired: 1 in]
          }
        }
        n373 = case shown="True" "Plot sample extrema vs time" {
          tunnel: w1554 -> [_ w1687]
          tunnel: w1553 -> [_ w1688]
          tunnel: w1552 -> [_ w1689]
          tunnel: [w1665 w1675] -> w1543
          tunnel: w1580 -> [w1665 w1680]
          tunnel: w1586 -> [w1664 w1692]
          tunnel: w1585 -> [w1663 w1691]
          tunnel: w1584 -> [w1662 w1693]
          tunnel: w1583 -> [w1661 w1690]
          tunnel: w1582 -> [w1660 w1695]
          tunnel: w1581 -> [w1659 w1694]
          tunnel: [w1664 w1679] -> w1579
          tunnel: [w1663 w1673] -> w1578
          tunnel: [w1662 w1677] -> w1577
          tunnel: [w1661 w1672] -> w1576
          tunnel: [w1660 w1678] -> w1575
          tunnel: [w1659 w1671] -> w1574
          tunnel: w1569 -> [_ w1669]
          frame False {
          }
          frame True {
            w1674 = 1
            # "Number of VAR2 steps is 1."
            # "abs(Ig)"
            # "abs(Is)"
            # "abs(Id)"
            # "Adjusts graph colors."
            n374 = Absolute Value(x=w1689) -> (abs(x)=w1666:dbl[])
            n375 = Absolute Value(x=w1688) -> (abs(x)=w1667:dbl[])
            n376 = Absolute Value(x=w1687) -> (abs(x)=w1668:dbl[])
            n377 = Array Max & Min(array=w1668) -> (max value=w1686:dbl, min value=w1683:dbl)  [unwired: 2 out]
            n378 = Array Max & Min(array=w1667) -> (max value=w1685:dbl, min value=w1682:dbl)  [unwired: 2 out]
            n379 = Array Max & Min(array=w1666) -> (max value=w1684:dbl, min value=w1681:dbl)  [unwired: 2 out]
            n380 = local write "Id max"(w1685) -> ()
            n381 = local write "Id min"(w1682) -> ()
            n382 = local write "Ig max"(w1684) -> ()
            n383 = local write "Ig min"(w1681) -> ()
            n384 = Insert Into Array(array=w1695, new element=w1666) -> (w1678:dbl[])  [unwired: 1 in]
            n385 = Insert Into Array(array=w1694, new element=w1666) -> (w1671:dbl[])  [unwired: 1 in]
            n386 = local write "Is max"(w1686) -> ()
            n387 = local write "Is min"(w1683) -> ()
            n388 = Insert Into Array(array=w1693, new element=w1667) -> (w1677:dbl[])  [unwired: 1 in]
            n389 = Insert Into Array(array=w1690, new element=w1667) -> (w1672:dbl[])  [unwired: 1 in]
            n390 = Insert Into Array(array=w1692, new element=w1668) -> (w1679:dbl[])  [unwired: 1 in]
            n391 = Insert Into Array(array=w1691, new element=w1668) -> (w1673:dbl[])  [unwired: 1 in]
            n392 = control-ref of="Imax vs time"() -> (w1696:refnum<vi>)
            n393 = call "4155C Config Chart Colours.vi"("Numeric"=w1674, "XY Graph 2"=w1696) -> ()  [unwired: 6 in]
            n394 = call "4155C Split array.vi"("Number of VAR2 steps"=w1674, "Y2 data in"=w1677, "X data in"=w1669, "Y1 data in"=w1679, "Y3 data in"=w1678, "error in (no error)"=w1680) -> ("Array of clusters"=w1697:cluster{"Y data in":dbl[], "X data in":dbl[]}[], "error out"=w1676:errorcluster)  [unwired: 1 in]
            n395 = call "4155C Split array.vi"("Number of VAR2 steps"=w1674, "Y2 data in"=w1672, "X data in"=w1669, "Y1 data in"=w1673, "Y3 data in"=w1671, "error in (no error)"=w1676) -> ("Array of clusters"=w1670:cluster{"Y data in":dbl[], "X data in":dbl[]}[], "error out"=w1675:errorcluster)  [unwired: 1 in]
            n396 = local write "Imax vs time"(w1697) -> ()
            n397 = local write "Imin vs time"(w1670) -> ()
          }
        }
        n398 = control-ref of="I vs time (Bias Stress)"() -> (w1568:refnum<vi>)
        n399 = call "4155C Split array.vi"("Number of VAR2 steps"=w1570, "Y2 data in"=w1549, "X data in"=w1548, "Y1 data in"=w1551, "Y3 data in"=w1550) -> ("Array of clusters"=w1571:cluster{"Y data in":dbl[], "X data in":dbl[]}[])  [unwired: 2 in, 1 out]
        n400 = local write "I vs time (Bias Stress)"(w1571) -> ()
        n401 = call "4155C Config Chart Colours.vi"("Numeric"=w1570, "XY Graph 2"=w1568) -> ()  [unwired: 6 in]
        n402 = Insert Into Array(array=dbl[][] [] ("Input Array"), new element=w1555) -> (w1630:dbl[][])  [unwired: 2 in]
        n403 = Insert Into Array(array=w1630, new element=w1552) -> (w1629:dbl[][])  [unwired: 2 in]
        n404 = VISA Write(VISA resource name=w1617, write buffer=":DISP ON" ("write buffer (\"\")"), error in (no error)=w1543) -> (VISA resource name out=w1616:refnum<visa-resource-name>, error out=w1618:errorcluster)  [unwired: 1 out]
        n405 = Insert Into Array(array=w1629, new element=w1553) -> (w1628:dbl[][])  [unwired: 2 in]
        n406 = Insert Into Array(array=w1628, new element=w1554) -> (w1622:dbl[][])  [unwired: 2 in]
        n407 = call <vilib>:"compatOverwrite.vi"("overwrite (F)"=TRUE) -> ("overwrite?"=w1605:T8)
        n408 = Open/Create/Replace File(file path (use dialog)=w1626, error in=w1618, operation (0:open)=w1605) -> (refnum out=w1633:refnum<file>, error out=w1632:errorcluster)  [unwired: 3 in, 1 out]
        n409 = Transpose 2D Array(2D array=w1622) -> (transposed array=w1621:dbl[][])
        n410 = call "4155C Write array to file.vi"("Byte Stream File Refnum"=w1633, "Header"=string[] ["Time /Units", "Ig /A", "Id /A", "Is /A"], "Data Array"=w1621, "error in (no error)"=w1632) -> ("dup refnum"=w1635:refnum<file>, "error out"=w1634:errorcluster)  [unwired: 1 in]
        n411 = Close File(refnum=w1635, error in=w1634) -> (error out=w1624:errorcluster)  [unwired: 1 out]
      }
      frame "samplei" {
        n412 = Number To Decimal String(number=w1729) -> (decimal integer string=w1780:string)  [unwired: 1 in]
        n413 = local read "Sample I - Source/Common"() -> (w1698:u32)
        n414 = local read "Sample I - Probe 4 (Disabled)"() -> (w1701:u32)
        n415 = Concatenate Strings(w1759, "-samplei-" ("Substring"), w1780, w1728, ".txt" ("Substring")) -> (w1778:string)
        n416 = Fract/Exp String To Number(string=w1777) -> (number=w1744:dbl[])  [unwired: 3 in, 1 out]
        n417 = String To Path(string=w1778) -> (path=w1762:path)
        n418 = Index Array(array=w1744, index=4 ("Index")) -> (element=w1738:dbl)
        n419 = Index Array(array=w1744, index=3 ("Index")) -> (element=w1739:dbl)
        n420 = Index Array(array=w1744, index=1 ("Index")) -> (element=w1741:dbl)
        n421 = Index Array(array=w1744, index=0 ("Index")) -> (element=w1742:dbl)
        n422 = local read "Sample I - Drain/Gate"() -> (w1700:u32)
        n423 = Index Array(array=w1744, index=2 ("Index")) -> (element=w1740:dbl)
        n424 = local read "Sample I - Probe 3 (Disabled)"() -> (w1699:u32)
        n425 = call "4155C Config SamplingI Measurements v2.0.vi"("VISA session"=w1783, "Num Points"=w1741, "Sample I - Probe 3 (Disabled)"=w1699, "Display on/off"=TRUE, "Sample I - Source/Common"=w1698, "Sample I - Drain/Gate"=w1700, "Sampling interval"=w1739, "Standby"=w1702, "error in (no error)"=w1782, "Timings"=w1751, "Sample I - Probe 4 (Disabled)"=w1701, "Sample time"=w1740) -> ("dup VISA resource name"=w1785:refnum<visa-resource-name>, "error out"=w1784:errorcluster)  [unwired: 2 in]
        n426 = call "4155C Take SampleI v2.0.vi"("Sample I - Drain/Gate"=w1700, "Emergency Stop"=w1756, "error in (no error)"=w1784, "Idg 2"=w1742, "Vdg compliance 2"=w1738, "VISA resource name in"=w1785) -> ("error out"=w1754:errorcluster, "Idg"=w1787:dbl[], "Vdg"=w1764:dbl[], "VISA Resource Name out"=w1752:refnum<visa-resource-name>, "Is"=w1786:dbl[], "Time"=w1768:dbl[])
        n427 = Insert Into Array(array=dbl[][] [] ("Input Array"), new element=w1768) -> (w1767:dbl[][])  [unwired: 2 in]
        n428 = Insert Into Array(array=w1767, new element=w1764) -> (w1766:dbl[][])  [unwired: 2 in]
        n429 = Insert Into Array(array=w1766, new element=w1787) -> (w1765:dbl[][])  [unwired: 2 in]
        n430 = VISA Write(VISA resource name=w1752, write buffer=":DISP ON" ("write buffer (\"\")"), error in (no error)=w1754) -> (VISA resource name out=w1737:refnum<visa-resource-name>, error out=w1753:errorcluster)  [unwired: 1 out]
        n431 = Insert Into Array(array=w1765, new element=w1786) -> (w1758:dbl[][])  [unwired: 2 in]
        n432 = call <vilib>:"compatOverwrite.vi"("overwrite (F)"=TRUE) -> ("overwrite?"=w1732:T8)
        n433 = Open/Create/Replace File(file path (use dialog)=w1762, error in=w1753, operation (0:open)=w1732) -> (refnum out=w1771:refnum<file>, error out=w1770:errorcluster)  [unwired: 3 in, 1 out]
        n434 = Transpose 2D Array(2D array=w1758) -> (transposed array=w1757:dbl[][])
        n435 = call "4155C Write array to file.vi"("Byte Stream File Refnum"=w1771, "Header"=string[] ["Time /s", "Vdg /V", "Idg /A", "Is /A"], "Data Array"=w1757, "error in (no error)"=w1770) -> ("dup refnum"=w1773:refnum<file>, "error out"=w1772:errorcluster)  [unwired: 1 in]
        n436 = Close File(refnum=w1773, error in=w1772) -> (error out=w1735:errorcluster)  [unwired: 1 out]
        n437 = VISA Write(VISA resource name=w1737, write buffer=";:PAGE:SCON:STAN OFF;:PAGE:CHAN:VSU2:DIS;" ("write buffer (\"\")"), error in (no error)=w1735) -> (VISA resource name out=w1733:refnum<visa-resource-name>, error out=w1734:errorcluster)  [unwired: 1 out]
      }
      frame "#" {
        n438 = VISA Write(VISA resource name=w1818, write buffer=":DISP ON" ("write buffer (\"\")"), error in (no error)=w1817) -> (VISA resource name out=w1816:refnum<visa-resource-name>, error out=w1815:errorcluster)  [unwired: 1 out]
      }
      frame "stressV" {
        n439 = Number To Decimal String(number=w1855) -> (decimal integer string=w1896:string)  [unwired: 1 in]
        n440 = Concatenate Strings(w1880, "-stressV-" ("Substring"), w1896, w1854, ".txt" ("Substring")) -> (w1894:string)
        n441 = Fract/Exp String To Number(string=w1893) -> (number=w1866:dbl[])  [unwired: 3 in, 1 out]
        n442 = local read "Stress V - Source/Common"() -> (w1829:u32)
        n443 = String To Path(string=w1894) -> (path=w1884:path)
        n444 = Index Array(array=w1866, index=3 ("Index")) -> (element=w1863:dbl)
        n445 = Index Array(array=w1866, index=1 ("Index")) -> (element=w1861:dbl)
        n446 = Index Array(array=w1866, index=0 ("Index")) -> (element=w1860:dbl)
        n447 = Index Array(array=w1866, index=4 ("Index")) -> (element=w1865:dbl)
        n448 = Index Array(array=w1866, index=2 ("Index")) -> (element=w1862:dbl)
        n449 = local read "Stress V - Drain"() -> (w1828:u32)
        n450 = local read "Stress V - Gate"() -> (w1827:u32)
        n451 = call "4155C Config V Stress v2.0.vi"("Display on/off"=TRUE, "Stress V - Gate"=w1827, "Stress V - Drain"=w1828, "Stress V - Source/Common"=w1829, "IG compliance"=w1862, "ID compliance"=w1863, "error in (no error)"=w1898, "VG"=w1860, "VD"=w1861, "VISA session"=w1899) -> ("error out"=w1900:errorcluster, "dup VISA resource name"=w1901:refnum<visa-resource-name>)
        n452 = call "4155C Apply Stress.vi"("error in (no error)"=w1900, "Duration"=w1865, "Emergency Stop"=w1879, "VISA resource name in"=w1901) -> ("error out"=w1877:errorcluster, "VISA Resource Name out"=w1875:refnum<visa-resource-name>)
        n453 = VISA Write(VISA resource name=w1875, write buffer=":DISP ON" ("write buffer (\"\")"), error in (no error)=w1877) -> (VISA resource name out=w1874:refnum<visa-resource-name>, error out=w1876:errorcluster)  [unwired: 1 out]
        n454 = call <vilib>:"compatOverwrite.vi"("overwrite (F)"=TRUE) -> ("overwrite?"=w1859:T8)
        n455 = Open/Create/Replace File(file path (use dialog)=w1884, error in=w1876, operation (0:open)=w1859) -> (refnum out=w1887:refnum<file>, error out=w1886:errorcluster)  [unwired: 3 in, 1 out]
        n456 = call "4155C Write array to file.vi"("Byte Stream File Refnum"=w1887, "Header"=string[] ["V stress completed successfully", ""], "error in (no error)"=w1886) -> ("dup refnum"=w1889:refnum<file>, "error out"=w1888:errorcluster)  [unwired: 2 in]
        n457 = Close File(refnum=w1889, error in=w1888) -> (error out=w1882:errorcluster)  [unwired: 1 out]
      }
      frame "stressI" {
        n458 = local read "Stress I - Source/Common"() -> (w1902:u32)
        n459 = Number To Decimal String(number=w1929) -> (decimal integer string=w1966:string)  [unwired: 1 in]
        n460 = Concatenate Strings(w1950, "-stressI-" ("Substring"), w1966, w1928, ".txt" ("Substring")) -> (w1964:string)
        n461 = Fract/Exp String To Number(string=w1963) -> (number=w1938:dbl[])  [unwired: 3 in, 1 out]
        n462 = Index Array(array=w1938, index=1 ("Index")) -> (element=w1934:dbl)
        n463 = Index Array(array=w1938, index=0 ("Index")) -> (element=w1935:dbl)
        n464 = Index Array(array=w1938, index=2 ("Index")) -> (element=w1936:dbl)
        n465 = String To Path(string=w1964) -> (path=w1954:path)
        n466 = local read "Stress I - Drain/Gate"() -> (w1903:u32)
        n467 = call "4155C Config I Stress v2.0.vi"("Stress I - Drain/Gate"=w1903, "Stress I - Source/Common"=w1902, "Display on/off"=TRUE, "error in (no error)"=w1968, "VDG compliance"=w1934, "IDG"=w1935, "VISA session"=w1969) -> ("error out"=w1970:errorcluster, "dup VISA resource name"=w1971:refnum<visa-resource-name>)  [unwired: 1 in]
        n468 = call "4155C Apply Stress.vi"("error in (no error)"=w1970, "Duration"=w1936, "Emergency Stop"=w1949, "VISA resource name in"=w1971) -> ("error out"=w1947:errorcluster, "VISA Resource Name out"=w1945:refnum<visa-resource-name>)
        n469 = VISA Write(VISA resource name=w1945, write buffer=":DISP ON" ("write buffer (\"\")"), error in (no error)=w1947) -> (VISA resource name out=w1944:refnum<visa-resource-name>, error out=w1946:errorcluster)  [unwired: 1 out]
        n470 = call <vilib>:"compatOverwrite.vi"("overwrite (F)"=TRUE) -> ("overwrite?"=w1933:T8)
        n471 = Open/Create/Replace File(file path (use dialog)=w1954, error in=w1946, operation (0:open)=w1933) -> (refnum out=w1957:refnum<file>, error out=w1956:errorcluster)  [unwired: 3 in, 1 out]
        n472 = call "4155C Write array to file.vi"("Byte Stream File Refnum"=w1957, "Header"=string[] ["I stress completed successfully", ""], "error in (no error)"=w1956) -> ("dup refnum"=w1959:refnum<file>, "error out"=w1958:errorcluster)  [unwired: 2 in]
        n473 = Close File(refnum=w1959, error in=w1958) -> (error out=w1952:errorcluster)  [unwired: 1 out]
      }
      frame "vsu2pulse" {
        n474 = Number To Decimal String(number=w1998) -> (decimal integer string=w2033:string)  [unwired: 1 in]
        n475 = Concatenate Strings(w2018, "-vsu2-" ("Substring"), w2033, w1997, ".txt" ("Substring")) -> (w2031:string)
        n476 = Fract/Exp String To Number(string=w2030) -> (number=w2006:dbl[])  [unwired: 3 in, 1 out]
        n477 = String To Path(string=w2031) -> (path=w2022:path)
        n478 = Index Array(array=w2006, index=1 ("Index")) -> (element=w2005:dbl)
        n479 = Index Array(array=w2006, index=0 ("Index")) -> (element=w2003:dbl)
        n480 = local read "VSU2 Stress - Source/Common"() -> (w1972:u32)
        n481 = call "4155C Config VSU2 Stress v2.0.vi"("VISA session"=w2036, "Display on/off"=TRUE, "VSU2"=w2003, "error in (no error)"=w2035, "VSU2 Stress - Source/Common"=w1972) -> ("dup VISA resource name"=w2038:refnum<visa-resource-name>, "error out"=w2037:errorcluster)
        n482 = call "4155C Apply Stress.vi"("error in (no error)"=w2037, "Duration"=w2005, "Emergency Stop"=w2017, "VISA resource name in"=w2038) -> ("error out"=w2015:errorcluster, "VISA Resource Name out"=w2013:refnum<visa-resource-name>)
        n483 = VISA Write(VISA resource name=w2013, write buffer=":DISP ON" ("write buffer (\"\")"), error in (no error)=w2015) -> (VISA resource name out=w2012:refnum<visa-resource-name>, error out=w2014:errorcluster)  [unwired: 1 out]
        n484 = call <vilib>:"compatOverwrite.vi"("overwrite (F)"=TRUE) -> ("overwrite?"=w2002:T8)
        n485 = Open/Create/Replace File(file path (use dialog)=w2022, error in=w2014, operation (0:open)=w2002) -> (refnum out=w2025:refnum<file>, error out=w2024:errorcluster)  [unwired: 3 in, 1 out]
        n486 = call "4155C Write array to file.vi"("Byte Stream File Refnum"=w2025, "Header"=string[] ["VSU2 pulse completed successfully", ""], "error in (no error)"=w2024) -> ("dup refnum"=w2027:refnum<file>, "error out"=w2026:errorcluster)  [unwired: 2 in]
        n487 = Close File(refnum=w2027, error in=w2026) -> (error out=w2020:errorcluster)  [unwired: 1 out]
      }
      frame "sample-fpp" {
        w2080 = string[] ["Time /s", "Id VgVd /A", "Ig VgVd /A", "Vp1 VgVd /V", "Vp2 VgVd /V"] ("Header")
        w2084 = "%d" ("format string")
        n488 = Number To Decimal String(number=w2070) -> (decimal integer string=w2132:string)  [unwired: 1 in]
        n489 = Fract/Exp String To Number(string=w2129) -> (number=w2117:dbl[])  [unwired: 3 in, 1 out]
        n490 = Concatenate Strings(w2123, "-samplefpp-" ("Substring"), w2132, w2069, ".txt" ("Substring")) -> (w2130:string)
        n491 = local read "FPP - Source"() -> (w2039:u32)
        n492 = local read "FPP - Drain"() -> (w2040:u32)
        n493 = local read "FPP - Gate"() -> (w2041:u32)
        n494 = local read "FPP - Probe 1"() -> (w2042:u32)
        n495 = String To Path(string=w2130) -> (path=w2092:path)
        n496 = Index Array(array=w2117, index=0 ("Index")) -> (element=w2079:dbl)
        n497 = Index Array(array=w2117, index=1 ("Index")) -> (element=w2078:dbl)
        n498 = Index Array(array=w2117, index=2 ("Index")) -> (element=w2125:dbl)
        n499 = Index Array(array=w2117, index=3 ("Index")) -> (element=w2115:dbl)
        n500 = Number To Decimal String(number=w2079) -> (decimal integer string=w2104:string)  [unwired: 1 in]
        n501 = local read "FPP - Probe 2"() -> (w2043:u32)
        n502 = call "4155C Config Sampling Measurements FPP v2.0.vi"("VISA session"=w2135, "Gate Compliance"=w2124, "FPP - Source"=w2039, "FPP - Drain"=w2040, "Drain Compliance"=w2133, "error in (no error)"=w2134, "Num Points"=w2125, "Timings"=w2122, "FPP - Gate"=w2041, "FPP - Probe 1"=w2042, "Vg"=w2079, "Vd"=w2078, "Display on/off"=TRUE, "Sample time"=w2115, "FPP - Probe 2"=w2043, "Standby"=w2044) -> ("dup VISA resource name"=w2094:refnum<visa-resource-name>, "error out"=w2093:errorcluster)  [unwired: 2 in]
        n503 = call "4155C Take Sample FPP.vi"("VISA resource name in"=w2094, "error in (no error)"=w2093, "Emergency Stop"=w2095) -> ("Time"=w2099:dbl[], "Vp1"=w2109:dbl[], "VISA Resource Name out"=w2076:refnum<visa-resource-name>, "Ig"=w2097:dbl[], "Id"=w2098:dbl[], "Vp2"=w2107:dbl[], "error out"=w2096:errorcluster)  [unwired: 10 in]
        n504 = Insert Into Array(array=dbl[][] [] ("Input Array"), new element=w2099) -> (w2113:dbl[][])  [unwired: 2 in]
        n505 = Number To Decimal String(number=w2078) -> (decimal integer string=w2102:string)  [unwired: 1 in]
        n506 = Insert Into Array(array=w2113, new element=w2098) -> (w2112:dbl[][])  [unwired: 2 in]
        n507 = Concatenate Strings("(Vg = " ("Substring"), w2104, "V, Vd = " ("Substring"), w2102, "V)" ("Substring")) -> (w2100:string)
        n508 = Insert Into Array(array=w2112, new element=w2097) -> (w2111:dbl[][])  [unwired: 2 in]
        n509 = Insert Into Array(array=w2111, new element=w2109) -> (w2108:dbl[][])  [unwired: 2 in]
        n510 = Insert Into Array(array=w2108, new element=w2107) -> (w2077:dbl[][])  [unwired: 2 in]
        n511 = Transpose 2D Array(2D array=w2077) -> (transposed array=w2106:dbl[][])
        n512 = call <vilib>:"compatOverwrite.vi"("overwrite (F)"=TRUE) -> ("overwrite?"=w2074:T8)
        n513 = Open/Create/Replace File(file path (use dialog)=w2092, error in=w2096, operation (0:open)=w2074) -> (refnum out=w2089:refnum<file>, error out=w2090:errorcluster)  [unwired: 3 in, 1 out]
        n514 = Array To Spreadsheet String(array=w2080, 3:w2084) -> (spreadsheet string=w2086:string)  [unwired: 1 in]
        n515 = Search and Replace String(replace all?=TRUE ("replace all? (F)"), input string=w2086, search string="VgVd", replace string=w2100) -> (result string=w2082:string)  [unwired: 4 in, 3 out]
        n516 = Spreadsheet String To Array(format string=w2084, spreadsheet string=w2082, array type (2D Dbl)=w2080) -> (array=w2081:string[])  [unwired: 1 in]
        n517 = call "4155C Write array to file.vi"("Byte Stream File Refnum"=w2089, "Header"=w2081, "Data Array"=w2106, "error in (no error)"=w2090) -> ("dup refnum"=w2087:refnum<file>, "error out"=w2088:errorcluster)  [unwired: 1 in]
        n518 = Close File(refnum=w2087, error in=w2088) -> (error out=w2075:errorcluster)  [unwired: 1 out]
      }
      frame "resample-fpp" {
        w2174 = string[] ["Time /s", "Id VgVd /A", "Ig VgVd /A", "Vp1 VgVd /V", "Vp2 VgVd /V"] ("Header")
        w2178 = "%d" ("format string")
        n519 = Number To Decimal String(number=w2160) -> (decimal integer string=w2218:string)  [unwired: 1 in]
        n520 = Fract/Exp String To Number(string=w2215) -> (number=w2167:dbl[])  [unwired: 3 in, 1 out]
        n521 = Concatenate Strings(w2211, "-resamplefpp-" ("Substring"), w2218, w2161, ".txt" ("Substring")) -> (w2216:string)
        n522 = String To Path(string=w2216) -> (path=w2186:path)
        n523 = Index Array(array=w2167, index=0 ("Index")) -> (element=w2173:dbl)
        n524 = Index Array(array=w2167, index=1 ("Index")) -> (element=w2172:dbl)
        n525 = Number To Decimal String(number=w2173) -> (decimal integer string=w2196:string)  [unwired: 1 in]
        n526 = call "4155C Take Sample FPP.vi"("VISA resource name in"=w2169, "error in (no error)"=w2168, "Emergency Stop"=w2187) -> ("Time"=w2191:dbl[], "Vp1"=w2201:dbl[], "VISA Resource Name out"=w2171:refnum<visa-resource-name>, "Ig"=w2189:dbl[], "Id"=w2190:dbl[], "Vp2"=w2199:dbl[], "error out"=w2188:errorcluster)  [unwired: 10 in]
        n527 = Insert Into Array(array=dbl[][] [] ("Input Array"), new element=w2191) -> (w2205:dbl[][])  [unwired: 2 in]
        n528 = Number To Decimal String(number=w2172) -> (decimal integer string=w2194:string)  [unwired: 1 in]
        n529 = Insert Into Array(array=w2205, new element=w2190) -> (w2204:dbl[][])  [unwired: 2 in]
        n530 = Concatenate Strings("(Vg = " ("Substring"), w2196, "V, Vd = " ("Substring"), w2194, "V)" ("Substring")) -> (w2192:string)
        n531 = Insert Into Array(array=w2204, new element=w2189) -> (w2203:dbl[][])  [unwired: 2 in]
        n532 = Insert Into Array(array=w2203, new element=w2201) -> (w2200:dbl[][])  [unwired: 2 in]
        n533 = Insert Into Array(array=w2200, new element=w2199) -> (w2166:dbl[][])  [unwired: 2 in]
        n534 = call <vilib>:"compatOverwrite.vi"("overwrite (F)"=TRUE) -> ("overwrite?"=w2165:T8)
        n535 = Open/Create/Replace File(file path (use dialog)=w2186, error in=w2188, operation (0:open)=w2165) -> (refnum out=w2183:refnum<file>, error out=w2184:errorcluster)  [unwired: 3 in, 1 out]
        n536 = Array To Spreadsheet String(array=w2174, 3:w2178) -> (spreadsheet string=w2180:string)  [unwired: 1 in]
        n537 = Transpose 2D Array(2D array=w2166) -> (transposed array=w2198:dbl[][])
        n538 = Search and Replace String(replace all?=TRUE ("replace all? (F)"), input string=w2180, search string="VgVd", replace string=w2192) -> (result string=w2176:string)  [unwired: 4 in, 3 out]
        n539 = Spreadsheet String To Array(format string=w2178, spreadsheet string=w2176, array type (2D Dbl)=w2174) -> (array=w2175:string[])  [unwired: 1 in]
        n540 = call "4155C Write array to file.vi"("Byte Stream File Refnum"=w2183, "Header"=w2175, "Data Array"=w2198, "error in (no error)"=w2184) -> ("dup refnum"=w2181:refnum<file>, "error out"=w2182:errorcluster)  [unwired: 1 in]
        n541 = Close File(refnum=w2181, error in=w2182) -> (error out=w2170:errorcluster)  [unwired: 1 out]
      }
      frame "serial" {
        n542 = local read "Termination char\n(0xA = '\\n' = LF)\n(0xD = '\\r' = CR)"() -> (w2251:u8)
        n543 = local read "Enable Termination\nChar (T)"() -> (w2252:bool)
        n544 = Index Array(array=w2259, index=0 ("Index")) -> (element=w2258:string)
        n545 = local read "parity"() -> (w2242:u16)
        n546 = local read "Delay before read (ms)"() -> (w2253:u32)
        n547 = local read "byte count"() -> (w2250:u32)
        n548 = local read "Timeout (ms)"() -> (w2249:u32)
        n549 = local read "VISA resource name"() -> (w2246:refnum<visa-resource-name>)
        n550 = local read "baud rate"() -> (w2245:u32)
        n551 = local read "Serial End Mode for Reads"() -> (w2244:u16)
        n552 = local read "data bits"() -> (w2243:u16)
        n553 = local read "stop bits"() -> (w2248:u16)
        n554 = local read "flow control"() -> (w2247:u16)
        n555 = call "Serial write and read v0.5.vi"("Delay before read (ms)"=w2253, "Termination char\n(0xA = '\\n' = LF)\n(0xD = '\\r' = CR)"=w2251, "Enable Termination\nChar (T)"=w2252, "parity"=w2242, "stop bits"=w2248, "string to write"=w2258, "flow control"=w2247, "byte count"=w2250, "Serial Settings:Serial End Mode for Reads"=w2244, "Timeout (ms)"=w2249, "error in (no error)"=w2264, "VISA resource name"=w2246, "baud rate"=w2245, "data bits"=w2243) -> ("Serial port output"=w2254:string, "error out"=w2263:errorcluster)
        n556 = Build Array (concatenate)(w2254, w2255) -> (w2256:string[])
      }
      frame "pump" {
        # "Time array for valve position"
        # "Time array for absolute plunger position"
        # "Valve position"
        # "Absolute plunger position"
        # "Remove \"_\""
        # "Check if hard stop is pressed."
        # "Check if halt is pressed."
        # "Check if pump is idle. Else halt."
        n557 = Index Array(array=w2334, index=0 ("Index")) -> (element=w2311:string)
        n558 = case shown="\"No error\", Default" w2309 {
          tunnel: w2311 -> [w2370 _ w2372 w2373 w2374 w2375 _ _ w2378 w2379 _]
          tunnel: [w2370 "/1H" w2372 w2373 w2374 w2375 "/1H" "/1H" w2378 w2379 "/1H"] -> w2310
          frame "No error", Default {
          }
          frame "Initialization" {
          }
          frame "Invalid command" {
          }
          frame "Invalid operand" {
          }
          frame "Device not initialized" {
          }
          frame "Internal failure" {
          }
          frame "Plunger overload" {
          }
          frame "Valve overload" {
          }
          frame "Plunger move not allowed" {
          }
          frame "A/D converter failure" {
          }
          frame "Command overflow" {
          }
        }
        n559 = local read "Hard stop pump"() -> (w2313:bool)
        n560 = local read "Halt pump"() -> (w2316:bool)
        n561 = local read "Serial End Mode for Reads"() -> (w2322:u16)
        n562 = local read "flow control"() -> (w2325:u16)
        n563 = local read "stop bits"() -> (w2326:u16)
        n564 = local read "parity"() -> (w2320:u16)
        n565 = local read "Delay before read (ms)"() -> (w2331:u32)
        n566 = local read "byte count"() -> (w2328:u32)
        n567 = local read "Timeout (ms)"() -> (w2327:u32)
        n568 = local read "VISA resource name"() -> (w2324:refnum<visa-resource-name>)
        n569 = local read "baud rate"() -> (w2323:u32)
        n570 = local read "Enable Termination\nChar (T)"() -> (w2330:bool)
        n571 = local read "Termination char\n(0xA = '\\n' = LF)\n(0xD = '\\r' = CR)"() -> (w2329:u8)
        n572 = case shown="True" w2316 {
          tunnel: [w2384 "/1H"] -> w2315
          tunnel: w2310 -> [w2384 _]
          frame False {
          }
          frame True {
            n573 = local write "Halt pump"(FALSE) -> ()
          }
        }
        n574 = case shown="True" w2313 {
          tunnel: [w2381 "/1T"] -> w2314
          tunnel: w2315 -> [w2381 _]
          frame False {
          }
          frame True {
            n575 = local write "Hard stop pump"(FALSE) -> ()
          }
        }
        n576 = local read "data bits"() -> (w2321:u16)
        n577 = String Subset(string=w2305, offset (0)=1) -> (substring=w2303:string)  [unwired: 1 in]
        n578 = call "SPM Pump v0.6.vi"("Termination char\n(0xA = '\\n' = LF)\n(0xD = '\\r' = CR)"=w2329, "Enable Termination\nChar (T)"=w2330, "Timeout (ms)"=w2327, "Serial Settings:Serial End Mode for Reads"=w2322, "byte count"=w2328, "Delay before read (ms)"=w2331, "Time <input>"=w2308, "error in (no error)"=w2339, "Serial port input"=w2314, "VISA resource name"=w2324, "parity"=w2320, "baud rate"=w2323, "stop bits"=w2326, "data bits"=w2321, "flow control"=w2325, "Time units <input>"=w2303) -> ("Input command"=w2302:string, "Serial port data"=w2292:string[], "Pump status"=w2298:string, "Valve position"=w2300:i32, "Absolute plunger position"=w2312:i32, "Serial port"=w2307:string, "error out"=w2338:errorcluster)  [unwired: 1 in, 4 out]
        n579 = case shown="\"?6\"" w2302 {
          tunnel: [w2351 w2359 w2365] -> w2319
          tunnel: w2318 -> [w2351 w2358 w2365]
          tunnel: w2312 -> [_ w2357 _]
          tunnel: w2299 -> [w2350 w2356 w2366]
          tunnel: [w2350 w2356 w2368] -> w2301
          tunnel: w2300 -> [_ _ w2367]
          tunnel: w2297 -> [_ w2355 w2363]
          tunnel: w2296 -> [w2349 w2354 w2364]
          tunnel: [w2349 w2353 w2364] -> w2295
          tunnel: [w2348 w2352 w2362] -> w2294
          tunnel: w2293 -> [w2348 w2352 w2361]
          frame "Q", Default {
          }
          frame "?" {
            n580 = Build Array (concatenate)(w2358, w2357) -> (w2359:i32[])
            n581 = Build Array (concatenate)(w2354, w2355) -> (w2353:i32[])
            n582 = call "4155C Split array.vi"("X data in"=w2353, "Y1 data in"=w2359) -> ("Array of clusters"=w2360:cluster{"Y data in":dbl[], "X data in":dbl[]}[])  [unwired: 5 in, 1 out]
            n583 = local write "Absolute plunger position vs time"(w2360) -> ()
          }
          frame "?6" {
            n584 = Build Array (concatenate)(w2366, w2367) -> (w2368:i32[])
            n585 = Build Array (concatenate)(w2361, w2363) -> (w2362:i32[])
            n586 = call "4155C Split array.vi"("X data in"=w2362, "Y1 data in"=w2368) -> ("Array of clusters"=w2369:cluster{"Y data in":dbl[], "X data in":dbl[]}[])  [unwired: 5 in, 1 out]
            n587 = local write "Valve position vs time"(w2369) -> ()
          }
        }
        n588 = Build Array (concatenate)(w2290, w2292) -> (w2291:string[][])
        n589 = Build Array (concatenate)(w2306, w2307) -> (w2332:string[])
      }
      frame "filename" {
        n590 = Index Array(array=w2393, index=0 ("Index")) -> (element=w2392:string)
      }
    }
    n591 = local read "Time Units"() -> (w103:u16)
    n592 = case shown="0" w103 {
      tunnel: ["Time (Seconds)" ("element") "Time (Minutes)" ("element") "Time (Hours)" ("element")] -> w69
      frame 0 {
      }
      frame 1, Default {
      }
      frame 2 {
      }
    }
    n593 = Build Array(w177, w110, w120, w119, w118, w117, w116, w115, w114, w113, w112, w111, w109) -> (w215:dbl[][])
    n594 = Transpose 2D Array(2D array=w215) -> (transposed array=w214:dbl[][])
    n595 = Concatenate Strings(w76, w75, "Imax_Imin_Ion_Ioff_vs_time.txt" ("Suffix (Imax,Imin,Ion,Ioff)")) -> (w225:string)
    n596 = Build Array(w69, "Is max (A)" ("VAR2 Name"), "Is min (A)" ("VAR2 Name"), "Id max (A)" ("VAR2 Name"), "Id min (A)" ("VAR2 Name"), "Ig max (A)" ("VAR2 Name"), "Ig min (A)" ("VAR2 Name"), "Is on (A)" ("VAR2 Name"), "Is off (A)" ("VAR2 Name"), "Id on (A)" ("VAR2 Name"), "Id off (A)" ("VAR2 Name"), "Ig on (A)" ("VAR2 Name"), "Ig off (A)" ("VAR2 Name")) -> (w220:string[])
    n597 = Array To Spreadsheet String(array=w214, 3:"%e" ("format string")) -> (spreadsheet string=w218:string)  [unwired: 1 in]
    n598 = Array To Spreadsheet String(array=w220, 3:"" ("format string")) -> (spreadsheet string=w219:string)  [unwired: 1 in]
    n599 = String To Path(string=w225) -> (path=w224:path)
    n600 = Build Array(w219, w218) -> (w217:string[])
    n601 = Write to Text File(file (use dialog)=w224, text=w217, error in=w174) -> (refnum out=w226:refnum<file>, error out=w216:errorcluster)  [unwired: 1 in, 1 out]
    n602 = Close File(refnum=w226, error in=w216) -> (error out=w158:errorcluster)  [unwired: 1 out]
    n603 = Build Array(w155, w178) -> (w183:i32[][])
    n604 = Build Array(w69, "Absolute plunger position" ("VAR2 Name")) -> (w186:string[])
    n605 = Transpose 2D Array(2D array=w183) -> (transposed array=w176:i32[][])
    n606 = Array To Spreadsheet String(array=w186, 3:"" ("format string")) -> (spreadsheet string=w185:string)  [unwired: 1 in]
    n607 = Array To Spreadsheet String(array=w176, 3:"%e" ("format string")) -> (spreadsheet string=w182:string)  [unwired: 1 in]
    n608 = Build Array(w185, w182) -> (w188:string[])
    n609 = Concatenate Strings(w76, w75, "plunger_vs_time.txt" ("Suffix (plunger)")) -> (w180:string)
    n610 = String To Path(string=w180) -> (path=w179:path)
    n611 = Write to Text File(file (use dialog)=w179, text=w188, error in=w158) -> (refnum out=w181:refnum<file>, error out=w190:errorcluster)  [unwired: 1 in, 1 out]
    n612 = Close File(refnum=w181, error in=w190) -> (error out=w157:errorcluster)  [unwired: 1 out]
    n613 = Concatenate Strings(w76, w75, "serial_port_output.txt" ("Suffix (serial port log)")) -> (w196:string)
    n614 = String To Path(string=w196) -> (path=w195:path)
    n615 = Build Array(w69, "Serial port input" ("VAR2 Name"), "Pump status" ("VAR2 Name"), "Serial port output: ") -> (w145:string[])
    n616 = Array To Spreadsheet String(array=w151, 3:"" ("format string")) -> (spreadsheet string=w142:string)  [unwired: 1 in]
    n617 = Array To Spreadsheet String(array=w145, 3:"" ("format string")) -> (spreadsheet string=w143:string)  [unwired: 1 in]
    n618 = Array To Spreadsheet String(array=w150, 3:"" ("format string")) -> (spreadsheet string=w201:string)  [unwired: 1 in]
    n619 = Build Array(w143, w142) -> (w144:string[])
    n620 = Write to Text File(file (use dialog)=w195, text=w144, error in=w157) -> (refnum out=w197:refnum<file>, error out=w198:errorcluster)  [unwired: 1 in, 1 out]
    n621 = local write "Serial port data"(w201) -> ()
    n622 = Close File(refnum=w197, error in=w198) -> (error out=w156:errorcluster)  [unwired: 1 out]
    n623 = Build Array(w154, w160) -> (w166:i32[][])
    n624 = Build Array(w69, "Valve port" ("VAR2 Name")) -> (w169:string[])
    n625 = Transpose 2D Array(2D array=w166) -> (transposed array=w161:i32[][])
    n626 = Array To Spreadsheet String(array=w169, 3:"" ("format string")) -> (spreadsheet string=w168:string)  [unwired: 1 in]
    n627 = Array To Spreadsheet String(array=w161, 3:"%e" ("format string")) -> (spreadsheet string=w165:string)  [unwired: 1 in]
    n628 = Build Array(w168, w165) -> (w171:string[])
    n629 = Concatenate Strings(w76, w75, "valve_port_vs_time.txt" ("Suffix (valve)")) -> (w163:string)
    n630 = String To Path(string=w163) -> (path=w162:path)
    n631 = Write to Text File(file (use dialog)=w162, text=w171, error in=w156) -> (refnum out=w164:refnum<file>, error out=w173:errorcluster)  [unwired: 1 in, 1 out]
    n632 = Close File(refnum=w164, error in=w173) -> (error out=w78:errorcluster)  [unwired: 1 out]
    n633 = Build Array(w74, w73, w72, w71) -> (w87:dbl[][])
    n634 = Build Array(w69, "Is (A)" ("VAR2 Name"), "Id (A)" ("VAR2 Name"), "Ig (A)" ("VAR2 Name")) -> (w83:string[])
    n635 = Transpose 2D Array(2D array=w87) -> (transposed array=w86:dbl[][])
    n636 = Concatenate Strings(w76, w75, "sample_vs_time.txt" ("Suffix (Imax,Imin,Ion,Ioff)")) -> (w93:string)
    n637 = Array To Spreadsheet String(array=w83, 3:"" ("format string")) -> (spreadsheet string=w82:string)  [unwired: 1 in]
    n638 = Array To Spreadsheet String(array=w86, 3:"%e" ("format string")) -> (spreadsheet string=w90:string)  [unwired: 1 in]
    n639 = String To Path(string=w93) -> (path=w92:path)
    n640 = Build Array(w82, w90) -> (w89:string[])
    n641 = Write to Text File(file (use dialog)=w92, text=w89, error in=w78) -> (refnum out=w94:refnum<file>, error out=w88:errorcluster)  [unwired: 1 in, 1 out]
    n642 = Close File(refnum=w94, error in=w88) -> (error out=w77:errorcluster)  [unwired: 1 out]
  }
  "error out" <- w32
  "Timings Indicator" <- w17
  "Probe 4 Indicator" <- w3
  "Is max" <- w15
  "Id max" <- w15
  "Ig max" <- w15
  "Imax vs time" <- w1
  "I vs Vg" <- w1
  "Imin vs time" <- w1
  "I vs Vd" <- w1
  "Serial port data" <- "" ("Serial port data")
  "Valve position vs time" <- cluster{"Y data in":dbl[], "X data in":dbl[]}[] [] ("Valve position vs time")
  "Is min" <- w14
  "Id min" <- w14
  "Ig min" <- w14
  "Ion vs time" <- w1
  "Ioff vs time" <- w1
  "Is on" <- w13
  "Id on" <- w13
  "Ig on" <- w13
  "Is off" <- w12
  "Id off" <- w12
  "Ig off" <- w12
  "I vs time (Bias Stress)" <- w1
